vi "SentinelController v38.vi"() -> ()   [LabVIEW 2011]
uses:
  SC MT99XX tester states.ctl
  SC handler states.ctl
  Handler Types.ctl
  SC NS6040 tester states v2.ctl
  <vilib>/Instr/_visa.llb/Select Event Type.ctl
  <userlib>/configTool/configTool.llb/initConfigGlobal.vi
  <userlib>/configTool/configTool.llb/loadConfigFile.vi
  <userlib>/configTool/configTool.llb/closeConfig.vi
  <userlib>/configTool/configTool.llb/getProperty(DBL).vi
  <userlib>/configTool/configTool.llb/getProperty(U32).vi
  <userlib>/configTool/configTool.llb/getProperty(BOOL).vi
  <userlib>/configTool/configTool.llb/getProperty(I32).vi
  <userlib>/configTool/configTool.llb/getProperty(STR).vi
panel:
  out "H2 wt start hidden":u32
  out "H2 wt end hidden":u32
  out "H2 it start hidden":u32
  out "H2 it end hidden":u32
  out "H2 tt start hidden":u32
  out "H2 tt end hidden":u32
  in  "Data log path and filename":path=path "configuraitons/default_configuraiton.cfg"
  in  "Panels":T1(tab)=enum."System Configuration"
  in  "Test cell ID":string="default"
  in  "Operator name":string="default"
  in  "Lot number":string="default"
  in  "Configuration file path and filename":path
  in  "POWER":bool=TRUE
  in  "Tester Handler Config":T2=enum."Seiko-Epson NS6040" caption="Handler type"
  in  "H1 handler type":T2=enum."Seiko-Epson NS6040" caption="Handler type"
  in  "H2 handler type":T2=enum."Seiko-Epson NS6040" caption="Handler type"
  in  "H2 allow lower parallelism":bool
  in  "H1 allow lower parallelism":bool
  in  "H1 low yield warning":dbl=95.0 min=0.0 max=100.0 step=1.0
  in  "Ignore alarms until AFTER this many cycles":i32=20
  in  "H1 low yield alarm":dbl=85.0 min=0.0 max=100.0 step=1.0
  in  "H1 low UPH warning (%)":dbl=95.0 min=1.0 max=48000.0 step=1.0
  in  "H1 low UPH alarm (%)":dbl=90.0 min=1.0 max=48000.0 step=1.0
  in  "Enable data logging of all events":bool=TRUE
  in  "Enable electronic notification of alarms":bool
  in  "H2 low UPH alarm (%)":dbl=90.0 min=1.0 max=48000.0 step=1.0
  in  "H2 low UPH warning (%)":dbl=95.0 min=1.0 max=48000.0 step=1.0
  in  "H2 low yield alarm":dbl=90.0 min=0.0 max=100.0 step=1.0
  in  "H2  low yield warning":dbl=95.0 min=0.0 max=100.0 step=1.0
  in  "H1 enable halt\non yield alarm":bool
  in  "H2 enable halt\non yield alarm":bool
  in  "H1 enable halt\non UPH alarm":bool
  in  "H2 enable halt\non UPH alarm":bool
  out "H2 Device Count":u32 caption="Device Count"
  out "H1 Device Count":u32 caption="Decvice Count"
  out "H1 Good Units":u32 caption="Decvice Count"
  out "H2 Good Units":u32 caption="Device Count"
  out "H1 lot yield mon":dbl format="%.1f"
  out "H2 lot yield mon":dbl format="%.1f"
  out "UPH averaging":u32=20 min=2 max=100 step=1
  out "Yield averaging":u32=20 min=2 max=100 step=1
  in  "Push to reset charts":bool
  in  "Run":bool caption="Run / Stop"
  in  "Optimize handler speed":bool
  out "H1 parallelism":u32
  out "Utilization averaging":i32=6 min=2 max=20 step=1
  out "H2 nominal 2":bool=TRUE
  out "H2 warning 2":bool
  out "H2 alarm 2":bool
  out "H1 nominal 2":bool=TRUE
  out "H1 warning 2":bool
  out "H1 alarm 2":bool
  out "H2 nominal":bool=TRUE
  out "H2 warning":bool
  out "H2 alarm":bool
  out "H1 nominal":bool=TRUE
  out "H1 warning":bool
  out "H1 alarm":bool
  out "H2 Lock":bool
  out "H1 Lock":bool
  out "H2 measured Test Time":dbl caption="Index Time" format="%.2f"
  out "H2 measured  Index Time":dbl caption="Index Time" format="%.2f"
  out "H2 Indexing":bool
  out "H2 Testing":bool
  out "H2 Waiting":bool
  out "H2 On/Off-line":bool
  out "H2 measured Wait Time":dbl caption="Index Time" format="%.2f"
  out "H1 measured Test Time":dbl caption="Index Time" format="%.2f"
  out "H1 measured Index Time":dbl caption="Index Time" format="%.2f"
  out "H1 Indexing":bool
  out "H1 Testing":bool
  out "H1 Waiting":bool
  out "H1 On/Off-line":bool
  out "H1 measured Wait Time":dbl caption="Index Time" format="%.2f"
  out "System UPH":u32(knob) caption="Sys UPH" scale=0.0..30240.0 scale format="%#.0f"
  out "H2 UPH":cluster{u32, u32}(knob) scale=0.0..14400.0 scale format="%#.0f"
  out "H1 UPH":cluster{u32, u32}(knob) scale=0.0..14400.0 scale format="%#.0f"
  out "Sys utilization":dbl(knob) caption="Yield" scale=0.0..100.0
  in  "H2 online":bool=TRUE
  in  "H1 online":bool=TRUE
  in  "Tester online":bool=TRUE
  in  "Alert volume":u32(knob)=5 max=10 step=1 scale=0.0..10.0
  in  "Audio On / Off":bool
  out "SysUtilMon":cluster{i32, i32}(graph)
  out "H2 parallelism":u32 caption="H2 Paralellism"
  out "YieldMon":cluster{i32, i32, i32, i32}(graph)
  out "Program Parallelism":u32=8 caption="Tester Parallelism" min=1 max=16 step=1
  out "H2 calc UPH":dbl format="%#.0f"
  out "H1 Index Time 2":dbl caption="H1 index time"
  out "H1 Test Time 2":dbl caption="H1 test time"
  out "H1 P in formula":u32 caption="H1 Parallelism"
  out "H2 UPH per unit area":dbl format="%.1f"
  out "H1 calc UPH":dbl format="%#.0f"
  out "H1 UPH per unit area":dbl format="%.1f"
  out "Std mo cost ($/mo)":dbl
  out "Std unit cost\n(cents/device)":dbl format="%.3g"
  out "UPH":dbl format="%#.0f"
  in  "Hours per month":i32=730
  out "Std hourly\ncost ($/hr)":dbl format="%.2f"
  in  "Std cell \nfloorspace area":i32=200 min=10 max=1000 step=10
  in  "Overhead ($/mo)":dbl=1000.0 min=0.0 max=10000.0 step=100.0
  in  "Handler cost ($/mo)":dbl=2500.0 min=0.0 max=100000.0 step=100.0
  in  "Tester cost ($/mo)":dbl=8500.0 min=0.0 max=100000.0 step=500.0
  in  "Utilization (%)":u32=80 min=10 max=100 step=10
  out "Calendar days required\nfor testing all units":dbl format="%.1f"
  in  "# of devices to test":u32=10000000 min=1000 max=100000000 step=1000
  out "$ saved":i64 format="%#.0f"
  out "H2 IT (scycle)":dbl format="%.2f"
  out "H2 TT (s/cycle)":dbl format="%.2f"
  out "H2 WT (s/cycle)":dbl format="%.2f"
  out "H1 WT (s/cycle)":dbl format="%.2f"
  out "H1 IT (s/cycle)":dbl format="%.2f"
  out "H1 TT (s/cycle)":dbl format="%.2f"
  out "H2 units/cycle":u32 caption="H1 Parallelism"
  out "H1 units/cycle":u32
  out "Calc H1 UPH":u32
  out "Calc H2 UPH":u32
  out "Std cell floorspace area":i32
  out "Tandem unit cost\n(cents/device)":dbl format="%.3f"
  out "Hours per month 2":i32 caption="Hours per month"
  out "Total Mo Costs ($/mo) 3":dbl caption="Tandem mo cost ($/mo)"
  out "Total Mo Costs ($/mo) 2":dbl caption="Std mo cost ($/mo)"
  out "Calc\nsystem UPH":u32 caption="Simulated\nSystem UPH"
  out "Tandem\nfloorspace area":i32
  out "Tandem UPH\nper unit area":dbl format="%.1f"
  in  "Second handler cost ($/mo)":dbl=2500.0 min=0.0 max=10000.0 step=100.0
  out "Tandem hourly\ncost ($/hr)":dbl format="%.2f"
  in  "Celerint licensing cost ($/mo)":dbl=1000.0 min=0.0 max=10000.0 step=100.0
  in  "Celerint hardware cost ($/mo)":dbl min=0.0 max=10000.0 step=1.0
  in  "Additional floorspace\nfor second handler":i32=50 min=0 max=1000 step=10
  out "Number of text alerts":u32 caption="Number of alerts\nsent as notifications"
  in  "Enable text notification":bool
  out "Notifications Lot Display":string="default" caption="Lot number (not editable)"
  in  "Include\ndata log as\nattachment":bool=TRUE
  out "Number of email alerts":u32 caption="Number of alerts\nsent as notifications"
  out "Email alert - attachment (not editable)":path
  in  "Email alert - message":string="An alarm event has ocurred on a semiconductor test lot that you have requested to monitor.  Please see the attached data log for event details.\n\nThis message is generated automatically by the Sentinel Controller program.\n\nTo stop these messages, please contact the test floor operator and disable automatic alert notifictions.\n\n"
  in  "Email alert - engineer":string="harry@celerint.com"
  in  "Email alert - CC":string="hjr@celerint.com"
  in  "Enable email notification":bool
  in  "Carrier":enum16{"T-Mobile", "AT&T", "Verizon", "Sprint"}(ring)=enum."AT&T"
  in  "Phone number":string="5128263411"
  in  "Subject":string="From: Sentinel Controller"
  in  "Body":string="An alarm event has ocurred"
  in  "GPIB wait time (ms)":u32=1000
  in  "Slow for  Diagnostics":bool=TRUE
  out "GPIB bus 0 read error":bool
  out "GPIB Bus 0 traffic":string
  out "GPIB bus 1 traffic":string
  out "GPIB bus 2 traffic":string
  out "GPIB bus 0 write error":bool
  out "GPIB bus 1 read error":bool
  out "GPIB bus 1 write error":bool
  out "GPIB bus 2 write error":bool
  out "GPIB bus 2 read error":bool
  out "VISA bus 1 open error":bool
  out "VISA bus 2 open error":bool
  out "VISA bus 0 open error":bool
  out "VISA bus 0 close error":bool
  out "VISA bus 1 close error":bool
  out "VISA bus 2 close error":bool
  out "Decrease Handler Velocity":string
  out "Increase Handler Velocity":string
  out "Get Handler Velocity":string
  in  "SentCtrl listens to tester at":refnum<visa-resource-name>="GPIB0::INTFC"
  out "H2 Address":string
  out "H1 Address":string
  out "Tester address":string
  in  "SentCtrl talks to tester at":refnum<visa-resource-name>="GPIB0::0::INSTR"
  in  "SentCtrl listens to handler 1 at":refnum<visa-resource-name>="GPIB1::INTFC"
  in  "SentCtrl talks to handler 1 at":refnum<visa-resource-name>="GPIB1::1::INSTR"
  in  "SentCtrl listens to handler 2 at":refnum<visa-resource-name>="GPIB2::INTFC"
  in  "SentCtrl talks to handler 2 at":refnum<visa-resource-name>="GPIB2::1::INSTR"
  in  "Ni Logo":bool
  in  "Ni Logo 2":bool
  in  "H2 Ready with sites hid":bool
  in  "SRQ MASK from tester hid":string
  in  "H1 binning string hid":string
  in  "H2 binning string hid":string
  in  "H1 FULLSITES? response hid":string
  in  "H2 FULLSITES? response hid":string
  in  "H1 FULLSITES? binary hid":string
  in  "H2 FULLSITES? binary hid":string
  in  "H1 response to SPOLL hid":string
  in  "H2 response to SPOLL hid":string
  in  "H1 response to FR? hid":string
  in  "H2 response to FR? hid":string
  in  "NS6040 tester states H1 hid":T3
  in  "NS6040 tester states H2 hid":T3
  in  "MT99XX tester states H2 hid":T4
  in  "MT99XX tester states H1 hid":T4
  in  "GPIB parsed msg from tester hid":string
  in  "Message from H2 hid":string
  in  "Message from H1 hid":string
  in  "Message from tester hid":string
  in  "H1 response to *IDN? hid":string
  in  "H2 response to *IDN? hid":string
  in  "GPIB wait timeout hid":u32
  out "Number of data log entries hid":u32
  in  "Last locked handler hid":enum16{"H1", "H2"}(ring)
  out "SC measured wait time hid":dbl
  out "Exit SC tester H2 StMach hid":bool
  out "Exit SC tester H1 StMach hid":bool
  out "Exit SC handler StMach hid":bool
  out "H2 response to *HAND? hid":string
  out "H1 response to *HAND? hid":string
  in  "Tester loop counter hid":u32
  in  "H2 loop counter hid":u32
  in  "H1 loop counter hid":u32
  in  "Test Cycle State hid":T5(ring)
  in  "Test time expected hid":dbl
  out "H1 it end hidden":u32
  out "H1 wt start hidden":u32
  out "H1 tt start hidden":u32
  out "H1 wt end hidden":u32
  out "H1 tt end hidden":u32
  out "H1 it start hidden":u32
  in  "H1 SITES? response hid":string
  out "VISA bus 1 resource name out hid":refnum<visa-resource-name>
  out "VISA bus 1 error out hid":errorcluster
  out "VISA bus 2 error out hid":errorcluster
  out "VISA bus 2 resource name out hid":refnum<visa-resource-name>
  out "VISA bus 0 error out hid":errorcluster
  out "tester wt start hid":u32
  out "tester wt end hid":u32
  out "tester tt start hid":u32
  out "tester tt end hid":u32
  out "SC measured test time hid":dbl
  in  "Binning string from tester hid":string
  out "VISA bus 0 resource name out hid":refnum<visa-resource-name>
  in  "SC handler states hid":T6
  out "H1 Single Handler UPH hid":dbl
  out "H1 UPH warning limit hid":dbl
  out "H1 UPH alarm limit hid":dbl
  out "H2 Single Handler UPH hid":dbl
  out "H2 UPH warning limit hid":dbl
  out "H2 UPH alarm limit hid":dbl
  in  "Min Test Time hid":dbl=0.499 caption="Min Test Time" min=0.1 max=1.0 step=0.1 format="%#.1g"
  in  "H2 index time expected hid":dbl
  in  "H1 index time expected hid":dbl
  in  "system states hid":T7(ring)
  in  "system statuts hid":T8(ring)
  out "H1 cycle yield hid":dbl format="%.1f"
  out "H2 cycle yield hid":dbl format="%.1f"
  in  "H2 SITES? response hid":string
  in  "H1 Ready with sites hid":bool
  # "Sentinel Controller\nfor\nTandlem Handler\nTest Cells \nwww.celerint.com"
  # "Turning off POWER will stop execution the Sentinel Controller Program"
  # "INPUT FILE"
  # "LOT INFORMATION"
  # "Celerint Sentinel Controller"
  # "SYSTEM SETTINGS"
  # "Tester Handler Config"
  # "Handler  1"
  # "Handler 2"
  # "Set UPH thresholds as % of max UPH"
  # "Set UPH thresholds as % of max UPH"
  # "test cycles (insertions)"
  # "Celerint Sentinel Controller"
  # "Handler 2"
  # "Handler 1"
  # "Yield"
  # "UPH"
  # "Yield"
  # "UPH"
  # "parallelism"
  # "lot yield (%)"
  # "good devices"
  # "devices tested"
  # "Data"
  # "Avg"
  # "wait time"
  # "index time"
  # "test time"
  # "waiting"
  # "H1"
  # "H2"
  # "testing"
  # "indexing"
  # "on/off-line"
  # "STANDARD SETUP"
  # "H2 calculated\nsimilarly"
  # "3600"
  # "Celerint Sentinel\nController Simulator"
  # "TANDEM HANDLER SETUP"
  # "SAVINGS"
  # "3600 (s/hr)"
  # "3600 (s/hr)"
  # "Celerint Sentinel Controller"
  # "Lot number will be appended automatically:"
  # "This data is read from the INI file (.cfg)\nat program start and is used to configure\nthe various GPIB interfaces on the Sentinel\nController."
  # "These setting are created based on the addresses read from the INI file."
  # "Laptop Tester Sim\nGPIB0,SC\naddress 0\nlisten at: GPIB0::INTFC\ntalk to: GPIB0::1::INSTR"
  # "*SITES?"
  # "binning"
  # "Bus 0"
  # "1011"
  # "SC\nGPIB0,Non-SC\naddress 1\nlisten at: GPIB0::INTFC\ntalk to: GPIB0::0::INSTR"
  # "SC\nGPIB1,SC\naddress 0\nlisten at: GPIB1::INTFC\ntalk to: GPIB1::0::INSTR"
  # "SC\nGPIB2,SC\naddress 0\nlisten at: GPIB2::INTFC\ntalk to: GPIB2::0::INSTR"
  # "NI PXI-1031"
  # "*SITES?"
  # "binning"
  # "*SITES?"
  # "binning"
  # "Bus 1"
  # "Bus 2"
  # "1011"
  # "1011"
  # "Laptop H1 Sim\nGPIB1,Non-SC\naddress 1\nlisten at: GPIB1::INTFC\ntalk to: GPIB1::0::INSTR"
  # "Laptop H2 Sim\nGPIB2,Non-SC\naddress 1\nlisten at: GPIB2::INTFC\ntalk to: GPIB2::0::INSTR"
  # "Note:\nUsually, there are default GPIB addresses used for the tester and handler.\nThese addresses are read in from the INI file (.cfrg extension) when this\nprogram initializes.  For the purposes of this map, we are using  these defaults:\n          - Semiconductor tester default GPIB address: 6\n          - Semiconductor handler default GPIB address: 14\nFor the purposes of this illustration, these addresses are purely arbitrary."
  # "Tester\nGPIB0,SC\naddress 6\nlisten at: GPIB0::INTFC\ntalk to: GPIB0:14::INSTR"
  # "*SITES?"
  # "binning"
  # "Bus 0"
  # "1011"
  # "SC\nGPIB0,Non-SC\naddress 14\nlisten at: GPIB1::INTFC\ntalk to: GPIB1:6::INSTR"
  # "SC\nGPIB1,SC\naddress 6\nlisten at: GPIB1::INTFC\ntalk to: GPIB1:14::INSTR"
  # "SC\nGPIB2,SC\naddress 6\nlisten at: GPIB2::INTFC\ntalk to: GPIB2:14::INSTR"
  # "NI PXI-1031"
  # "*SITES?"
  # "binning"
  # "*SITES?"
  # "binning"
  # "Bus 1"
  # "Bus 2"
  # "1011"
  # "1011"
  # "Handler 1\nGPIB0,Non-SC\naddress 14\nlisten at: GPIB0::INTFC\ntalk to: GPIB0:6::INSTR"
  # "Handler 2\nGPIB0,Non-SC\naddress 14\nlisten at: GPIB0::INTFC\ntalk to: GPIB0:6::INSTR"
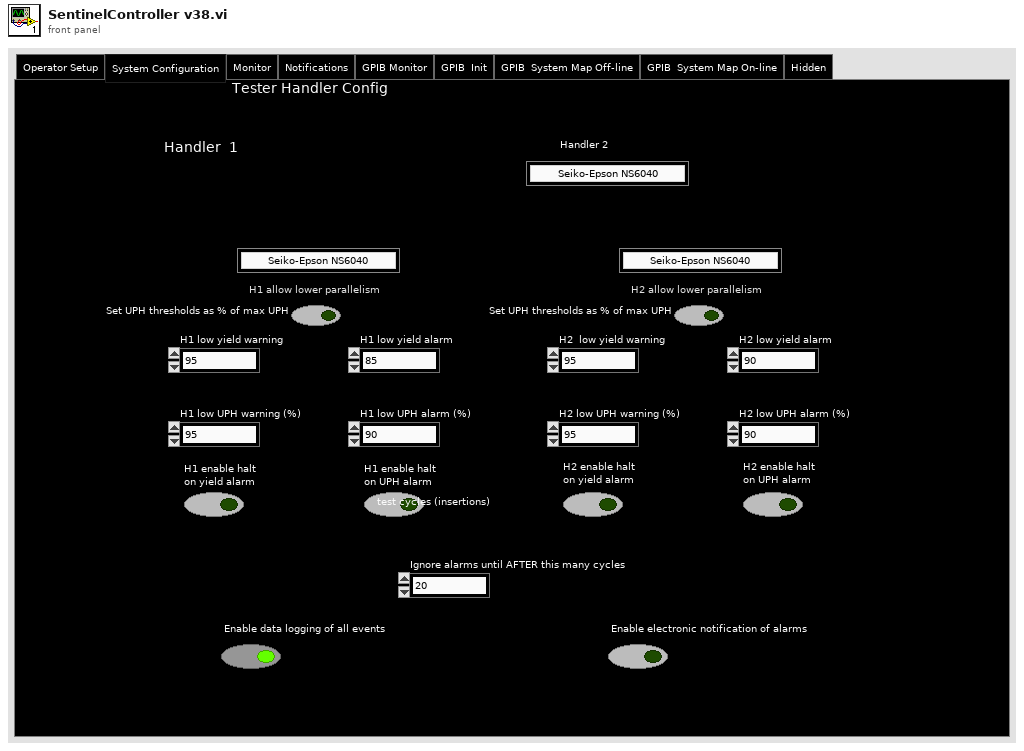
[diagram p1: front panel]
types:
  T1 = enum32{"Operator Setup", "System Configuration", "Monitor", "Benefit Analysis", "Notifications", "GPIB Monitor", "GPIB  Init", "GPIB  System Map Off-line", "GPIB  System Map On-line", "Hidden"}
  T2 = typedef "Handler Types.ctl" = enum16{"Multitest", "Seiko-Epson NS6040"}
  T3 = typedef "SC NS6040 tester states v2.ctl" = enum16{"initializing bus", "sending *IDN?", "serial polling handler", "sending Fullsites?", "testing", "binning", "closing bus"}
  T4 = typedef "SC MT99XX tester states.ctl" = enum16{"initializing bus", "polling *SITES?", "sending *IDN?", "testing", "binning", "closing bus"}
  T5 = enum16{"idled", "SOT received", "SOT sent", "binning sent", "binning received", "sites ready received", "sites ready sent"}
  T6 = typedef "SC handler states.ctl" = enum16{"initializing bus", "waiting on event", "waiting on serial poll", "reading", "responding to *IDN?", "responding to Fullsites?", "responding to SITES?", "responding to HIDN?", "respond to HAND?", "testing", "responding to BINON", "responding to A BIN", "ECHONG", "ECHOOK", "responding to unknown command", "closing bus"}
  T7 = enum16{"H1 Ready", "H2 Ready", "No Handler Ready"}
  T8 = enum16{"H1NH2N", "H1NH2W", "H1NH2A", "H1WH2N", "H1WH2W", "H1WH2A", "H1AH2N", "H1AH2W", "H1AH2A"}
  T9 = enum16{"open", "replace", "create", "open or create", "replace or create", "replace or create with confirmation"}
  T10 = typedef "configRef.ctl" = refnum<vi>
  T11 = cluster{i32, "rolling avg out":dbl, "H1 low yield alarm":dbl, "H2 low yield alarm":dbl}
  T12 = cluster{"rolling avg out":dbl, i32, "H1 low yield alarm":dbl, "H2 low yield alarm":dbl}
  T13 = typedef "Select Event Type.ctl" = u32
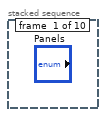
[diagram p2: hidden frame]
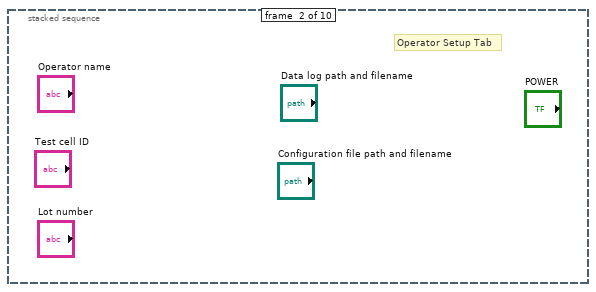
[diagram p3: hidden frame]
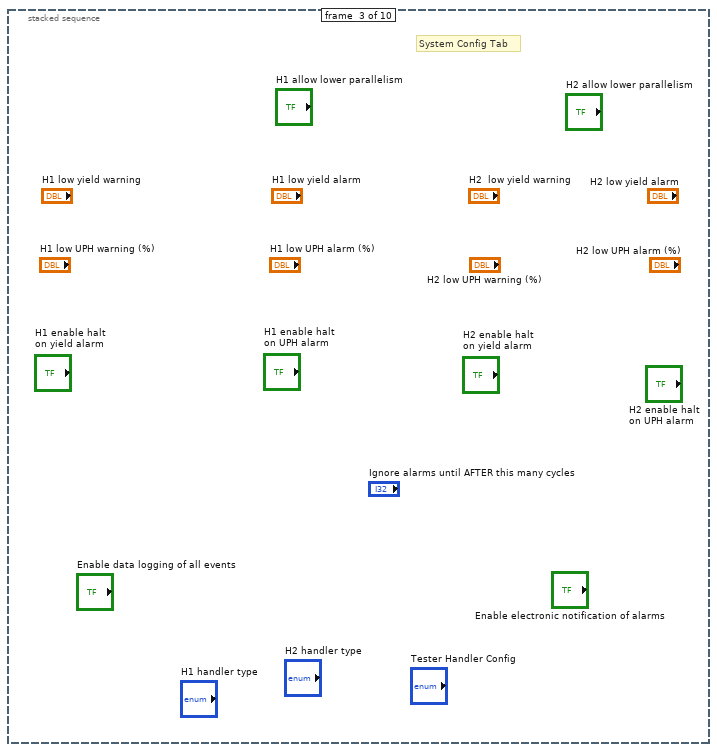
[diagram p4: hidden frame]
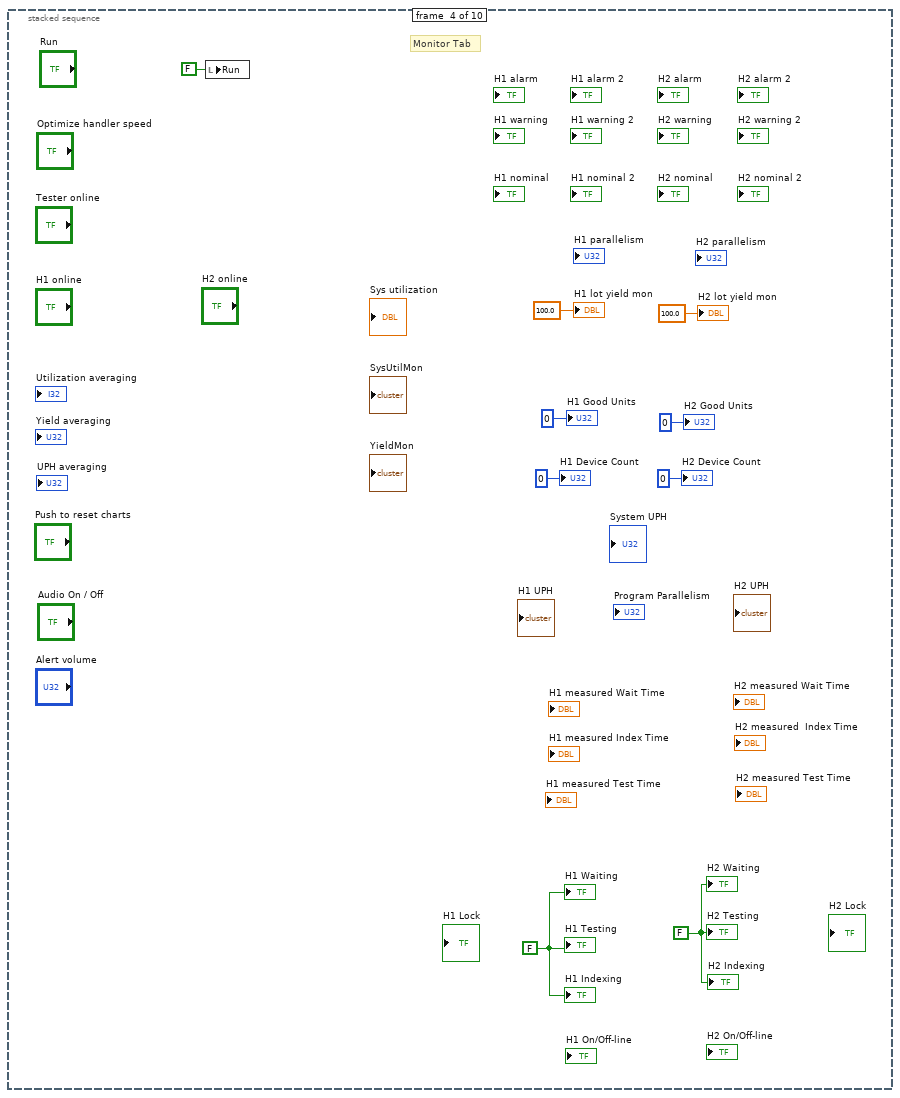
[diagram p5: hidden frame]
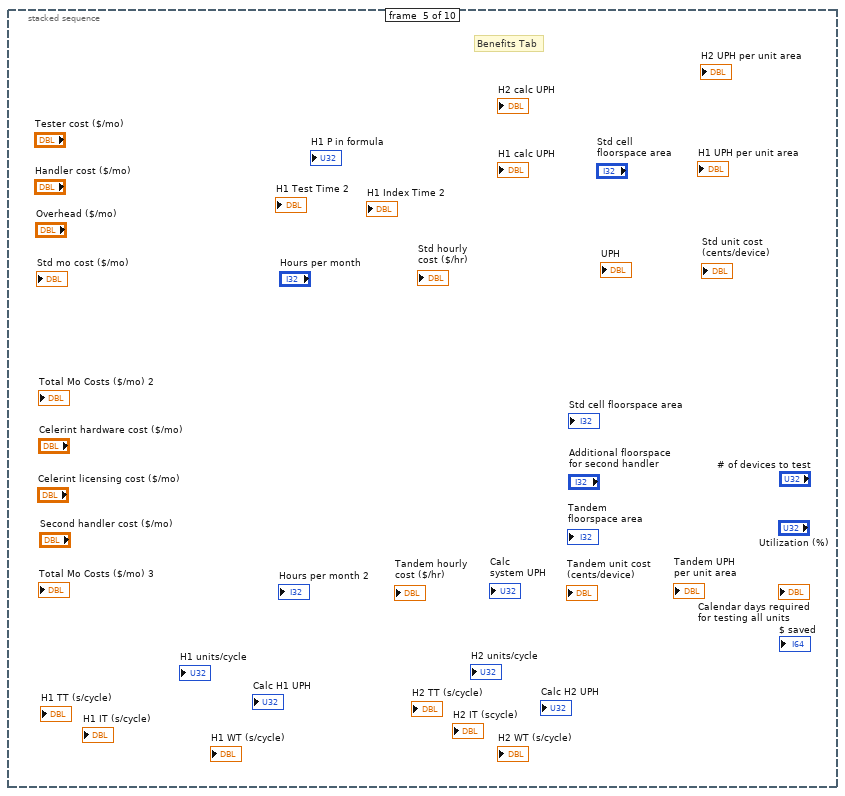
[diagram p6: hidden frame]
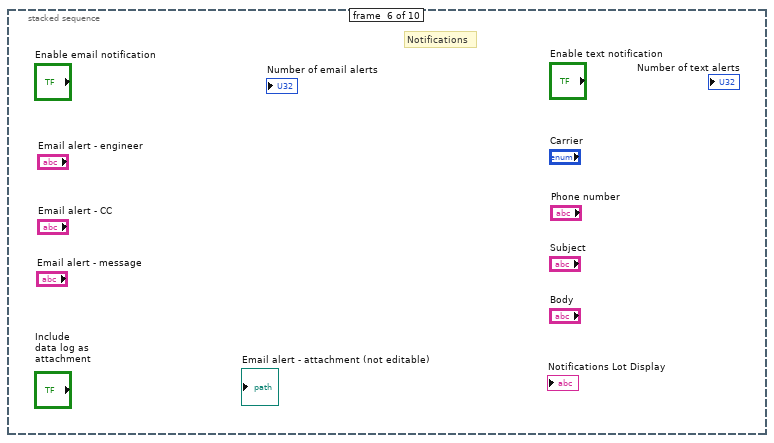
[diagram p7: hidden frame]
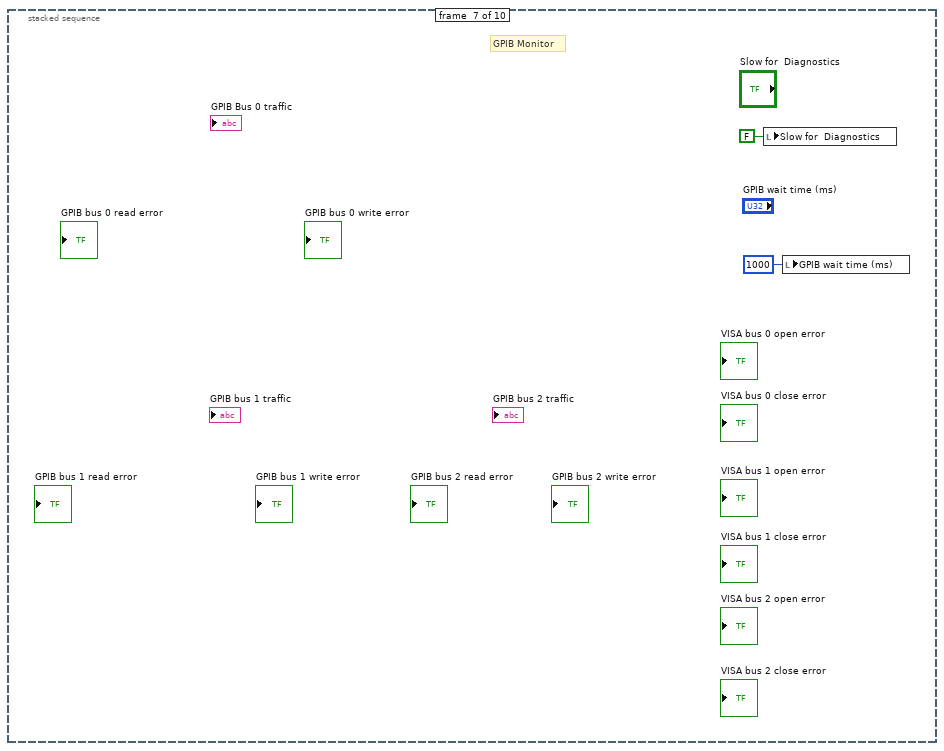
[diagram p8: hidden frame]
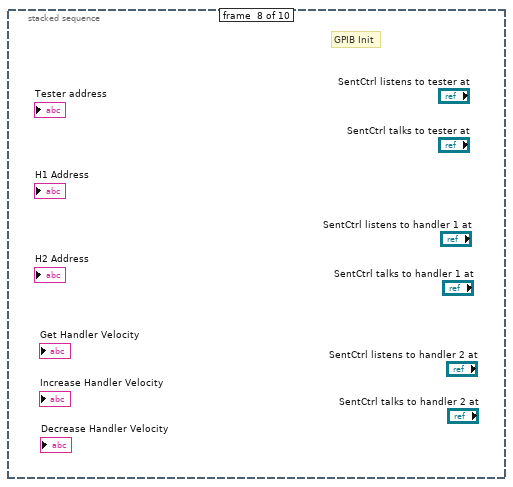
[diagram p9: hidden frame]
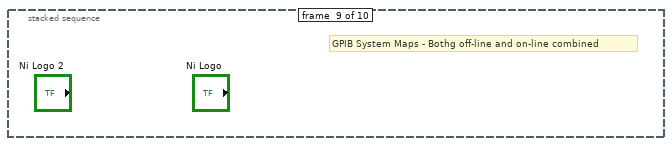
[diagram p10: hidden frame]
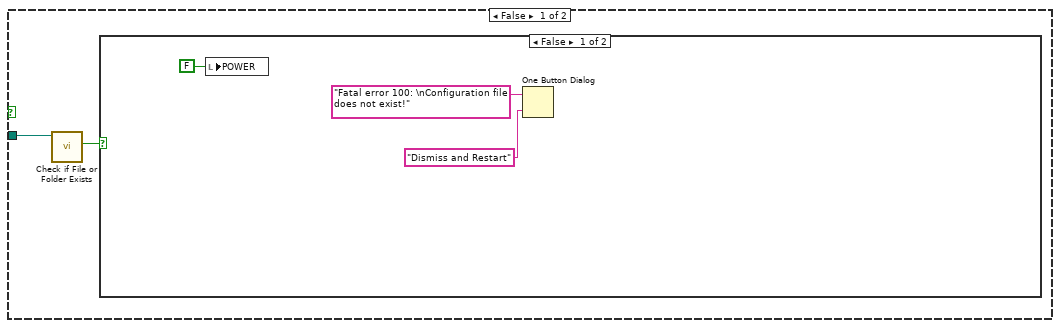
[diagram p11: hidden frame]
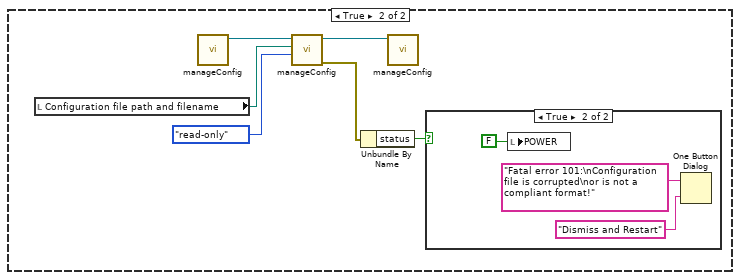
[diagram p12: hidden frame]
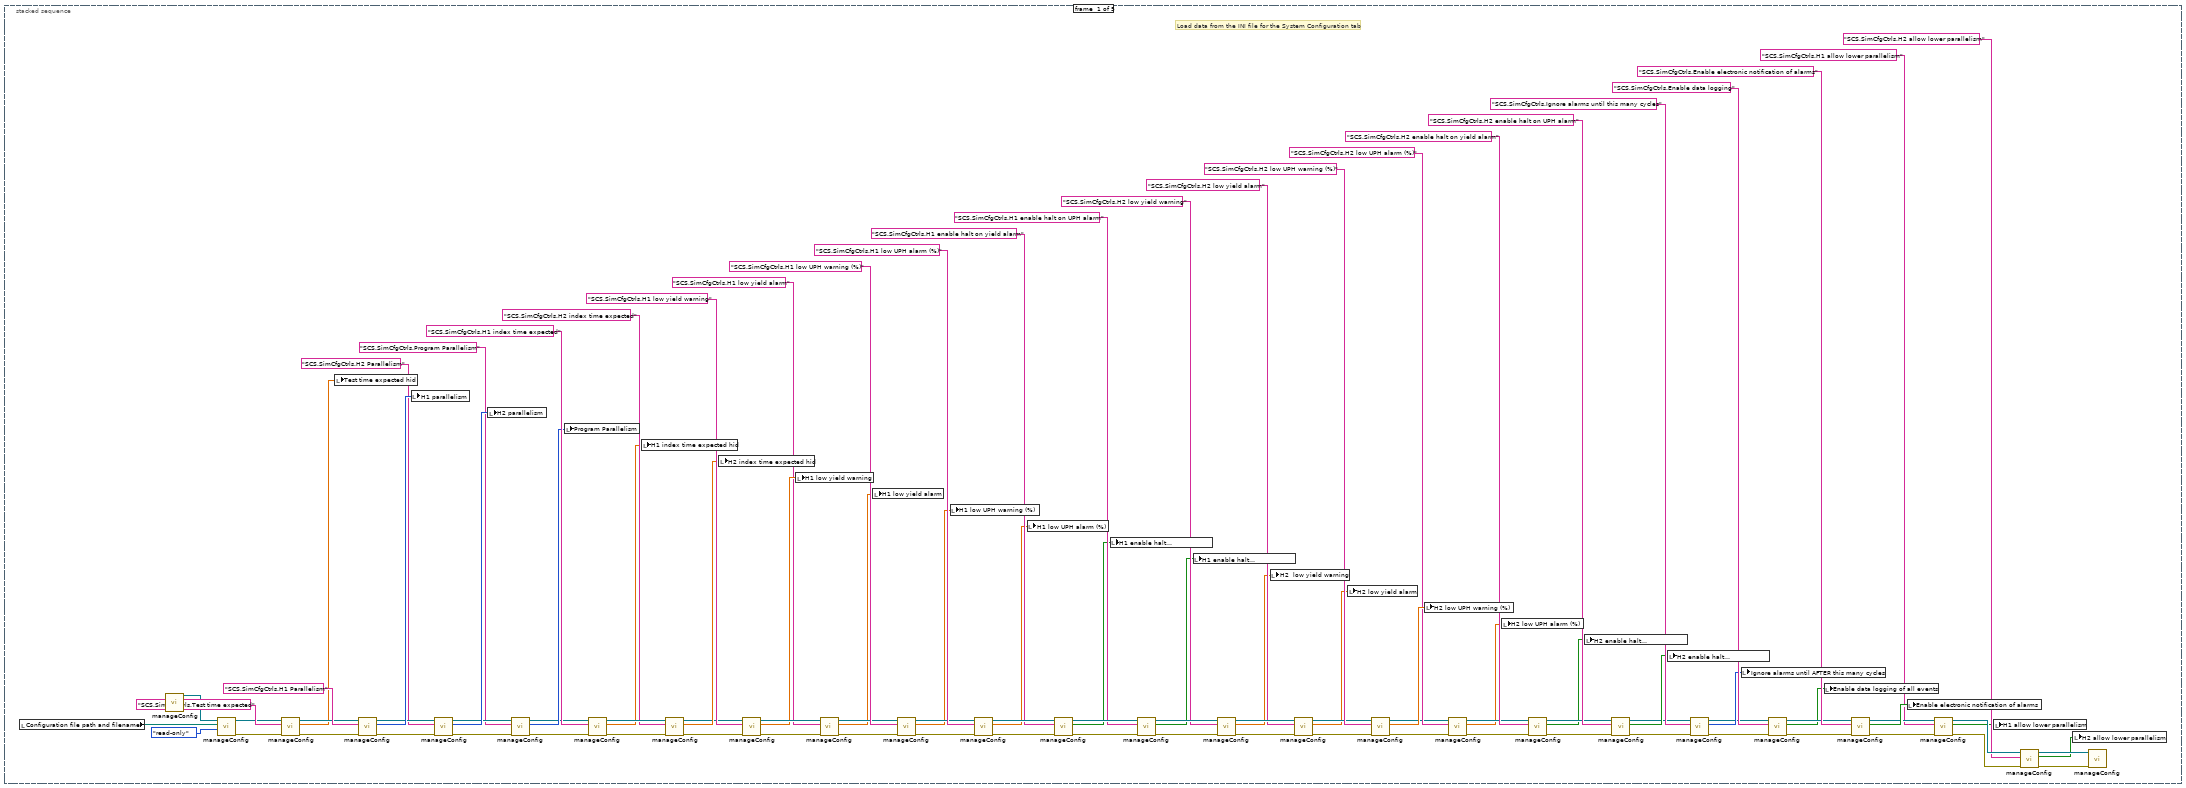
[diagram p15: hidden frame]
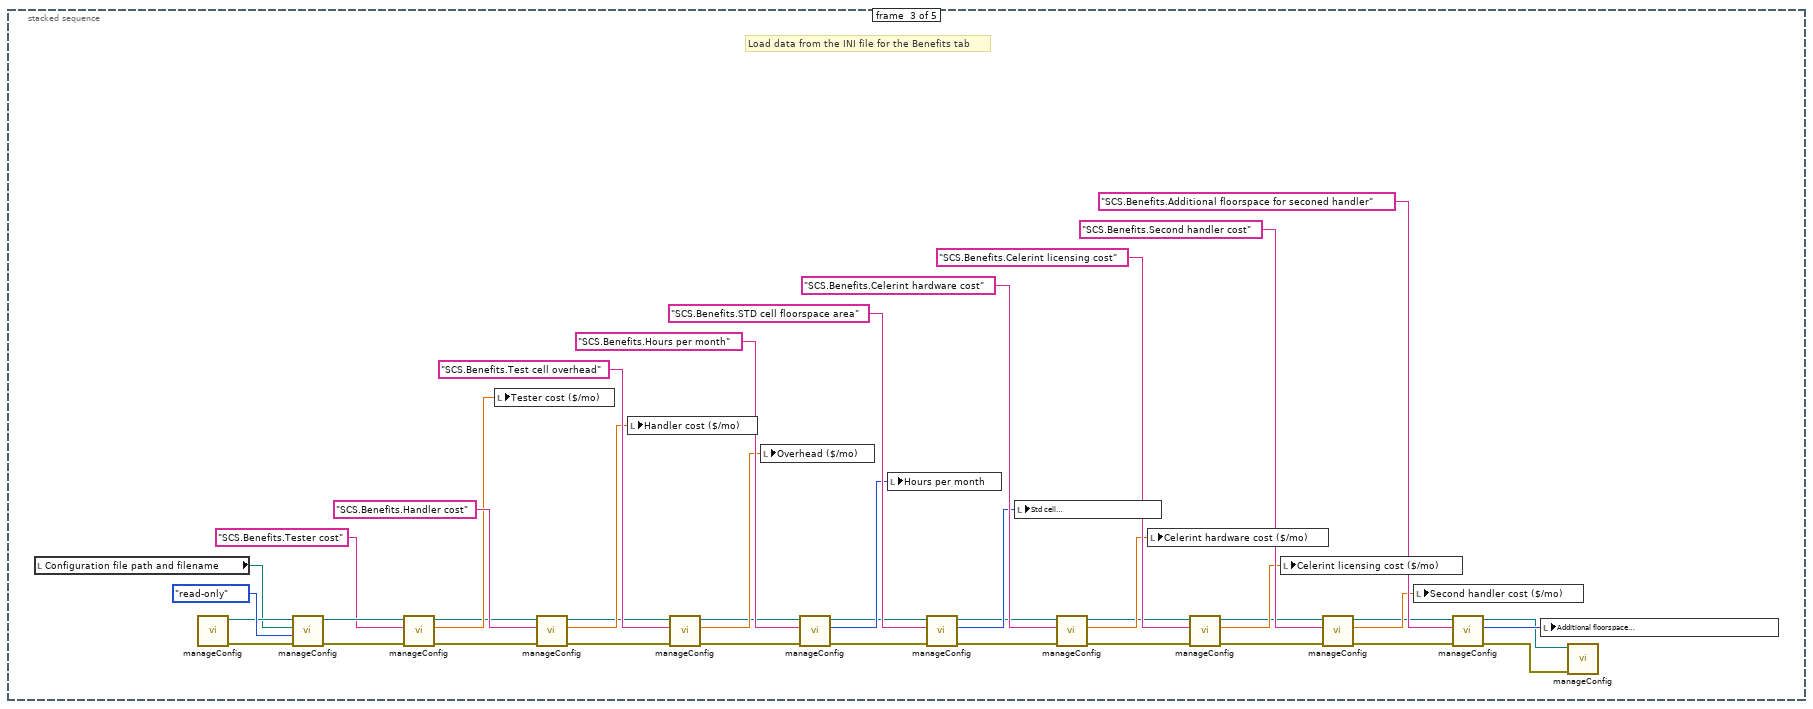
[diagram p16: hidden frame]
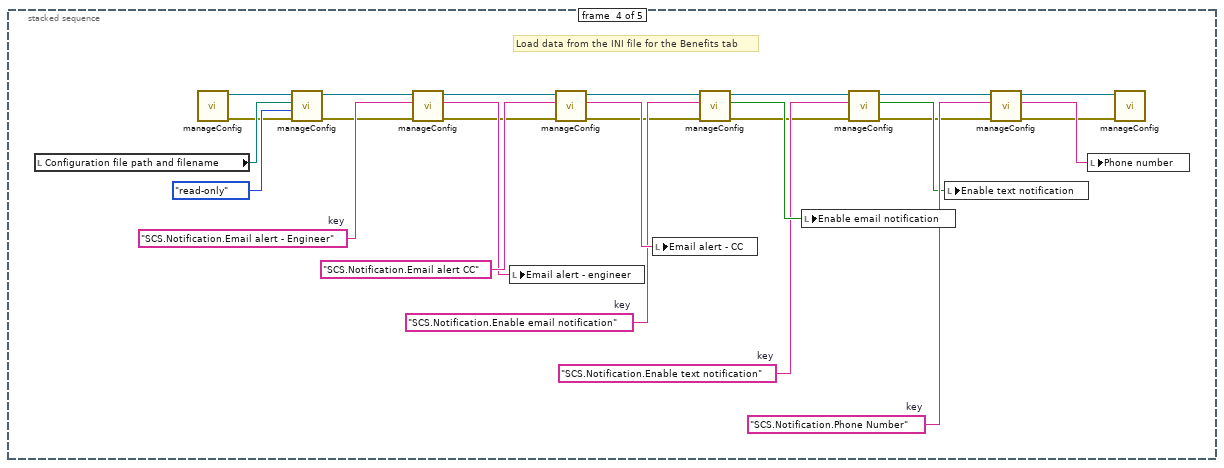
[diagram p17: hidden frame]
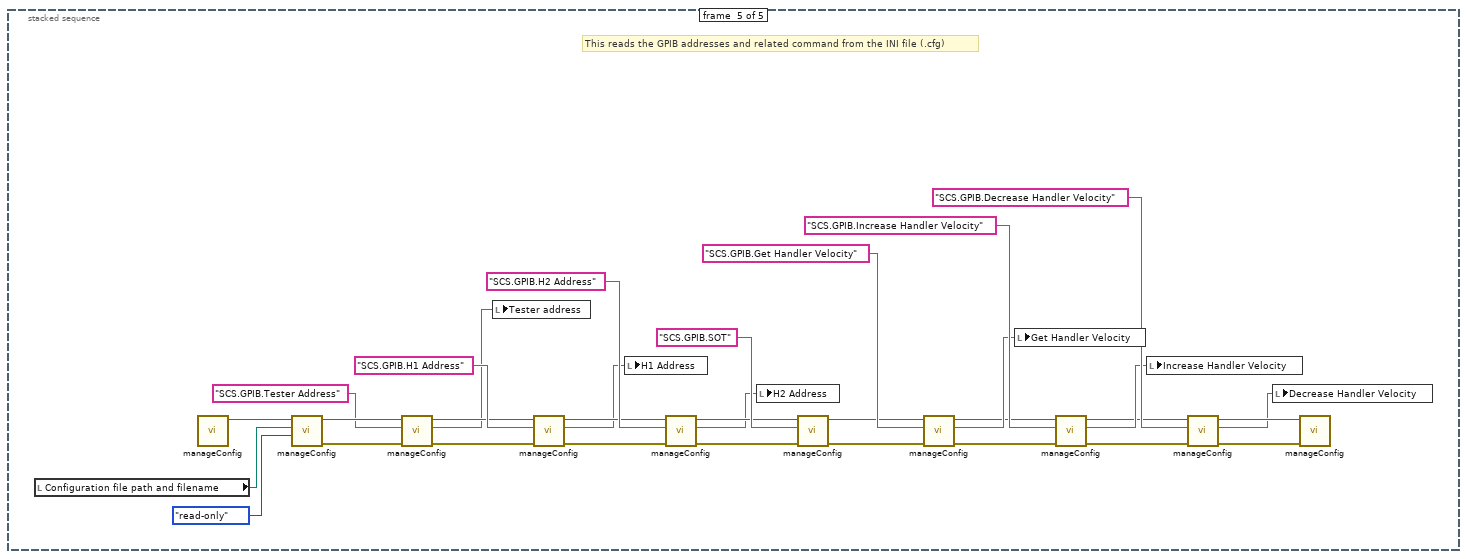
[diagram p18: hidden frame]
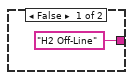
[diagram p20: hidden frame]
diagram:
  n1 = flat-sequence {
    frame #0 {
      # "This frame contains ALL declarations for control and indicators.\nAll hidden objects are on frame #9.  On the front panel, these hidden\nobjects are located on a tab that is hidden."
      n2 = stacked-sequence {
        frame #0 {
        }
        frame #1 {
          # "Operator Setup Tab"
        }
        frame #2 {
          # "System Config Tab"
        }
        frame #3 {
          w2 = FALSE ("H2 Testing")
          w1 = FALSE ("H1 Testing")
          # "Monitor Tab"
          n3 = local write "Run"(FALSE ("Run")) -> ()
          "H1 Testing" <- w1
          "H1 Waiting" <- w1
          "H1 Indexing" <- w1
          "H2 Testing" <- w2
          "H2 Waiting" <- w2
          "H2 Indexing" <- w2
          "H2 Good Units" <- 0
          "H2 Device Count" <- 0
          "H2 lot yield mon" <- 100.0 ("H2 Yield  Mon")
          "H1 lot yield mon" <- 100.0 ("H1 Yield Mon")
          "H1 Good Units" <- u32 0
          "H1 Device Count" <- u32 0
        }
        frame #4 {
          # "Benefits Tab"
        }
        frame #5 {
          # "Notifications"
        }
        frame #6 {
          # "GPIB Monitor"
          n4 = local write "Slow for  Diagnostics"(FALSE ("Slow for  Diagnostics")) -> ()
          n5 = local write "GPIB wait time (ms)"(u32 1000 ("GPIB wait time (ms)")) -> ()
        }
        frame #7 {
          # "GPIB Init"
        }
        frame #8 {
          # "GPIB System Maps - Bothg off-line and on-line combined"
        }
        frame #9 {
          (unwired) 0.031 ("tester measured wait time")
          # "Hidden controls and indicators"
          n6 = local write "Last locked handler hid"(enum16{"H1", "H2"}."H1" ("Last locked handler")) -> ()
          "SC measured test time hid" <- 1.0 ("tester measured test time")
          "H1 response to *HAND? hid" <- "" ("H1 response to *HAND? hidden")
          "H2 response to *HAND? hid" <- "" ("H2 response to *HAND? hidden")
          "Exit SC handler StMach hid" <- FALSE ("Exit tester state machine")
          "Exit SC tester H1 StMach hid" <- FALSE ("Exit H1 state machine")
          "Exit SC tester H2 StMach hid" <- FALSE ("Exit H2 state machine")
          "SC measured wait time hid" <- 1.0 ("tester measured wait time hid")
          "H2 cycle yield hid" <- 100.0 ("H2 Yield  Mon")
          "H1 cycle yield hid" <- 100.0 ("H1 Yield Mon")
        }
      }
    }
    frame #1 {
      n7 = local write "POWER"(TRUE ("POWER")) -> ()
    }
    frame #2 {
      # "This frame handles verifying that the configuration file exists and is valaid.\nIt also creates the data log."
      n8 = local read "Configuration file path and filename"() -> (w25:path)
      n9 = call <vilib>:"Application Directory.vi"() -> ("Application Directory"=w27:path)
      n10 = Equal?(x=w25, y=path "") -> (x = y?=w24:bool)
      n11 = Get Date/Time String(want seconds? (F)=TRUE) -> (date string=w40:string, time string=w32:string)  [unwired: 2 in]
      n12 = Build Path(base path=w27, name or relative path="datalogs") -> (appended path=w45:path)
      n13 = Path To String(path=w45) -> (string=w36:string)
      n14 = Search and Replace String(replace all?=TRUE ("replace all? (F)"), input string=w40, search string="/", replace string="-" ("replace string (\"\")")) -> (result string=w30:string)  [unwired: 4 in, 3 out]
      n15 = Search and Replace String(replace all?=TRUE ("replace all? (F)"), input string=w32, search string=":", replace string="." ("replace string (\"\")")) -> (result string=w31:string)  [unwired: 4 in, 3 out]
      n16 = case shown="True" w24 {
        tunnel: w25 -> [w47 _]
        frame False {
          n17 = call <vilib>:"Check if File or Folder Exists.vi"("path"=w47) -> ("file or folder exists?"=w46:bool)  [unwired: 8 in, 2 out]
          n18 = case shown="False" w46 {
            frame False {
              n19 = local write "POWER"(FALSE ("POWER")) -> ()
              n20 = One Button Dialog(message="Fatal error 100: \nConfiguration file does not exist!", button name ("OK")="Dismiss and Restart") -> ()  [unwired: 1 out]
            }
            frame True {
              n21 = local read "Configuration file path and filename"() -> (w54:path)
              n22 = call-poly <userlib>:"manageConfig.vi"() -> ("config ref out"=w55:T10)  [unwired: 10 in, 1 out]
              n23 = call-poly <userlib>:"manageConfig.vi"("access (0:read/write)"=enum16{"read/write", "read-only", "write-only"}."read-only", "config file path"=w54, "config ref"=w55) -> ("error out"=w53:errorcluster, "config ref out"=w51:T10)  [unwired: 6 in, 1 out]
              n24 = Unbundle By Name(w53) -> ("status"=w52:bool)
              n25 = call-poly <userlib>:"manageConfig.vi"("config ref"=w51) -> ()  [unwired: 10 in, 1 out]
              n26 = case shown="True" w52 {
                frame False {
                }
                frame True {
                  n27 = local write "POWER"(FALSE ("POWER")) -> ()
                  n28 = One Button Dialog(message="Fatal error 101:\nConfiguration file is corrupted\nor is not a compliant format!", button name ("OK")="Dismiss and Restart") -> ()  [unwired: 1 out]
                }
              }
            }
          }
        }
        frame True {
          n29 = call <vilib>:"Application Directory.vi"() -> ("Application Directory"=w63:path)
          n30 = Build Path(base path=w63, name or relative path="configurations") -> (appended path=w60:path)
          n31 = Path To String(path=w60) -> (string=w65:string)
          n32 = Concatenate Strings(w65, "\\" ("string"), "default_configuration.cfg" ("string")) -> (w66:string)
          n33 = String To Path(string=w66) -> (path=w67:path)
          n34 = local write "Configuration file path and filename"(w67) -> ()
        }
      }
      n35 = Concatenate Strings(w36, "\\" ("string"), w30, " " ("string"), w31, ".txt" ("string")) -> (w42:string)
      n36 = String To Path(string=w42) -> (path=w44:path)
      n37 = local write "Data log path and filename"(w44) -> ()
    }
    frame #3 {
      # "This frame reads the INI file and initializes all data that is under engineering control."
      n38 = local read "POWER"() -> (w68:bool)
      n39 = case shown="True" w68 {
        frame False {
        }
        frame True {
          n40 = stacked-sequence {
            frame #0 {
              # "Load data from the INI file for the System Configuration tab"
              n41 = local read "Configuration file path and filename"() -> (w162:path)
              n42 = call-poly <userlib>:"manageConfig.vi"() -> ("config ref out"=w163:T10)  [unwired: 10 in, 1 out]
              n43 = call-poly <userlib>:"manageConfig.vi"("access (0:read/write)"=enum16{"read/write", "read-only", "write-only"}."read-only", "config file path"=w162, "config ref"=w163) -> ("error out"=w101:errorcluster, "config ref out"=w100:T10)  [unwired: 6 in, 1 out]
              n44 = call-poly <userlib>:"manageConfig.vi"("error in"=w101, "property path"="SCS.SimCfgCtrls.Test time expected" ("key"), "config ref"=w100) -> ("error out"=w97:errorcluster, "data"=w103:dbl, "config ref out"=w104:T10)  [unwired: 5 in, 1 out]
              n45 = local write "Test time expected hid"(w103) -> ()
              n46 = call-poly <userlib>:"manageConfig.vi"("error in"=w97, "property path"="SCS.SimCfgCtrls.H1 Parallelism", "config ref"=w104) -> ("error out"=w96:errorcluster, "value"=w116:u32, "config ref out"=w110:T10)  [unwired: 5 in, 1 out]
              n47 = local write "H1 parallelism"(w116) -> ()
              n48 = call-poly <userlib>:"manageConfig.vi"("error in"=w96, "property path"="SCS.SimCfgCtrls.H2 Parallelism", "config ref"=w110) -> ("error out"=w95:errorcluster, "value"=w112:u32, "config ref out"=w109:T10)  [unwired: 5 in, 1 out]
              n49 = local write "H2 parallelism"(w112) -> ()
              n50 = call-poly <userlib>:"manageConfig.vi"("error in"=w95, "property path"="SCS.SimCfgCtrls.Program Parallelism", "config ref"=w109) -> ("error out"=w94:errorcluster, "value"=w111:u32, "config ref out"=w102:T10)  [unwired: 5 in, 1 out]
              n51 = local write "Program Parallelism"(w111) -> ()
              n52 = call-poly <userlib>:"manageConfig.vi"("error in"=w94, "property path"="SCS.SimCfgCtrls.H1 index time expected", "config ref"=w102) -> ("error out"=w93:errorcluster, "data"=w106:dbl, "config ref out"=w115:T10)  [unwired: 5 in, 1 out]
              n53 = local write "H1 index time expected hid"(w106) -> ()
              n54 = call-poly <userlib>:"manageConfig.vi"("error in"=w93, "property path"="SCS.SimCfgCtrls.H2 index time expected", "config ref"=w115) -> ("error out"=w99:errorcluster, "data"=w105:dbl, "config ref out"=w98:T10)  [unwired: 5 in, 1 out]
              n55 = local write "H2 index time expected hid"(w105) -> ()
              n56 = call-poly <userlib>:"manageConfig.vi"("error in"=w99, "property path"="SCS.SimCfgCtrls.H1 low yield warning" ("key"), "config ref"=w98) -> ("error out"=w92:errorcluster, "data"=w139:dbl, "config ref out"=w149:T10)  [unwired: 5 in, 1 out]
              n57 = local write "H1 low yield warning"(w139) -> ()
              n58 = call-poly <userlib>:"manageConfig.vi"("error in"=w92, "property path"="SCS.SimCfgCtrls.H1 low yield alarm", "config ref"=w149) -> ("error out"=w91:errorcluster, "data"=w138:dbl, "config ref out"=w148:T10)  [unwired: 5 in, 1 out]
              n59 = local write "H1 low yield alarm"(w138) -> ()
              n60 = call-poly <userlib>:"manageConfig.vi"("error in"=w91, "property path"="SCS.SimCfgCtrls.H1 low UPH warning (%)", "config ref"=w148) -> ("error out"=w90:errorcluster, "data"=w137:dbl, "config ref out"=w150:T10)  [unwired: 5 in, 1 out]
              n61 = local write "H1 low UPH warning (%)"(w137) -> ()
              n62 = call-poly <userlib>:"manageConfig.vi"("error in"=w90, "property path"="SCS.SimCfgCtrls.H1 low UPH alarm (%)", "config ref"=w150) -> ("error out"=w89:errorcluster, "data"=w136:dbl, "config ref out"=w151:T10)  [unwired: 5 in, 1 out]
              n63 = local write "H1 low UPH alarm (%)"(w136) -> ()
              n64 = call-poly <userlib>:"manageConfig.vi"("error in"=w89, "property path"="SCS.SimCfgCtrls.H1 enable halt on yield alarm", "config ref"=w151) -> ("error out"=w88:errorcluster, "value"=w135:bool, "config ref out"=w152:T10)  [unwired: 5 in, 1 out]
              n65 = local write "H1 enable halt\non yield alarm"(w135) -> ()
              n66 = call-poly <userlib>:"manageConfig.vi"("error in"=w88, "property path"="SCS.SimCfgCtrls.H1 enable halt on UPH alarm", "config ref"=w152) -> ("error out"=w87:errorcluster, "value"=w134:bool, "config ref out"=w153:T10)  [unwired: 5 in, 1 out]
              n67 = local write "H1 enable halt\non UPH alarm"(w134) -> ()
              n68 = call-poly <userlib>:"manageConfig.vi"("error in"=w87, "property path"="SCS.SimCfgCtrls.H2 low yield warning", "config ref"=w153) -> ("error out"=w86:errorcluster, "data"=w133:dbl, "config ref out"=w154:T10)  [unwired: 5 in, 1 out]
              n69 = local write "H2  low yield warning"(w133) -> ()
              n70 = call-poly <userlib>:"manageConfig.vi"("error in"=w86, "property path"="SCS.SimCfgCtrls.H2 low yield alarm", "config ref"=w154) -> ("error out"=w85:errorcluster, "data"=w132:dbl, "config ref out"=w155:T10)  [unwired: 5 in, 1 out]
              n71 = local write "H2 low yield alarm"(w132) -> ()
              n72 = call-poly <userlib>:"manageConfig.vi"("error in"=w85, "property path"="SCS.SimCfgCtrls.H2 low UPH warning (%)", "config ref"=w155) -> ("error out"=w84:errorcluster, "data"=w131:dbl, "config ref out"=w123:T10)  [unwired: 5 in, 1 out]
              n73 = local write "H2 low UPH warning (%)"(w131) -> ()
              n74 = call-poly <userlib>:"manageConfig.vi"("error in"=w84, "property path"="SCS.SimCfgCtrls.H2 low UPH alarm (%)", "config ref"=w123) -> ("error out"=w83:errorcluster, "data"=w121:dbl, "config ref out"=w122:T10)  [unwired: 5 in, 1 out]
              n75 = local write "H2 low UPH alarm (%)"(w121) -> ()
              n76 = call-poly <userlib>:"manageConfig.vi"("error in"=w83, "property path"="SCS.SimCfgCtrls.H2 enable halt on yield alarm", "config ref"=w122) -> ("error out"=w82:errorcluster, "value"=w130:bool, "config ref out"=w156:T10)  [unwired: 5 in, 1 out]
              n77 = local write "H2 enable halt\non yield alarm"(w130) -> ()
              n78 = call-poly <userlib>:"manageConfig.vi"("error in"=w82, "property path"="SCS.SimCfgCtrls.H2 enable halt on UPH alarm", "config ref"=w156) -> ("error out"=w81:errorcluster, "value"=w129:bool, "config ref out"=w120:T10)  [unwired: 5 in, 1 out]
              n79 = local write "H2 enable halt\non UPH alarm"(w129) -> ()
              n80 = call-poly <userlib>:"manageConfig.vi"("error in"=w81, "property path"="SCS.SimCfgCtrls.Ignore alarms until this many cycles", "config ref"=w120) -> ("error out"=w80:errorcluster, "value"=w128:i32, "config ref out"=w119:T10)  [unwired: 5 in, 1 out]
              n81 = local write "Ignore alarms until AFTER this many cycles"(w128) -> ()
              n82 = call-poly <userlib>:"manageConfig.vi"("error in"=w80, "property path"="SCS.SimCfgCtrls.Enable data logging", "config ref"=w119) -> ("error out"=w79:errorcluster, "value"=w127:bool, "config ref out"=w140:T10)  [unwired: 5 in, 1 out]
              n83 = local write "Enable data logging of all events"(w127) -> ()
              n84 = call-poly <userlib>:"manageConfig.vi"("error in"=w79, "property path"="SCS.SimCfgCtrls.Enable electronic notification of alarms", "config ref"=w140) -> ("error out"=w78:errorcluster, "value"=w126:bool, "config ref out"=w76:T10)  [unwired: 5 in, 1 out]
              n85 = local write "Enable electronic notification of alarms"(w126) -> ()
              n86 = call-poly <userlib>:"manageConfig.vi"("error in"=w78, "property path"="SCS.SimCfgCtrls.H1 allow lower parallelism", "config ref"=w76) -> ("error out"=w77:errorcluster, "value"=w70:bool, "config ref out"=w75:T10)  [unwired: 5 in, 1 out]
              n87 = local write "H1 allow lower parallelism"(w70) -> ()
              n88 = call-poly <userlib>:"manageConfig.vi"("error in"=w77, "property path"="SCS.SimCfgCtrls.H2 allow lower parallelism", "config ref"=w75) -> ("error out"=w73:errorcluster, "value"=w69:bool, "config ref out"=w74:T10)  [unwired: 5 in, 1 out]
              n89 = local write "H2 allow lower parallelism"(w69) -> ()
              n90 = call-poly <userlib>:"manageConfig.vi"("error in (no error)"=w73, "config ref"=w74) -> ()  [unwired: 9 in, 1 out]
            }
            frame #1 {
              # "Load data from the INI file for the Monitor tab"
              n91 = local read "Configuration file path and filename"() -> (w201:path)
              n92 = call-poly <userlib>:"manageConfig.vi"() -> ("error out"=w175:errorcluster, "config ref out"=w202:T10)  [unwired: 10 in]
              n93 = call-poly <userlib>:"manageConfig.vi"("error in (no error)"=w175, "access (0:read/write)"=enum16{"read/write", "read-only", "write-only"}."read-only", "config file path"=w201, "config ref"=w202) -> ("error out"=w204:errorcluster, "config ref out"=w206:T10)  [unwired: 5 in, 1 out]
              n94 = call-poly <userlib>:"manageConfig.vi"("error in"=w204, "property path"="SCS.Monitor.Optimize handler speed" ("key"), "config ref"=w206) -> ("error out"=w174:errorcluster, "value"=w184:bool, "config ref out"=w176:T10)  [unwired: 5 in, 1 out]
              n95 = local write "Optimize handler speed"(w184) -> ()
              n96 = call-poly <userlib>:"manageConfig.vi"("error in"=w174, "property path"="SCS.Monitor.Tester on-line" ("key"), "config ref"=w176) -> ("error out"=w173:errorcluster, "value"=w183:bool, "config ref out"=w197:T10)  [unwired: 5 in, 1 out]
              n97 = local write "Tester online"(w183) -> ()
              n98 = call-poly <userlib>:"manageConfig.vi"("error in"=w173, "property path"="SCS.Monitor.H1 on-line" ("key"), "config ref"=w197) -> ("error out"=w172:errorcluster, "value"=w182:bool, "config ref out"=w196:T10)  [unwired: 5 in, 1 out]
              n99 = local write "H1 online"(w182) -> ()
              n100 = call-poly <userlib>:"manageConfig.vi"("error in"=w172, "property path"="SCS.Monitor.H2 on-line" ("key"), "config ref"=w196) -> ("error out"=w171:errorcluster, "value"=w181:bool, "config ref out"=w195:T10)  [unwired: 5 in, 1 out]
              n101 = local write "H2 online"(w181) -> ()
              n102 = call-poly <userlib>:"manageConfig.vi"("error in"=w171, "property path"="SCS.Monitor.Utilization averaging", "config ref"=w195) -> ("error out"=w170:errorcluster, "value"=w177:i32, "config ref out"=w194:T10)  [unwired: 5 in, 1 out]
              n103 = local write "Utilization averaging"(w177) -> ()
              n104 = call-poly <userlib>:"manageConfig.vi"("error in"=w170, "property path"="SCS.Monitor.Audio On/Off", "config ref"=w194) -> ("error out"=w169:errorcluster, "config ref out"=w193:T10)  [unwired: 5 in, 2 out]
              n105 = call-poly <userlib>:"manageConfig.vi"("error in"=w169, "property path"="SCS.Monitor.Alert volume", "config ref"=w193) -> ("error out"=w168:errorcluster, "value"=w180:u32, "config ref out"=w192:T10)  [unwired: 5 in, 1 out]
              n106 = local write "Alert volume"(w180) -> ()
              n107 = call-poly <userlib>:"manageConfig.vi"("error in"=w168, "property path"="SCS.Monitor.UPH averaging", "config ref"=w192) -> ("error out"=w167:errorcluster, "value"=w179:u32, "config ref out"=w191:T10)  [unwired: 5 in, 1 out]
              n108 = local write "UPH averaging"(w179) -> ()
              n109 = call-poly <userlib>:"manageConfig.vi"("error in"=w167, "property path"="SCS.Monitor.Yield averaging", "config ref"=w191) -> ("error out"=w166:errorcluster, "value"=w178:u32, "config ref out"=w190:T10)  [unwired: 5 in, 1 out]
              n110 = local write "Yield averaging"(w178) -> ()
              n111 = call-poly <userlib>:"manageConfig.vi"("error in (no error)"=w166, "config ref"=w190) -> ()  [unwired: 9 in, 1 out]
            }
            frame #2 {
              # "Load data from the INI file for the Benefits tab"
              n112 = local read "Configuration file path and filename"() -> (w243:path)
              n113 = call-poly <userlib>:"manageConfig.vi"() -> ("error out"=w216:errorcluster, "config ref out"=w244:T10)  [unwired: 10 in]
              n114 = call-poly <userlib>:"manageConfig.vi"("error in (no error)"=w216, "access (0:read/write)"=enum16{"read/write", "read-only", "write-only"}."read-only", "config file path"=w243, "config ref"=w244) -> ("error out"=w246:errorcluster, "config ref out"=w248:T10)  [unwired: 5 in, 1 out]
              n115 = call-poly <userlib>:"manageConfig.vi"("error in"=w246, "property path"="SCS.Benefits.Tester cost" ("key"), "config ref"=w248) -> ("error out"=w215:errorcluster, "data"=w234:dbl, "config ref out"=w225:T10)  [unwired: 5 in, 1 out]
              n116 = local write "Tester cost ($/mo)"(w234) -> ()
              n117 = call-poly <userlib>:"manageConfig.vi"("error in"=w215, "property path"="SCS.Benefits.Handler cost" ("key"), "config ref"=w225) -> ("error out"=w214:errorcluster, "data"=w233:dbl, "config ref out"=w224:T10)  [unwired: 5 in, 1 out]
              n118 = local write "Handler cost ($/mo)"(w233) -> ()
              n119 = call-poly <userlib>:"manageConfig.vi"("error in"=w214, "property path"="SCS.Benefits.Test cell overhead" ("key"), "config ref"=w224) -> ("error out"=w213:errorcluster, "data"=w232:dbl, "config ref out"=w223:T10)  [unwired: 5 in, 1 out]
              n120 = local write "Overhead ($/mo)"(w232) -> ()
              n121 = call-poly <userlib>:"manageConfig.vi"("error in"=w213, "property path"="SCS.Benefits.Hours per month" ("key"), "config ref"=w223) -> ("error out"=w212:errorcluster, "value"=w231:i32, "config ref out"=w222:T10)  [unwired: 5 in, 1 out]
              n122 = local write "Hours per month"(w231) -> ()
              n123 = call-poly <userlib>:"manageConfig.vi"("error in"=w212, "property path"="SCS.Benefits.STD cell floorspace area" ("key"), "config ref"=w222) -> ("error out"=w211:errorcluster, "value"=w230:i32, "config ref out"=w221:T10)  [unwired: 5 in, 1 out]
              n124 = local write "Std cell \nfloorspace area"(w230) -> ()
              n125 = call-poly <userlib>:"manageConfig.vi"("error in"=w211, "property path"="SCS.Benefits.Celerint hardware cost" ("key"), "config ref"=w221) -> ("error out"=w210:errorcluster, "data"=w229:dbl, "config ref out"=w220:T10)  [unwired: 5 in, 1 out]
              n126 = local write "Celerint hardware cost ($/mo)"(w229) -> ()
              n127 = call-poly <userlib>:"manageConfig.vi"("error in"=w210, "property path"="SCS.Benefits.Celerint licensing cost" ("key"), "config ref"=w220) -> ("error out"=w209:errorcluster, "data"=w228:dbl, "config ref out"=w219:T10)  [unwired: 5 in, 1 out]
              n128 = local write "Celerint licensing cost ($/mo)"(w228) -> ()
              n129 = call-poly <userlib>:"manageConfig.vi"("error in"=w209, "property path"="SCS.Benefits.Second handler cost" ("key"), "config ref"=w219) -> ("error out"=w208:errorcluster, "data"=w227:dbl, "config ref out"=w218:T10)  [unwired: 5 in, 1 out]
              n130 = local write "Second handler cost ($/mo)"(w227) -> ()
              n131 = call-poly <userlib>:"manageConfig.vi"("error in"=w208, "property path"="SCS.Benefits.Additional floorspace for seconed handler" ("key"), "config ref"=w218) -> ("error out"=w207:errorcluster, "value"=w226:i32, "config ref out"=w217:T10)  [unwired: 5 in, 1 out]
              n132 = local write "Additional floorspace\nfor second handler"(w226) -> ()
              n133 = call-poly <userlib>:"manageConfig.vi"("error in (no error)"=w207, "config ref"=w217) -> ()  [unwired: 9 in, 1 out]
            }
            frame #3 {
              w259 = "SCS.Notification.Enable text notification"  # key
              w265 = "SCS.Notification.Phone Number"  # key
              w266 = "SCS.Notification.Enable email notification"  # key
              w273 = "SCS.Notification.Email alert - Engineer"  # key
              # "Load data from the INI file for the Benefits tab"
              n134 = local read "Configuration file path and filename"() -> (w270:path)
              n135 = call-poly <userlib>:"manageConfig.vi"() -> ("error out"=w255:errorcluster, "config ref out"=w271:T10)  [unwired: 10 in]
              n136 = call-poly <userlib>:"manageConfig.vi"("error in (no error)"=w255, "access (0:read/write)"=enum16{"read/write", "read-only", "write-only"}."read-only", "config file path"=w270, "config ref"=w271) -> ("error out"=w254:errorcluster, "config ref out"=w274:T10)  [unwired: 5 in, 1 out]
              n137 = call-poly <userlib>:"manageConfig.vi"("error in"=w254, "property path"=w273, "config ref"=w274) -> ("error out"=w253:errorcluster, "value"=w268:string, "config ref out"=w264:T10)  [unwired: 5 in, 1 out]
              n138 = local write "Email alert - engineer"(w268) -> ()
              n139 = call-poly <userlib>:"manageConfig.vi"("error in"=w253, "property path"="SCS.Notification.Email alert CC", "config ref"=w264) -> ("error out"=w252:errorcluster, "value"=w267:string, "config ref out"=w263:T10)  [unwired: 5 in, 1 out]
              n140 = local write "Email alert - CC"(w267) -> ()
              n141 = call-poly <userlib>:"manageConfig.vi"("error in"=w252, "property path"=w266, "config ref"=w263) -> ("error out"=w251:errorcluster, "value"=w261:bool, "config ref out"=w258:T10)  [unwired: 5 in, 1 out]
              n142 = local write "Enable email notification"(w261) -> ()
              n143 = call-poly <userlib>:"manageConfig.vi"("error in"=w251, "property path"=w259, "config ref"=w258) -> ("error out"=w250:errorcluster, "value"=w256:bool, "config ref out"=w257:T10)  [unwired: 5 in, 1 out]
              n144 = local write "Enable text notification"(w256) -> ()
              n145 = call-poly <userlib>:"manageConfig.vi"("error in"=w250, "property path"=w265, "config ref"=w257) -> ("error out"=w249:errorcluster, "value"=w260:string, "config ref out"=w262:T10)  [unwired: 5 in, 1 out]
              n146 = local write "Phone number"(w260) -> ()
              n147 = call-poly <userlib>:"manageConfig.vi"("error in (no error)"=w249, "config ref"=w262) -> ()  [unwired: 9 in, 1 out]
            }
            frame #4 {
              # "This reads the GPIB addresses and related command from the INI file (.cfg)"
              n148 = local read "Configuration file path and filename"() -> (w301:path)
              n149 = call-poly <userlib>:"manageConfig.vi"() -> ("config ref out"=w302:T10)  [unwired: 10 in, 1 out]
              n150 = call-poly <userlib>:"manageConfig.vi"("access (0:read/write)"=enum16{"read/write", "read-only", "write-only"}."read-only", "config file path"=w301, "config ref"=w302) -> ("error out"=w304:errorcluster, "config ref out"=w306:T10)  [unwired: 6 in, 1 out]
              n151 = call-poly <userlib>:"manageConfig.vi"("error in"=w304, "property path"="SCS.GPIB.Tester Address" ("key"), "config ref"=w306) -> ("error out"=w291:errorcluster, "value"=w283:string, "config ref out"=w297:T10)  [unwired: 5 in, 1 out]
              n152 = local write "Tester address"(w283) -> ()
              n153 = call-poly <userlib>:"manageConfig.vi"("error in"=w291, "property path"="SCS.GPIB.H1 Address" ("key"), "config ref"=w297) -> ("error out"=w290:errorcluster, "value"=w282:string, "config ref out"=w296:T10)  [unwired: 5 in, 1 out]
              n154 = local write "H1 Address"(w282) -> ()
              n155 = call-poly <userlib>:"manageConfig.vi"("error in"=w290, "property path"="SCS.GPIB.H2 Address" ("key"), "config ref"=w296) -> ("error out"=w289:errorcluster, "value"=w281:string, "config ref out"=w295:T10)  [unwired: 5 in, 1 out]
              n156 = local write "H2 Address"(w281) -> ()
              n157 = call-poly <userlib>:"manageConfig.vi"("error in"=w289, "property path"="SCS.GPIB.SOT" ("key"), "config ref"=w295) -> ("error out"=w288:errorcluster, "config ref out"=w277:T10)  [unwired: 5 in, 2 out]
              n158 = call-poly <userlib>:"manageConfig.vi"("error in"=w288, "property path"="SCS.GPIB.Get Handler Velocity" ("key"), "config ref"=w277) -> ("error out"=w287:errorcluster, "value"=w280:string, "config ref out"=w276:T10)  [unwired: 5 in, 1 out]
              n159 = local write "Get Handler Velocity"(w280) -> ()
              n160 = call-poly <userlib>:"manageConfig.vi"("error in"=w287, "property path"="SCS.GPIB.Increase Handler Velocity" ("key"), "config ref"=w276) -> ("error out"=w286:errorcluster, "value"=w279:string, "config ref out"=w275:T10)  [unwired: 5 in, 1 out]
              n161 = local write "Increase Handler Velocity"(w279) -> ()
              n162 = call-poly <userlib>:"manageConfig.vi"("error in"=w286, "property path"="SCS.GPIB.Decrease Handler Velocity" ("key"), "config ref"=w275) -> ("error out"=w285:errorcluster, "value"=w278:string, "config ref out"=w284:T10)  [unwired: 5 in, 1 out]
              n163 = local write "Decrease Handler Velocity"(w278) -> ()
              n164 = call-poly <userlib>:"manageConfig.vi"("error in (no error)"=w285, "config ref"=w284) -> ()  [unwired: 9 in, 1 out]
            }
          }
        }
      }
    }
    frame #4 {
      # "This frame writes the headewr to the data log.\nIt includes setup and configuration information for the lot."
      n165 = local read "POWER"() -> (w307:bool)
      n166 = case shown="True" w307 {
        frame False {
        }
        frame True {
          w313 = "\r\n"
          n167 = local read "Lot number"() -> (w317:string)
          n168 = local read "Test cell ID"() -> (w315:string)
          n169 = local read "H1 online"() -> (w325:bool)
          n170 = local read "H2 online"() -> (w326:bool)
          n171 = local read "Data log path and filename"() -> (w308:path)
          n172 = local read "Operator name"() -> (w319:string)
          n173 = local read "H1 UPH warning limit hid"() -> (w321:dbl)
          n174 = local read "H2 UPH warning limit hid"() -> (w323:dbl)
          n175 = local read "H2  low yield warning"() -> (w322:dbl)
          n176 = local read "H1 low yield warning"() -> (w320:dbl)
          n177 = case shown="True" w325 {
            tunnel: ["H1 Off-Line" "H1 On-Line"] -> w327
            frame False {
            }
            frame True {
            }
          }
          n178 = case shown="True" w326 {
            tunnel: ["H2 Off-Line" "H2 On-Line"] -> w332
            frame False {
            }
            frame True {
            }
          }
          n179 = local write "Email alert - attachment (not editable)"(w308) -> ()
          n180 = Number To Decimal String(number=w320) -> (decimal integer string=w329:string)  [unwired: 1 in]
          n181 = Number To Decimal String(number=w321) -> (decimal integer string=w331:string)  [unwired: 1 in]
          n182 = Number To Decimal String(number=w322) -> (decimal integer string=w334:string)  [unwired: 1 in]
          n183 = Number To Decimal String(number=w323) -> (decimal integer string=w336:string)  [unwired: 1 in]
          n184 = Get Date/Time String() -> (date string=w310:string, time string=w312:string)  [unwired: 3 in]
          n185 = Concatenate Strings(w310, "   " ("string"), w312, w313, "Test Cell ID: ", w315, w313, "Lot Number: ", w317, w313, "Operator Name:  ", w319, w313, "System Started", w313, w327, w313, "H1 Low Yield Warning Limit: ", w329, w313, "H1 Low UPH Warning Limit: ", w331, w313, w332, w313, "H2 Low Yield Warning Limit: ", w334, w313, "H2 Low UPH Warning Limit: ", w336, w313, w313) -> (w337:string)
          n186 = call "SentinelDatalog.vi"("operation (0:open)"=T9."open or create", "String"=w337, "data log path"=w308) -> ()  [unwired: 8 in, 1 out]
        }
      }
    }
    frame #5 {
      # "This frame implements the main Sentinel Controller loop.\nAll loops within this frame execute as parallel processes."
      n187 = local read "POWER"() -> (w342:bool)
      n188 = case shown="True" w342 {
        frame False {
        }
        frame True {
          n189 = while {
            stop <- w357 stop-if-true
            w347 = 0
            w346 = 0.0
            w354 = 0
            w355 = 0.0
            # "Sentinel operating loop\n- tester loop\n- H1 loop\n- H2 loop\n- controls loop\n- alarm state machine loop\nExit with Power off"
            n190 = local read "POWER"() -> (w358:bool)
            n191 = Wait (ms)(milliseconds to wait=u32 100) -> ()  [unwired: 1 out]
            n192 = Not(x=w358) -> (.not. x?=w357:bool)
            n193 = while {
              i -> [w2475]
              stop <- w2491 stop-if-true
              n194 = local read "Run"() -> (w2467:bool)
              n195 = First Call?() -> (First Call?: T/F=w2468:bool)
              n196 = case shown="True" w2467 {
                frame False {
                  n197 = local write "Tester online"(FALSE ("Tester online")) -> ()
                  n198 = local write "H2 online"(FALSE ("H2 online")) -> ()
                  n199 = local write "H1 online"(FALSE ("H1 online")) -> ()
                }
                frame True {
                }
              }
              n200 = local read "Additional floorspace\nfor second handler"() -> (w2476:i32)
              n201 = Wait (ms)(milliseconds to wait=u32 50) -> ()  [unwired: 1 out]
              n202 = local read "Optimize handler speed"() -> (w2484:bool)
              n203 = local read "Std cell \nfloorspace area"() -> (w2489:i32)
              n204 = local read "Std cell \nfloorspace area"() -> (w2461:i32)
              n205 = local read "Celerint hardware cost ($/mo)"() -> (w2479:dbl)
              n206 = local read "Celerint licensing cost ($/mo)"() -> (w2478:dbl)
              n207 = local read "Second handler cost ($/mo)"() -> (w2477:dbl)
              n208 = case shown="True" w2468 {
                frame False {
                }
                frame True {
                  n209 = local read "H1 parallelism"() -> (w2524:u32)
                  n210 = local read "H2 parallelism"() -> (w2523:u32)
                  n211 = local read "H1 index time expected hid"() -> (w2522:dbl)
                  n212 = local read "H1 index time expected hid"() -> (w2532:dbl)
                  n213 = local read "H2 index time expected hid"() -> (w2521:dbl)
                  n214 = local read "H2 index time expected hid"() -> (w2533:dbl)
                  n215 = local read "Test time expected hid"() -> (w2530:dbl)
                  n216 = local write "H2 units/cycle"(w2523) -> ()
                  n217 = local write "H1 units/cycle"(w2524) -> ()
                  n218 = formula code="H1UPHorig=P1*3600/(T+H1ITorig);\nH2UPHorig=P2*3600/(T+H2ITorig);\nSYSH1WT=T-H1I;\nSYSH2WT=T-H2I;"("T"=w2530, "H1I"=w2522, "H2I"=w2521, "P1"=w2524, "H1ITorig"=w2532, "H2ITorig"=w2533, "P2"=w2523) -> ("H1UPHorig"=w2520:dbl, "H2UPHorig"=w2519:dbl, "SYSH1WT"=w2539:dbl, "SYSH2WT"=w2538:dbl)
                  n219 = local write "H1 Index Time 2"(w2522) -> ()
                  n220 = local write "H1 Test Time 2"(w2521) -> ()
                  n221 = local write "H1 P in formula"(w2524) -> ()
                  n222 = local write "H2 calc UPH"(w2519) -> ()
                  n223 = local read "H1 index time expected hid"() -> (w2526:dbl)
                  n224 = local read "H2 index time expected hid"() -> (w2525:dbl)
                  n225 = local read "Test time expected hid"() -> (w2527:dbl)
                  n226 = local write "H1 calc UPH"(w2520) -> ()
                  n227 = local write "UPH"(w2520) -> ()
                  n228 = local read "H2 parallelism"() -> (w2529:u32)
                  n229 = local read "H1 parallelism"() -> (w2528:u32)
                  n230 = Less Than 0?(x=w2539) -> (x < 0?=w2540:bool)
                  n231 = Less Than 0?(x=w2538) -> (x < 0?=w2541:bool)
                  n232 = Select(t=0.0, s=w2540, f=w2539) -> (s? t:f=w2535:dbl)
                  n233 = Select(t=0.0, s=w2541, f=w2538) -> (s? t:f=w2534:dbl)
                  n234 = local read "H1 index time expected hid"() -> (w2518:dbl)
                  n235 = local read "H2 index time expected hid"() -> (w2517:dbl)
                  n236 = local read "Test time expected hid"() -> (w2513:dbl)
                  n237 = formula code="ExpH1UPH=P1*3600/(T+SYSH1I+SYSH1WT);\nExpH2UPH=P2*3600/(T+SYSH2I+SYSH2WT);\nMaxUPH=Margin*(ExpH1UPH+ExpH2UPH);"("P1"=w2529, "T"=w2527, "SYSH1I"=w2526, "SYSH2I"=w2525, "Margin"=1.05 ("input variable"), "SYSH1WT"=w2535, "SYSH2WT"=w2534, "P2"=w2528) -> ("MaxUPH"=w2531:dbl, "ExpH1UPH"=w2537:dbl, "ExpH2UPH"=w2536:dbl)
                  n238 = Add(x=w2518, y=w2517) -> (x+y=w2516:dbl)
                  n239 = Divide(x=w2516, y=2.0) -> (x/y=w2514:dbl)
                  n240 = Add(x=w2513, y=w2514) -> (x+y=w2512:dbl)
                  n241 = Multiply(x=4000.0, y=w2512) -> (x*y=w2510:dbl)
                  n242 = To Unsigned Long Integer(number=w2510) -> (unsigned 32bit integer=w2509:u32)
                  n243 = local write "GPIB wait timeout hid"(w2509) -> ()
                  n244 = property on="System UPH" class="Knob (strict)"("Scale.Maximum"=w2531) -> ()  [unwired: 2 in, 2 out]
                  n245 = property on="H1 UPH" class="Knob (strict)"("Scale.Maximum"=w2537) -> ()  [unwired: 2 in, 2 out]
                  n246 = property on="H2 UPH" class="Knob (strict)"("Scale.Maximum"=w2536) -> ()  [unwired: 2 in, 2 out]
                }
              }
              n247 = local read "Handler cost ($/mo)"() -> (w2481:dbl)
              n248 = local read "Tester cost ($/mo)"() -> (w2482:dbl)
              n249 = local read "H1 online"() -> (w2471:bool)
              n250 = local read "H2 online"() -> (w2470:bool)
              n251 = local read "Overhead ($/mo)"() -> (w2480:dbl)
              n252 = local read "POWER"() -> (w2493:bool)
              n253 = Not(x=w2493) -> (.not. x?=w2492:bool)
              n254 = Not(x=w2471) -> (.not. x?=w2459:bool)
              n255 = Not(x=w2470) -> (.not. x?=w2458:bool)
              n256 = local read "Hours per month"() -> (w2463:i32)
              n257 = case shown="True" w2484 {
                frame False {
                }
                frame True {
                  # "place code here to optimize handler index times"
                }
              }
              n258 = local write "Std cell floorspace area"(w2461) -> ()
              n259 = Compound Arithmetic op=OR(w2492) -> (w2491:bool)
              n260 = And(x=w2459, y=w2458) -> (x .and. y?=w2469:bool)
              n261 = case shown="True" w2459 {
                frame False {
                }
                frame True {
                  n262 = local write "H1 nominal 2"(TRUE) -> ()
                  n263 = local write "H1 nominal"(TRUE) -> ()
                  n264 = local write "H1 warning 2"(TRUE) -> ()
                  n265 = local write "H1 warning"(TRUE) -> ()
                  n266 = local write "H1 alarm 2"(TRUE) -> ()
                  n267 = local write "H1 alarm"(TRUE) -> ()
                }
              }
              n268 = local write "H1 On/Off-line"(w2459) -> ()
              n269 = case shown="True" w2458 {
                frame False {
                }
                frame True {
                  n270 = local write "H2 nominal"(TRUE) -> ()
                  n271 = local write "H2 nominal 2"(TRUE) -> ()
                  n272 = local write "H2 warning"(TRUE) -> ()
                  n273 = local write "H2 warning 2"(TRUE) -> ()
                  n274 = local write "H2 alarm"(TRUE) -> ()
                  n275 = local write "H2 alarm 2"(TRUE) -> ()
                }
              }
              n276 = local write "H2 On/Off-line"(w2458) -> ()
              n277 = Add(x=w2476, y=w2489) -> (x+y=w2460:i32)
              n278 = Compound Arithmetic op=ADD(w2482, w2481, w2480) -> (w2486:dbl)
              n279 = Compound Arithmetic op=ADD(w2479, w2478, w2477) -> (w2487:dbl)
              n280 = Compound Arithmetic op=ADD(w2482, w2480) -> (w2464:dbl)
              n281 = case shown="False" w2469 {
                frame False {
                }
                frame True {
                  n282 = local write "System UPH"(u32 0 ("System UPH")) -> ()
                  n283 = local write "Sys utilization"(0.0 ("Sys utilization")) -> ()
                }
              }
              n284 = local write "Tandem\nfloorspace area"(w2460) -> ()
              n285 = Divide(x=w2487, y=w2463) -> (x/y=w2490:dbl)
              n286 = Add(x=w2487, y=w2486) -> (x+y=w2466:dbl)
              n287 = Divide(x=w2486, y=w2463) -> (x/y=w2462:dbl)
              n288 = local write "Hours per month 2"(w2463) -> ()
              n289 = local write "Total Mo Costs ($/mo) 2"(w2464) -> ()
              n290 = local write "Total Mo Costs ($/mo) 3"(w2466) -> ()
              n291 = local write "Std mo cost ($/mo)"(w2464) -> ()
              n292 = Add(x=w2462, y=w2490) -> (x+y=w2465:dbl)
              n293 = local write "Std hourly\ncost ($/hr)"(w2462) -> ()
              n294 = local read "Push to reset charts"() -> (w2473:bool)
              n295 = local write "Tandem hourly\ncost ($/hr)"(w2465) -> ()
              n296 = local read "Optimize handler speed"() -> (w2472:bool)
              n297 = case shown="True" w2473 {
                frame False {
                }
                frame True {
                  n298 = property on="YieldMon" class="WFChart (strict)"("History Data"=cluster{dbl, dbl, dbl, dbl}[] [{100.0, 100.0, 0.0, 0.0}]) -> ()  [unwired: 2 in, 2 out]
                  n299 = property on="SysUtilMon" class="WFChart (strict)"("History Data"=cluster{dbl, dbl}[] []) -> ()  [unwired: 2 in, 2 out]
                }
              }
              n300 = Equal To 0?(x=w2475) -> (x = 0?=w2474:bool)
              n301 = case shown="True" w2474 {
                frame False {
                }
                frame True {
                  w2568 = "" ("Message from tester")
                  w2571 = 0
                  w2574 = 0
                  w2587 = 100
                  w2588 = 0
                  w2589 = FALSE ("H1 alarm")
                  # "graphs and charts - declared here, displayed elsewhere"
                  n302 = Bundle(w2587, w2587, w2587, w2587) -> (w2566:cluster{i32, i32, i32, i32})  [unwired: 1 in]
                  n303 = Bundle(w2588, w2588) -> (w2565:cluster{i32, i32})  [unwired: 1 in]
                  n304 = local write "H2 Lock"(FALSE ("H2 Lock")) -> ()
                  n305 = local write "H1 alarm"(FALSE ("H1 warning")) -> ()
                  n306 = local write "H1 Lock"(FALSE ("H1 Lock")) -> ()
                  n307 = local write "H2 warning 2"(FALSE ("H1 warning")) -> ()
                  n308 = local write "H2 warning"(FALSE ("H1 warning")) -> ()
                  n309 = local write "H1 warning 2"(FALSE ("H1 warning")) -> ()
                  n310 = local write "H1 warning"(FALSE ("H1 warning")) -> ()
                  n311 = local write "H2 nominal 2"(TRUE ("H1 nominal")) -> ()
                  n312 = local write "H2 alarm 2"(FALSE ("H1 warning")) -> ()
                  n313 = local write "H2 alarm"(FALSE ("H1 warning")) -> ()
                  n314 = local write "H1 nominal 2"(TRUE ("H1 nominal")) -> ()
                  n315 = local write "H1 alarm 2"(FALSE ("H1 warning")) -> ()
                  n316 = local write "system statuts hid"(T8."H1NH2N" ("system statuts")) -> ()
                  n317 = local write "H1 Good Units"(w2574) -> ()
                  n318 = local write "H2 Device Count"(w2574) -> ()
                  n319 = local write "H2 Good Units"(w2574) -> ()
                  n320 = local write "H1 Device Count"(w2574) -> ()
                  n321 = property on="System UPH" class="Knob (strict)"("Scale.Minimum"=w2571) -> ()  [unwired: 2 in, 2 out]
                  n322 = property on="H1 UPH" class="Knob (strict)"("Scale.Minimum"=w2571) -> ()  [unwired: 2 in, 2 out]
                  n323 = property on="H2 UPH" class="Knob (strict)"("Scale.Minimum"=w2571) -> ()  [unwired: 2 in, 2 out]
                  n324 = property on="SysUtilMon" class="WFChart (strict)"("History Data"=cluster{dbl, dbl}[] []) -> ()  [unwired: 2 in, 2 out]
                  n325 = local write "H1 alarm"(w2589) -> ()
                  n326 = local write "H2 alarm"(w2589) -> ()
                  n327 = property on="YieldMon" class="WFChart (strict)"("History Data"=cluster{dbl, dbl, dbl, dbl}[] []) -> ()  [unwired: 2 in, 2 out]
                  n328 = local write "YieldMon"(w2566) -> ()
                  n329 = local write "SysUtilMon"(w2565) -> ()
                  n330 = local write "Sys utilization"(0.0) -> ()
                  n331 = local write "H2 alarm 2"(w2589) -> ()
                  n332 = local write "H1 alarm 2"(w2589) -> ()
                  n333 = local write "H2 nominal"(TRUE ("H1 nominal")) -> ()
                  n334 = local write "H1 nominal"(TRUE ("H1 nominal")) -> ()
                  n335 = local read "Lot number"() -> (w2563:string)
                  n336 = local write "Number of text alerts"(0.0 ("Number of Emails Alerts Sent")) -> ()
                  n337 = local write "Number of email alerts"(u32 0 ("Number of Emails Alerts Sent")) -> ()
                  n338 = local write "Tester loop counter hid"(u32 0 ("Tester loop counter")) -> ()
                  n339 = local write "H1 loop counter hid"(u32 0 ("H1 loop counter hid")) -> ()
                  n340 = local write "H2 loop counter hid"(u32 0 ("H2 loop counter hid")) -> ()
                  n341 = local write "H1 Waiting"(FALSE ("H1 Ready with sites")) -> ()
                  n342 = local write "H2 Waiting"(FALSE ("H1 Ready with sites")) -> ()
                  n343 = local write "GPIB Bus 0 traffic"(w2568) -> ()
                  n344 = local write "Notifications Lot Display"(w2563) -> ()
                  n345 = local write "GPIB bus 1 traffic"(w2568) -> ()
                  n346 = local write "GPIB bus 2 traffic"(w2568) -> ()
                }
              }
              n347 = case shown="True" w2472 {
                frame False {
                }
                frame True {
                  w2548 = FALSE
                  n348 = local read "H1 online"() -> (w2550:bool)
                  n349 = local read "H2 online"() -> (w2549:bool)
                  n350 = Equal?(x=w2550, y=w2548) -> (x = y?=w2552:bool)
                  n351 = Equal?(x=w2548, y=w2549) -> (x = y?=w2551:bool)
                  n352 = Or(x=w2552, y=w2551) -> (x .or. y?=w2547:bool)
                  n353 = case shown="True" w2547 {
                    frame False {
                    }
                    frame True {
                      n354 = local write "Optimize handler speed"(FALSE ("Optimize Handler Speed")) -> ()
                    }
                  }
                }
              }
              n355 = local read "Alert volume"() -> (w2483:u32)
              n356 = Equal To 0?(x=w2483) -> (x = 0?=w2485:bool)
              n357 = case shown="True" w2485 {
                frame False {
                }
                frame True {
                  n358 = local write "Audio On / Off"(FALSE ("Audio On/Off")) -> ()
                }
              }
            }
            n359 = case shown="True" FALSE {
              frame False {
              }
              frame True {
                n360 = while {
                  i -> [w602]
                  stop <- w615 stop-if-true
                  # "Play Audio Aert Loop"
                  n361 = local read "Ignore alarms until AFTER this many cycles"() -> (w607:i32)
                  n362 = local read "H1 Device Count"() -> (w612:u32)
                  n363 = local read "H2 Device Count"() -> (w611:u32)
                  n364 = local read "Program Parallelism"() -> (w609:u32)
                  n365 = local read "Run"() -> (w604:bool)
                  n366 = local read "POWER"() -> (w605:bool)
                  n367 = Add(x=w612, y=w611) -> (x+y=w610:u32)
                  n368 = Wait (ms)(milliseconds to wait=u32 100) -> ()  [unwired: 1 out]
                  n369 = Divide(x=w610, y=w609) -> (x/y=w608:dbl)
                  n370 = Greater?(x=w602, y=50) -> (0:w600:bool)
                  n371 = Greater?(x=w608, y=w607) -> (0:w606:bool)
                  n372 = Compound Arithmetic op=AND(w606, w605, w604, w600) -> (w603:bool)
                  n373 = case shown="True" w603 {
                    frame False {
                    }
                    frame True {
                      n374 = local read "system statuts hid"() -> (w619:T8)
                      n375 = case shown="\"H1AH2A\"" w619 {
                        frame "H1NH2N", Default {
                          n376 = Wait (ms)(milliseconds to wait=u32 50) -> ()  [unwired: 1 out]
                        }
                        frame "H1NH2W" {
                          n377 = flat-sequence {
                            frame #0 {
                              n378 = local read "Audio On / Off"() -> (w622:bool)
                              n379 = local read "H2 online"() -> (w621:bool)
                              n380 = And(x=w621, y=w622) -> (x .and. y?=w623:bool)
                              n381 = case shown="True" w623 {
                                frame False {
                                }
                                frame True {
                                n382 = local read "Run"() -> (w626:bool)
                                n383 = case shown="True" w626 {
                                tunnel: [0.001 w628] -> w625
                                frame False {
                                }
                                frame True {
                                n384 = local read "Alert volume"() -> (w628:u32)
                                }
                                }
                                n385 = call "PlayAlarm.vi"("wavefilename"="audio\\4_synth_warning.wav", "alertvolume"=w625) -> ()  [unwired: 10 in]
                                }
                              }
                            }
                            frame #1 {
                              n386 = local read "Run"() -> (w629:bool)
                              n387 = case shown="True" w629 {
                                frame False {
                                }
                                frame True {
                                n388 = Wait (ms)(milliseconds to wait=u32 5000) -> ()  [unwired: 1 out]
                                }
                              }
                            }
                          }
                        }
                        frame "H1NH2A" {
                          n389 = flat-sequence {
                            frame #0 {
                              n390 = local read "Audio On / Off"() -> (w633:bool)
                              n391 = local read "H2 online"() -> (w632:bool)
                              n392 = And(x=w632, y=w633) -> (x .and. y?=w631:bool)
                              n393 = case shown="True" w631 {
                                frame False {
                                }
                                frame True {
                                n394 = local read "Run"() -> (w636:bool)
                                n395 = case shown="True" w636 {
                                tunnel: [0.001 w638] -> w635
                                frame False {
                                }
                                frame True {
                                n396 = local read "Alert volume"() -> (w638:u32)
                                }
                                }
                                n397 = call "PlayAlarm.vi"("wavefilename"="audio\\bass_synth_alarm.wav", "alertvolume"=w635) -> ()  [unwired: 10 in]
                                }
                              }
                            }
                            frame #1 {
                              n398 = local read "Run"() -> (w639:bool)
                              n399 = case shown="True" w639 {
                                frame False {
                                n400 = Wait (ms)(milliseconds to wait=u32 50) -> ()  [unwired: 1 out]
                                }
                                frame True {
                                n401 = Wait (ms)(milliseconds to wait=u32 5000) -> ()  [unwired: 1 out]
                                }
                              }
                            }
                          }
                        }
                        frame "H1WH2N" {
                          n402 = flat-sequence {
                            frame #0 {
                              n403 = local read "Audio On / Off"() -> (w644:bool)
                              n404 = local read "H1 online"() -> (w643:bool)
                              n405 = And(x=w643, y=w644) -> (x .and. y?=w642:bool)
                              n406 = case shown="True" w642 {
                                frame False {
                                }
                                frame True {
                                n407 = local read "Run"() -> (w647:bool)
                                n408 = case shown="True" w647 {
                                tunnel: [0.001 w649] -> w646
                                frame False {
                                }
                                frame True {
                                n409 = local read "Alert volume"() -> (w649:u32)
                                }
                                }
                                n410 = call "PlayAlarm.vi"("wavefilename"="audio\\4_synth_warning.wav", "alertvolume"=w646) -> ()  [unwired: 10 in]
                                }
                              }
                            }
                            frame #1 {
                              n411 = local read "Run"() -> (w650:bool)
                              n412 = case shown="True" w650 {
                                frame False {
                                n413 = Wait (ms)(milliseconds to wait=u32 50) -> ()  [unwired: 1 out]
                                }
                                frame True {
                                n414 = Wait (ms)(milliseconds to wait=u32 5000) -> ()  [unwired: 1 out]
                                }
                              }
                            }
                          }
                        }
                        frame "H1WH2W" {
                          n415 = flat-sequence {
                            frame #0 {
                              n416 = local read "Audio On / Off"() -> (w656:bool)
                              n417 = local read "H1 online"() -> (w653:bool)
                              n418 = local read "H2 online"() -> (w655:bool)
                              n419 = Compound Arithmetic op=AND(w653, w655, w656) -> (w654:bool)
                              n420 = case shown="True" w654 {
                                frame False {
                                }
                                frame True {
                                n421 = local read "Run"() -> (w659:bool)
                                n422 = case shown="True" w659 {
                                tunnel: [0.001 w661] -> w658
                                frame False {
                                }
                                frame True {
                                n423 = local read "Alert volume"() -> (w661:u32)
                                }
                                }
                                n424 = call "PlayAlarm.vi"("wavefilename"="audio\\4_synth_warning.wav", "alertvolume"=w658) -> ()  [unwired: 10 in]
                                }
                              }
                            }
                            frame #1 {
                              n425 = local read "Run"() -> (w662:bool)
                              n426 = case shown="True" w662 {
                                frame False {
                                n427 = Wait (ms)(milliseconds to wait=u32 50) -> ()  [unwired: 1 out]
                                }
                                frame True {
                                n428 = Wait (ms)(milliseconds to wait=u32 5000) -> ()  [unwired: 1 out]
                                }
                              }
                            }
                          }
                        }
                        frame "H1WH2A" {
                          n429 = flat-sequence {
                            frame #0 {
                              n430 = local read "Audio On / Off"() -> (w668:bool)
                              n431 = local read "H1 online"() -> (w666:bool)
                              n432 = local read "H2 online"() -> (w667:bool)
                              n433 = Compound Arithmetic op=AND(w666, w667, w668) -> (w665:bool)
                              n434 = case shown="True" w665 {
                                frame False {
                                }
                                frame True {
                                n435 = local read "Run"() -> (w671:bool)
                                n436 = case shown="True" w671 {
                                tunnel: [0.001 w673] -> w670
                                frame False {
                                }
                                frame True {
                                n437 = local read "Alert volume"() -> (w673:u32)
                                }
                                }
                                n438 = call "PlayAlarm.vi"("wavefilename"="audio\\bass_synth_alarm.wav", "alertvolume"=w670) -> ()  [unwired: 10 in]
                                }
                              }
                            }
                            frame #1 {
                              n439 = local read "Run"() -> (w674:bool)
                              n440 = case shown="True" w674 {
                                frame False {
                                n441 = Wait (ms)(milliseconds to wait=u32 50) -> ()  [unwired: 1 out]
                                }
                                frame True {
                                n442 = Wait (ms)(milliseconds to wait=u32 5000) -> ()  [unwired: 1 out]
                                }
                              }
                            }
                          }
                        }
                        frame "H1AH2N" {
                          n443 = flat-sequence {
                            frame #0 {
                              n444 = local read "Audio On / Off"() -> (w679:bool)
                              n445 = local read "H1 online"() -> (w677:bool)
                              n446 = And(x=w677, y=w679) -> (x .and. y?=w678:bool)
                              n447 = case shown="True" w678 {
                                frame False {
                                }
                                frame True {
                                n448 = local read "Run"() -> (w682:bool)
                                n449 = case shown="True" w682 {
                                tunnel: [0.001 w684] -> w681
                                frame False {
                                }
                                frame True {
                                n450 = local read "Alert volume"() -> (w684:u32)
                                }
                                }
                                n451 = call "PlayAlarm.vi"("wavefilename"="audio\\bass_synth_alarm.wav", "alertvolume"=w681) -> ()  [unwired: 10 in]
                                }
                              }
                            }
                            frame #1 {
                              n452 = local read "Run"() -> (w685:bool)
                              n453 = case shown="True" w685 {
                                frame False {
                                n454 = Wait (ms)(milliseconds to wait=u32 50) -> ()  [unwired: 1 out]
                                }
                                frame True {
                                n455 = Wait (ms)(milliseconds to wait=u32 5000) -> ()  [unwired: 1 out]
                                }
                              }
                            }
                          }
                        }
                        frame "H1AH2W" {
                          n456 = flat-sequence {
                            frame #0 {
                              n457 = local read "Audio On / Off"() -> (w691:bool)
                              n458 = local read "H1 online"() -> (w689:bool)
                              n459 = local read "H2 online"() -> (w690:bool)
                              n460 = Compound Arithmetic op=AND(w689, w690, w691) -> (w688:bool)
                              n461 = case shown="True" w688 {
                                frame False {
                                }
                                frame True {
                                n462 = local read "Run"() -> (w694:bool)
                                n463 = case shown="True" w694 {
                                tunnel: [0.001 w696] -> w693
                                frame False {
                                }
                                frame True {
                                n464 = local read "Alert volume"() -> (w696:u32)
                                }
                                }
                                n465 = call "PlayAlarm.vi"("wavefilename"="audio\\bass_synth_alarm.wav", "alertvolume"=w693) -> ()  [unwired: 10 in]
                                }
                              }
                            }
                            frame #1 {
                              n466 = local read "Run"() -> (w697:bool)
                              n467 = case shown="True" w697 {
                                frame False {
                                n468 = Wait (ms)(milliseconds to wait=u32 50) -> ()  [unwired: 1 out]
                                }
                                frame True {
                                n469 = Wait (ms)(milliseconds to wait=u32 5000) -> ()  [unwired: 1 out]
                                }
                              }
                            }
                          }
                        }
                        frame "H1AH2A" {
                          n470 = flat-sequence {
                            frame #0 {
                              n471 = local read "Audio On / Off"() -> (w703:bool)
                              n472 = local read "H1 online"() -> (w701:bool)
                              n473 = local read "H2 online"() -> (w702:bool)
                              n474 = Compound Arithmetic op=AND(w701, w702, w703) -> (w700:bool)
                              n475 = case shown="True" w700 {
                                frame False {
                                }
                                frame True {
                                n476 = local read "Run"() -> (w706:bool)
                                n477 = case shown="True" w706 {
                                tunnel: [0.001 w708] -> w705
                                frame False {
                                }
                                frame True {
                                n478 = local read "Alert volume"() -> (w708:u32)
                                }
                                }
                                n479 = call "PlayAlarm.vi"("wavefilename"="audio\\bass_synth_alarm.wav", "alertvolume"=w705) -> ()  [unwired: 10 in]
                                }
                              }
                            }
                            frame #1 {
                              n480 = local read "Run"() -> (w709:bool)
                              n481 = case shown="True" w709 {
                                frame False {
                                n482 = Wait (ms)(milliseconds to wait=u32 50) -> ()  [unwired: 1 out]
                                }
                                frame True {
                                n483 = Wait (ms)(milliseconds to wait=u32 5000) -> ()  [unwired: 1 out]
                                }
                              }
                            }
                          }
                        }
                      }
                    }
                  }
                  n484 = local read "Run"() -> (w613:bool)
                  n485 = local read "POWER"() -> (w616:bool)
                  n486 = Not(x=w616) -> (.not. x?=w618:bool)
                  n487 = Not(x=w613) -> (.not. x?=w617:bool)
                  n488 = Compound Arithmetic op=OR(w618, w617) -> (w615:bool)
                }
              }
            }
            n489 = while {
              shift-right: [w1878] -> _
              shift-left: T8."H1NH2N" ("system statuts") -> [w1868]
              stop <- w1867 continue-if-true
              # "system status state machine:\n- writes data log whenever there is a change (if data loggin enabled)\n- issues email and text alerts is enabled (electronic notification of alarms)"
              n490 = local read "H1 parallelism"() -> (w1874:u32)
              n491 = local read "H1 Device Count"() -> (w1875:u32)
              n492 = local read "H2 Device Count"() -> (w1873:u32)
              n493 = local read "H2 parallelism"() -> (w1872:u32)
              n494 = local read "POWER"() -> (w1867:bool)
              n495 = Divide(x=w1873, y=w1872) -> (x/y=w1869:dbl)
              n496 = Divide(x=w1875, y=w1874) -> (x/y=w1870:dbl)
              n497 = local read "Ignore alarms until AFTER this many cycles"() -> (w1877:i32)
              n498 = Add(x=w1870, y=w1869) -> (x+y=w1871:dbl)
              n499 = Greater?(x=w1871, y=w1877) -> (0:w1876:bool)
              n500 = case shown="True" w1876 {
                tunnel: [w1880 w1883] -> w1878
                tunnel: w1868 -> [w1880 w1881]
                frame False {
                }
                frame True {
                  n501 = flat-sequence {
                    tunnel: [w1884] -> w1882
                    tunnel: w1881 -> [w1884]
                    tunnel: [w1981] -> w1883
                    tunnel: w1882 -> [w1979]
                    frame #0 {
                      # "Determine current state for System Status state-machine"
                      n502 = stacked-sequence {
                        frame #0 {
                          n503 = local read "H1 nominal 2"() -> (w1888:bool)
                          n504 = local read "H2 nominal 2"() -> (w1886:bool)
                          n505 = local read "H1 nominal"() -> (w1889:bool)
                          n506 = local read "H2 nominal"() -> (w1887:bool)
                          n507 = Compound Arithmetic op=AND(w1889, w1888, w1887, w1886) -> (w1885:bool)
                          n508 = case shown="True" w1885 {
                            frame False {
                            }
                            frame True {
                              n509 = local write "system statuts hid"(T8."H1NH2N" ("system statuts")) -> ()
                            }
                          }
                        }
                        frame #1 {
                          n510 = local read "H2 warning 2"() -> (w1893:bool)
                          n511 = local read "H2 warning"() -> (w1894:bool)
                          n512 = local read "H1 nominal 2"() -> (w1895:bool)
                          n513 = local read "H1 nominal"() -> (w1896:bool)
                          n514 = Or(x=w1894, y=w1893) -> (x .or. y?=w1892:bool)
                          n515 = Compound Arithmetic op=AND(w1896, w1895, w1892) -> (w1891:bool)
                          n516 = case shown="False" w1891 {
                            frame False {
                            }
                            frame True {
                              n517 = local write "system statuts hid"(T8."H1NH2W" ("system statuts")) -> ()
                            }
                          }
                        }
                        frame #2 {
                          n518 = local read "H1 nominal 2"() -> (w1903:bool)
                          n519 = local read "H1 nominal"() -> (w1904:bool)
                          n520 = local read "H2 alarm 2"() -> (w1901:bool)
                          n521 = local read "H2 alarm"() -> (w1902:bool)
                          n522 = Or(x=w1902, y=w1901) -> (x .or. y?=w1899:bool)
                          n523 = And(x=w1904, y=w1903) -> (x .and. y?=w1900:bool)
                          n524 = And(x=w1900, y=w1899) -> (x .and. y?=w1898:bool)
                          n525 = case shown="True" w1898 {
                            frame False {
                            }
                            frame True {
                              n526 = local write "system statuts hid"(T8."H1NH2A" ("system statuts")) -> ()
                            }
                          }
                        }
                        frame #3 {
                          n527 = local read "H1 alarm 2"() -> (w1914:bool)
                          n528 = local read "H1 alarm"() -> (w1915:bool)
                          n529 = local read "H2 nominal 2"() -> (w1917:bool)
                          n530 = local read "H1 warning 2"() -> (w1910:bool)
                          n531 = local read "H1 warning"() -> (w1911:bool)
                          n532 = local read "H2 nominal"() -> (w1916:bool)
                          n533 = Not(x=w1915) -> (.not. x?=w1913:bool)
                          n534 = Not(x=w1914) -> (.not. x?=w1912:bool)
                          n535 = Or(x=w1911, y=w1910) -> (x .or. y?=w1908:bool)
                          n536 = And(x=w1913, y=w1912) -> (x .and. y?=w1907:bool)
                          n537 = And(x=w1916, y=w1917) -> (x .and. y?=w1906:bool)
                          n538 = Compound Arithmetic op=AND(w1908, w1907, w1906) -> (w1909:bool)
                          n539 = case shown="True" w1909 {
                            frame False {
                            }
                            frame True {
                              n540 = local write "system statuts hid"(T8."H1WH2N" ("system statuts")) -> ()
                            }
                          }
                        }
                        frame #4 {
                          n541 = local read "H1 alarm 2"() -> (w1929:bool)
                          n542 = local read "H2 alarm 2"() -> (w1934:bool)
                          n543 = local read "H1 alarm"() -> (w1928:bool)
                          n544 = local read "H2 alarm"() -> (w1935:bool)
                          n545 = local read "H1 warning 2"() -> (w1925:bool)
                          n546 = local read "H2 warning 2"() -> (w1926:bool)
                          n547 = local read "H1 warning"() -> (w1924:bool)
                          n548 = local read "H2 warning"() -> (w1927:bool)
                          n549 = Not(x=w1928) -> (.not. x?=w1930:bool)
                          n550 = Not(x=w1929) -> (.not. x?=w1931:bool)
                          n551 = Not(x=w1935) -> (.not. x?=w1933:bool)
                          n552 = Not(x=w1934) -> (.not. x?=w1932:bool)
                          n553 = Or(x=w1924, y=w1925) -> (x .or. y?=w1922:bool)
                          n554 = Or(x=w1927, y=w1926) -> (x .or. y?=w1920:bool)
                          n555 = And(x=w1930, y=w1931) -> (x .and. y?=w1921:bool)
                          n556 = And(x=w1933, y=w1932) -> (x .and. y?=w1919:bool)
                          n557 = Compound Arithmetic op=AND(w1922, w1921, w1920, w1919) -> (w1923:bool)
                          n558 = case shown="True" w1923 {
                            frame False {
                            }
                            frame True {
                              n559 = local write "system statuts hid"(T8."H1WH2W" ("system statuts")) -> ()
                            }
                          }
                        }
                        frame #5 {
                          n560 = local read "H1 alarm 2"() -> (w1942:bool)
                          n561 = local read "H1 alarm"() -> (w1943:bool)
                          n562 = local read "H1 warning 2"() -> (w1945:bool)
                          n563 = local read "H1 warning"() -> (w1946:bool)
                          n564 = local read "H2 alarm 2"() -> (w1947:bool)
                          n565 = local read "H2 alarm"() -> (w1948:bool)
                          n566 = Not(x=w1943) -> (.not. x?=w1941:bool)
                          n567 = Not(x=w1942) -> (.not. x?=w1940:bool)
                          n568 = Or(x=w1946, y=w1945) -> (x .or. y?=w1939:bool)
                          n569 = Or(x=w1948, y=w1947) -> (x .or. y?=w1937:bool)
                          n570 = And(x=w1941, y=w1940) -> (x .and. y?=w1938:bool)
                          n571 = Compound Arithmetic op=AND(w1939, w1938, w1937) -> (w1944:bool)
                          n572 = case shown="True" w1944 {
                            frame False {
                            }
                            frame True {
                              n573 = local write "system statuts hid"(T8."H1WH2A" ("system statuts")) -> ()
                            }
                          }
                        }
                        frame #6 {
                          n574 = local read "H2 nominal 2"() -> (w1955:bool)
                          n575 = local read "H2 nominal"() -> (w1956:bool)
                          n576 = local read "H1 alarm 2"() -> (w1953:bool)
                          n577 = local read "H1 alarm"() -> (w1954:bool)
                          n578 = Or(x=w1954, y=w1953) -> (x .or. y?=w1951:bool)
                          n579 = And(x=w1956, y=w1955) -> (x .and. y?=w1950:bool)
                          n580 = And(x=w1951, y=w1950) -> (x .and. y?=w1952:bool)
                          n581 = case shown="True" w1952 {
                            frame False {
                            }
                            frame True {
                              n582 = local write "system statuts hid"(T8."H1AH2N" ("system statuts")) -> ()
                            }
                          }
                        }
                        frame #7 {
                          n583 = local read "H2 alarm 2"() -> (w1960:bool)
                          n584 = local read "H2 alarm"() -> (w1961:bool)
                          n585 = local read "H2 warning 2"() -> (w1966:bool)
                          n586 = local read "H2 warning"() -> (w1967:bool)
                          n587 = local read "H1 alarm 2"() -> (w1968:bool)
                          n588 = local read "H1 alarm"() -> (w1969:bool)
                          n589 = Not(x=w1961) -> (.not. x?=w1959:bool)
                          n590 = Not(x=w1960) -> (.not. x?=w1958:bool)
                          n591 = Or(x=w1969, y=w1968) -> (x .or. y?=w1964:bool)
                          n592 = Or(x=w1967, y=w1966) -> (x .or. y?=w1963:bool)
                          n593 = And(x=w1959, y=w1958) -> (x .and. y?=w1962:bool)
                          n594 = Compound Arithmetic op=AND(w1964, w1963, w1962) -> (w1965:bool)
                          n595 = case shown="True" w1965 {
                            frame False {
                            }
                            frame True {
                              n596 = local write "system statuts hid"(T8."H1AH2W" ("system statuts")) -> ()
                            }
                          }
                        }
                        frame #8 {
                          n597 = local read "H1 alarm 2"() -> (w1975:bool)
                          n598 = local read "H2 alarm 2"() -> (w1974:bool)
                          n599 = local read "H1 alarm"() -> (w1976:bool)
                          n600 = local read "H2 alarm"() -> (w1973:bool)
                          n601 = Or(x=w1976, y=w1975) -> (x .or. y?=w1971:bool)
                          n602 = Or(x=w1973, y=w1974) -> (x .or. y?=w1972:bool)
                          n603 = And(x=w1971, y=w1972) -> (x .and. y?=w1977:bool)
                          n604 = case shown="True" w1977 {
                            frame False {
                            }
                            frame True {
                              n605 = local write "system statuts hid"(T8."H1AH2A" ("system statuts")) -> ()
                            }
                          }
                        }
                      }
                    }
                    frame #1 {
                      n606 = local read "system statuts hid"() -> (w1981:T8)
                      n607 = Not Equal?(x=w1981, y=w1979) -> (x != y?=w1980:bool)
                      n608 = case shown="True" w1980 {
                        tunnel: w1981 -> [_ w1983]
                        frame False {
                        }
                        frame True {
                          n609 = local read "Enable data logging of all events"() -> (w1982:bool)
                          n610 = case shown="True" w1982 {
                            tunnel: w1983 -> [_ w1984]
                            frame False {
                            }
                            frame True {
                              n611 = stacked-sequence {
                                tunnel: w1984 -> [_ w1987 _ _ _]
                                frame #0 {
                                n612 = local read "Number of data log entries hid"() -> (w1986:u32)
                                n613 = Increment(x=w1986) -> (x+1=w1985:u32)
                                n614 = local write "Number of data log entries hid"(w1985) -> ()
                                }
                                frame #1 {
                                n615 = case shown="\"H1AH2A\"" w1987 {
                                frame "H1NH2N", Default {
                                w1994 = "\r\n"
                                n616 = local read "H1 online"() -> (w2011:bool)
                                n617 = local read "H2 online"() -> (w2012:bool)
                                n618 = local read "Number of data log entries hid"() -> (w1988:u32)
                                n619 = local read "H1 UPH warning limit hid"() -> (w2007:dbl)
                                n620 = local read "H2 UPH warning limit hid"() -> (w2009:dbl)
                                n621 = local read "YieldMon"() -> (w1992:cluster{i32, i32, i32, i32})
                                n622 = local read "H2  low yield warning"() -> (w2008:dbl)
                                n623 = local read "H1 low yield warning"() -> (w2006:dbl)
                                n624 = local read "H1 UPH"() -> (w2000:cluster{u32, u32})
                                n625 = local read "H2 UPH"() -> (w1998:cluster{u32, u32})
                                n626 = local read "YieldMon"() -> (w1990:cluster{i32, i32, i32, i32})
                                n627 = case shown="True" w2011 {
                                tunnel: ["H1 Off-Line" "H1 On-Line"] -> w2013
                                frame False {
                                }
                                frame True {
                                }
                                }
                                n628 = case shown="True" w2012 {
                                tunnel: ["H2 Off-Line" "H2 On-Line"] -> w2022
                                frame False {
                                }
                                frame True {
                                }
                                }
                                n629 = Unbundle(w1992) -> (w1991:i32)  [unwired: 3 out]
                                n630 = Unbundle(w2000) -> (w1999:u32)  [unwired: 1 out]
                                n631 = Unbundle(w1990) -> (w1989:i32)  [unwired: 3 out]
                                n632 = Unbundle(w1998) -> (w1997:u32)  [unwired: 1 out]
                                n633 = local read "Data log path and filename"() -> (w1996:path)
                                n634 = Number To Decimal String(number=w2006) -> (decimal integer string=w2015:string)  [unwired: 1 in]
                                n635 = Number To Decimal String(number=w1991) -> (decimal integer string=w2017:string)  [unwired: 1 in]
                                n636 = Number To Decimal String(number=w2007) -> (decimal integer string=w2019:string)  [unwired: 1 in]
                                n637 = Number To Decimal String(number=w1999) -> (decimal integer string=w2021:string)  [unwired: 1 in]
                                n638 = Number To Decimal String(number=w2008) -> (decimal integer string=w2024:string)  [unwired: 1 in]
                                n639 = Number To Decimal String(number=w1989) -> (decimal integer string=w2026:string)  [unwired: 1 in]
                                n640 = Number To Decimal String(number=w2009) -> (decimal integer string=w2028:string)  [unwired: 1 in]
                                n641 = Number To Decimal String(number=w1997) -> (decimal integer string=w2030:string)  [unwired: 1 in]
                                n642 = Number To Decimal String(number=w1988) -> (decimal integer string=w1993:string)  [unwired: 1 in]
                                n643 = Get Date/Time String(want seconds? (F)=TRUE) -> (date string=w2004:string, time string=w2005:string)  [unwired: 2 in]
                                n644 = Concatenate Strings(w1993, w1994, w2004, "   " ("string"), w2005, w1994, "H1 Nominal, H2 Nominal", w1994, w2013, w1994, "H1 Low Yield Warning Limit: ", w2015, ", H1 yield = ", w2017, w1994, "H1 Low UPH Warning Limit: ", w2019, ", H1 UPH = ", w2021, w1994, w2022, w1994, "H2 Low Yield Warning Limit: ", w2024, ", H2 yield = ", w2026, w1994, "H2 Low UPH Warning Limit: ", w2028, ", H2 UPH = ", w2030, w1994, w1994) -> (w2002:string)
                                n645 = call "SentinelDatalog.vi"("operation (0:open)"=T9."open", "String"=w2002, "data log path"=w1996) -> ()  [unwired: 8 in, 1 out]
                                }
                                frame "H1NH2W" {
                                w2040 = "\r\n"
                                n646 = local read "H1 online"() -> (w2058:bool)
                                n647 = local read "H2 online"() -> (w2059:bool)
                                n648 = local read "H1 UPH warning limit hid"() -> (w2054:dbl)
                                n649 = local read "H2 UPH warning limit hid"() -> (w2056:dbl)
                                n650 = local read "YieldMon"() -> (w2039:cluster{i32, i32, i32, i32})
                                n651 = local read "H2  low yield warning"() -> (w2055:dbl)
                                n652 = local read "H1 low yield warning"() -> (w2053:dbl)
                                n653 = local read "H1 UPH"() -> (w2047:cluster{u32, u32})
                                n654 = local read "H2 UPH"() -> (w2045:cluster{u32, u32})
                                n655 = local read "YieldMon"() -> (w2037:cluster{i32, i32, i32, i32})
                                n656 = local read "Number of data log entries hid"() -> (w2035:u32)
                                n657 = case shown="True" w2058 {
                                tunnel: ["H1 Off-Line" "H1 On-Line"] -> w2060
                                frame False {
                                }
                                frame True {
                                }
                                }
                                n658 = case shown="True" w2059 {
                                tunnel: ["H2 Off-Line" "H2 On-Line"] -> w2069
                                frame False {
                                }
                                frame True {
                                }
                                }
                                n659 = Unbundle(w2037) -> (w2036:i32)  [unwired: 3 out]
                                n660 = Unbundle(w2047) -> (w2046:u32)  [unwired: 1 out]
                                n661 = Unbundle(w2039) -> (w2038:i32)  [unwired: 3 out]
                                n662 = Unbundle(w2045) -> (w2044:u32)  [unwired: 1 out]
                                n663 = Number To Decimal String(number=w2053) -> (decimal integer string=w2062:string)  [unwired: 1 in]
                                n664 = Number To Decimal String(number=w2036) -> (decimal integer string=w2064:string)  [unwired: 1 in]
                                n665 = Number To Decimal String(number=w2054) -> (decimal integer string=w2066:string)  [unwired: 1 in]
                                n666 = Number To Decimal String(number=w2046) -> (decimal integer string=w2068:string)  [unwired: 1 in]
                                n667 = Number To Decimal String(number=w2055) -> (decimal integer string=w2071:string)  [unwired: 1 in]
                                n668 = Number To Decimal String(number=w2038) -> (decimal integer string=w2073:string)  [unwired: 1 in]
                                n669 = Number To Decimal String(number=w2056) -> (decimal integer string=w2075:string)  [unwired: 1 in]
                                n670 = Number To Decimal String(number=w2044) -> (decimal integer string=w2077:string)  [unwired: 1 in]
                                n671 = Number To Decimal String(number=w2035) -> (decimal integer string=w2041:string)  [unwired: 1 in]
                                n672 = local read "Data log path and filename"() -> (w2043:path)
                                n673 = Get Date/Time String(want seconds? (F)=TRUE) -> (date string=w2051:string, time string=w2052:string)  [unwired: 2 in]
                                n674 = Concatenate Strings(w2041, w2040, w2051, "   " ("string"), w2052, w2040, "H1 Nominal, H2 Warning", w2040, w2060, w2040, "H1 Low Yield Warning Limit: ", w2062, ", H1 yield = ", w2064, w2040, "H1 Low UPH Warning Limit: ", w2066, ", H1 UPH = ", w2068, w2040, w2069, w2040, "H2 Low Yield Warning Limit: ", w2071, ", H2 yield = ", w2073, w2040, "H2 Low UPH Warning Limit: ", w2075, ", H2 UPH = ", w2077, w2040, w2040) -> (w2049:string)
                                n675 = call "SentinelDatalog.vi"("operation (0:open)"=T9."open", "String"=w2049, "data log path"=w2043) -> ()  [unwired: 8 in, 1 out]
                                }
                                frame "H1NH2A" {
                                w2088 = "\r\n"
                                n676 = local read "H1 online"() -> (w2105:bool)
                                n677 = local read "H2 online"() -> (w2106:bool)
                                n678 = local read "Number of data log entries hid"() -> (w2082:u32)
                                n679 = local read "H1 UPH warning limit hid"() -> (w2101:dbl)
                                n680 = local read "H1 low yield warning"() -> (w2100:dbl)
                                n681 = local read "H2 UPH alarm limit hid"() -> (w2103:dbl)
                                n682 = local read "YieldMon"() -> (w2086:cluster{i32, i32, i32, i32})
                                n683 = local read "H1 UPH"() -> (w2094:cluster{u32, u32})
                                n684 = local read "H2 low yield alarm"() -> (w2102:dbl)
                                n685 = local read "H2 UPH"() -> (w2093:cluster{u32, u32})
                                n686 = local read "YieldMon"() -> (w2084:cluster{i32, i32, i32, i32})
                                n687 = case shown="True" w2105 {
                                tunnel: ["H1 Off-Line" "H1 On-Line"] -> w2107
                                frame False {
                                }
                                frame True {
                                }
                                }
                                n688 = case shown="True" w2106 {
                                tunnel: ["H2 Off-Line" "H2 On-Line"] -> w2116
                                frame False {
                                }
                                frame True {
                                }
                                }
                                n689 = Number To Decimal String(number=w2082) -> (decimal integer string=w2087:string)  [unwired: 1 in]
                                n690 = Unbundle(w2086) -> (w2085:i32)  [unwired: 3 out]
                                n691 = Unbundle(w2094) -> (w2091:u32)  [unwired: 1 out]
                                n692 = Unbundle(w2084) -> (w2083:i32)  [unwired: 3 out]
                                n693 = Unbundle(w2093) -> (w2092:u32)  [unwired: 1 out]
                                n694 = Number To Decimal String(number=w2100) -> (decimal integer string=w2109:string)  [unwired: 1 in]
                                n695 = Number To Decimal String(number=w2085) -> (decimal integer string=w2111:string)  [unwired: 1 in]
                                n696 = Number To Decimal String(number=w2101) -> (decimal integer string=w2113:string)  [unwired: 1 in]
                                n697 = Number To Decimal String(number=w2091) -> (decimal integer string=w2115:string)  [unwired: 1 in]
                                n698 = Number To Decimal String(number=w2102) -> (decimal integer string=w2118:string)  [unwired: 1 in]
                                n699 = Number To Decimal String(number=w2083) -> (decimal integer string=w2120:string)  [unwired: 1 in]
                                n700 = Number To Decimal String(number=w2103) -> (decimal integer string=w2122:string)  [unwired: 1 in]
                                n701 = Number To Decimal String(number=w2092) -> (decimal integer string=w2124:string)  [unwired: 1 in]
                                n702 = local read "Data log path and filename"() -> (w2090:path)
                                n703 = Get Date/Time String(want seconds? (F)=TRUE) -> (date string=w2098:string, time string=w2099:string)  [unwired: 2 in]
                                n704 = Concatenate Strings(w2087, w2088, w2098, "   " ("string"), w2099, w2088, "H1 Nominal, H2 Alarming", w2088, w2107, w2088, "H1 Low Yield Warning Limit: ", w2109, ", H1 yield = ", w2111, w2088, "H1 Low UPH Warning Limit: ", w2113, ", H1 UPH = ", w2115, w2088, w2116, w2088, "H2 Low Yield Alarm Limit: ", w2118, ", H2 yield = ", w2120, w2088, "H2 Low UPH Alarm Limit: ", w2122, ", H2 UPH = ", w2124, w2088, w2088) -> (w2096:string)
                                n705 = call "SentinelDatalog.vi"("operation (0:open)"=T9."open", "String"=w2096, "data log path"=w2090) -> ()  [unwired: 8 in, 1 out]
                                }
                                frame "H1WH2N" {
                                w2135 = "\r\n"
                                n706 = local read "H1 online"() -> (w2153:bool)
                                n707 = local read "H2 online"() -> (w2154:bool)
                                n708 = local read "H1 UPH warning limit hid"() -> (w2149:dbl)
                                n709 = local read "H2 UPH warning limit hid"() -> (w2151:dbl)
                                n710 = local read "H2  low yield warning"() -> (w2150:dbl)
                                n711 = local read "H1 low yield warning"() -> (w2148:dbl)
                                n712 = local read "H1 UPH"() -> (w2141:cluster{u32, u32})
                                n713 = local read "H2 UPH"() -> (w2140:cluster{u32, u32})
                                n714 = local read "YieldMon"() -> (w2133:cluster{i32, i32, i32, i32})
                                n715 = local read "YieldMon"() -> (w2131:cluster{i32, i32, i32, i32})
                                n716 = local read "Number of data log entries hid"() -> (w2129:u32)
                                n717 = case shown="True" w2153 {
                                tunnel: ["H1 Off-Line" "H1 On-Line"] -> w2142
                                frame False {
                                }
                                frame True {
                                }
                                }
                                n718 = case shown="True" w2154 {
                                tunnel: ["H2 Off-Line" "H2 On-Line"] -> w2163
                                frame False {
                                }
                                frame True {
                                }
                                }
                                n719 = Unbundle(w2133) -> (w2132:i32)  [unwired: 3 out]
                                n720 = Unbundle(w2141) -> (w2138:u32)  [unwired: 1 out]
                                n721 = Unbundle(w2131) -> (w2130:i32)  [unwired: 3 out]
                                n722 = Unbundle(w2140) -> (w2139:u32)  [unwired: 1 out]
                                n723 = Number To Decimal String(number=w2148) -> (decimal integer string=w2156:string)  [unwired: 1 in]
                                n724 = Number To Decimal String(number=w2132) -> (decimal integer string=w2158:string)  [unwired: 1 in]
                                n725 = Number To Decimal String(number=w2149) -> (decimal integer string=w2160:string)  [unwired: 1 in]
                                n726 = Number To Decimal String(number=w2138) -> (decimal integer string=w2162:string)  [unwired: 1 in]
                                n727 = Number To Decimal String(number=w2150) -> (decimal integer string=w2165:string)  [unwired: 1 in]
                                n728 = Number To Decimal String(number=w2130) -> (decimal integer string=w2167:string)  [unwired: 1 in]
                                n729 = Number To Decimal String(number=w2151) -> (decimal integer string=w2169:string)  [unwired: 1 in]
                                n730 = Number To Decimal String(number=w2139) -> (decimal integer string=w2171:string)  [unwired: 1 in]
                                n731 = local read "Data log path and filename"() -> (w2137:path)
                                n732 = Number To Decimal String(number=w2129) -> (decimal integer string=w2134:string)  [unwired: 1 in]
                                n733 = Get Date/Time String(want seconds? (F)=TRUE) -> (date string=w2146:string, time string=w2147:string)  [unwired: 2 in]
                                n734 = Concatenate Strings(w2134, w2135, w2146, "   " ("string"), w2147, w2135, "H1 Warning, H2 Nominal", w2135, w2142, w2135, "H1 Low Yield Warning Limit: ", w2156, ", H1 yield = ", w2158, w2135, "H1 Low UPH Warning Limit: ", w2160, ", H1 UPH = ", w2162, w2135, w2163, w2135, "H2 Low Yield Warning Limit: ", w2165, ", H2 yield = ", w2167, w2135, "H2 Low UPH Warning Limit: ", w2169, ", H2 UPH = ", w2171, w2135, w2135) -> (w2144:string)
                                n735 = call "SentinelDatalog.vi"("operation (0:open)"=T9."open", "String"=w2144, "data log path"=w2137) -> ()  [unwired: 8 in, 1 out]
                                }
                                frame "H1WH2W" {
                                w2181 = "\r\n"
                                w2189 = "\r\n"
                                n736 = local read "H1 online"() -> (w2200:bool)
                                n737 = local read "H2 online"() -> (w2201:bool)
                                n738 = local read "H1 UPH warning limit hid"() -> (w2196:dbl)
                                n739 = local read "H2 UPH warning limit hid"() -> (w2198:dbl)
                                n740 = local read "H2  low yield warning"() -> (w2197:dbl)
                                n741 = local read "H1 low yield warning"() -> (w2195:dbl)
                                n742 = local read "H1 UPH"() -> (w2188:cluster{u32, u32})
                                n743 = local read "H2 UPH"() -> (w2187:cluster{u32, u32})
                                n744 = local read "YieldMon"() -> (w2180:cluster{i32, i32, i32, i32})
                                n745 = local read "YieldMon"() -> (w2178:cluster{i32, i32, i32, i32})
                                n746 = case shown="True" w2200 {
                                tunnel: ["H1 Off-Line" "H1 On-Line"] -> w2202
                                frame False {
                                }
                                frame True {
                                }
                                }
                                n747 = case shown="True" w2201 {
                                tunnel: ["H2 Off-Line" "H2 On-Line"] -> w2211
                                frame False {
                                }
                                frame True {
                                }
                                }
                                n748 = local read "Number of data log entries hid"() -> (w2176:u32)
                                n749 = Unbundle(w2180) -> (w2179:i32)  [unwired: 3 out]
                                n750 = Unbundle(w2188) -> (w2186:u32)  [unwired: 1 out]
                                n751 = Unbundle(w2178) -> (w2177:i32)  [unwired: 3 out]
                                n752 = Unbundle(w2187) -> (w2185:u32)  [unwired: 1 out]
                                n753 = Number To Decimal String(number=w2195) -> (decimal integer string=w2204:string)  [unwired: 1 in]
                                n754 = Number To Decimal String(number=w2179) -> (decimal integer string=w2206:string)  [unwired: 1 in]
                                n755 = Number To Decimal String(number=w2196) -> (decimal integer string=w2208:string)  [unwired: 1 in]
                                n756 = Number To Decimal String(number=w2186) -> (decimal integer string=w2210:string)  [unwired: 1 in]
                                n757 = Number To Decimal String(number=w2197) -> (decimal integer string=w2213:string)  [unwired: 1 in]
                                n758 = Number To Decimal String(number=w2177) -> (decimal integer string=w2215:string)  [unwired: 1 in]
                                n759 = Number To Decimal String(number=w2198) -> (decimal integer string=w2217:string)  [unwired: 1 in]
                                n760 = Number To Decimal String(number=w2185) -> (decimal integer string=w2219:string)  [unwired: 1 in]
                                n761 = local read "Data log path and filename"() -> (w2184:path)
                                n762 = Get Date/Time String(want seconds? (F)=TRUE) -> (date string=w2193:string, time string=w2194:string)  [unwired: 2 in]
                                n763 = Number To Decimal String(number=w2176) -> (decimal integer string=w2182:string)  [unwired: 1 in]
                                n764 = Concatenate Strings(w2182, w2181, w2193, "   " ("string"), w2194, w2181, "H1 Warning, H2 Warning", w2181, w2202, w2181, "H1 Low Yield Warning Limit: ", w2204, ", H1 yield = ", w2206, w2189, "H1 Low UPH Warning Limit: ", w2208, ", H1 UPH = ", w2210, w2189, w2211, w2189, "H2 Low Yield Warning Limit: ", w2213, ", H2 yield = ", w2215, w2189, "H2 Low UPH Warning Limit: ", w2217, ", H2 UPH = ", w2219, w2189, w2189) -> (w2191:string)
                                n765 = call "SentinelDatalog.vi"("operation (0:open)"=T9."open", "String"=w2191, "data log path"=w2184) -> ()  [unwired: 8 in, 1 out]
                                }
                                frame "H1WH2A" {
                                w2230 = "\r\n"
                                n766 = local read "H1 online"() -> (w2247:bool)
                                n767 = local read "H2 online"() -> (w2248:bool)
                                n768 = local read "H1 UPH warning limit hid"() -> (w2243:dbl)
                                n769 = local read "H1 low yield warning"() -> (w2242:dbl)
                                n770 = local read "H2 UPH alarm limit hid"() -> (w2245:dbl)
                                n771 = local read "H1 UPH"() -> (w2236:cluster{u32, u32})
                                n772 = local read "H2 low yield alarm"() -> (w2244:dbl)
                                n773 = local read "H2 UPH"() -> (w2235:cluster{u32, u32})
                                n774 = local read "YieldMon"() -> (w2226:cluster{i32, i32, i32, i32})
                                n775 = local read "YieldMon"() -> (w2228:cluster{i32, i32, i32, i32})
                                n776 = local read "Number of data log entries hid"() -> (w2224:u32)
                                n777 = case shown="True" w2247 {
                                tunnel: ["H1 Off-Line" "H1 On-Line"] -> w2249
                                frame False {
                                }
                                frame True {
                                }
                                }
                                n778 = case shown="True" w2248 {
                                tunnel: ["H2 Off-Line" "H2 On-Line"] -> w2258
                                frame False {
                                }
                                frame True {
                                }
                                }
                                n779 = Unbundle(w2226) -> (w2225:i32)  [unwired: 3 out]
                                n780 = Unbundle(w2236) -> (w2234:u32)  [unwired: 1 out]
                                n781 = Unbundle(w2228) -> (w2227:i32)  [unwired: 3 out]
                                n782 = Unbundle(w2235) -> (w2233:u32)  [unwired: 1 out]
                                n783 = Number To Decimal String(number=w2242) -> (decimal integer string=w2251:string)  [unwired: 1 in]
                                n784 = Number To Decimal String(number=w2225) -> (decimal integer string=w2253:string)  [unwired: 1 in]
                                n785 = Number To Decimal String(number=w2243) -> (decimal integer string=w2255:string)  [unwired: 1 in]
                                n786 = Number To Decimal String(number=w2234) -> (decimal integer string=w2257:string)  [unwired: 1 in]
                                n787 = Number To Decimal String(number=w2244) -> (decimal integer string=w2260:string)  [unwired: 1 in]
                                n788 = Number To Decimal String(number=w2227) -> (decimal integer string=w2262:string)  [unwired: 1 in]
                                n789 = Number To Decimal String(number=w2245) -> (decimal integer string=w2264:string)  [unwired: 1 in]
                                n790 = Number To Decimal String(number=w2233) -> (decimal integer string=w2266:string)  [unwired: 1 in]
                                n791 = local read "Data log path and filename"() -> (w2232:path)
                                n792 = Get Date/Time String(want seconds? (F)=TRUE) -> (date string=w2240:string, time string=w2241:string)  [unwired: 2 in]
                                n793 = Number To Decimal String(number=w2224) -> (decimal integer string=w2229:string)  [unwired: 1 in]
                                n794 = Concatenate Strings(w2229, w2230, w2240, "   " ("string"), w2241, w2230, "H1 Warning, H2 Alarming", w2230, w2249, w2230, "H1 Low Yield Warning Limit: ", w2251, ", H1 yield = ", w2253, w2230, "H1 Low UPH Warning Limit: ", w2255, ", H1 UPH = ", w2257, w2230, w2258, w2230, "H2 Low Yield Alarm Limit: ", w2260, ", H2 yield = ", w2262, w2230, "H2 Low UPH Alarm Limit: ", w2264, ", H2 UPH = ", w2266, w2230, w2230) -> (w2238:string)
                                n795 = call "SentinelDatalog.vi"("operation (0:open)"=T9."open", "String"=w2238, "data log path"=w2232) -> ()  [unwired: 8 in, 1 out]
                                }
                                frame "H1AH2N" {
                                w2277 = "\r\n"
                                n796 = local read "H1 online"() -> (w2294:bool)
                                n797 = local read "H2 online"() -> (w2295:bool)
                                n798 = local read "H2 UPH warning limit hid"() -> (w2292:dbl)
                                n799 = local read "H2  low yield warning"() -> (w2291:dbl)
                                n800 = local read "H1 UPH alarm limit hid"() -> (w2290:dbl)
                                n801 = local read "H1 low yield alarm"() -> (w2289:dbl)
                                n802 = local read "H1 UPH"() -> (w2283:cluster{u32, u32})
                                n803 = local read "H2 UPH"() -> (w2282:cluster{u32, u32})
                                n804 = local read "YieldMon"() -> (w2275:cluster{i32, i32, i32, i32})
                                n805 = local read "YieldMon"() -> (w2273:cluster{i32, i32, i32, i32})
                                n806 = case shown="True" w2294 {
                                tunnel: ["H1 Off-Line" "H1 On-Line"] -> w2296
                                frame False {
                                }
                                frame True {
                                }
                                }
                                n807 = case shown="False" w2295 {
                                tunnel: ["H2 Off-Line" "H2 On-Line"] -> w2305
                                frame False {
                                }
                                frame True {
                                }
                                }
                                n808 = local read "Number of data log entries hid"() -> (w2271:u32)
                                n809 = Unbundle(w2275) -> (w2274:i32)  [unwired: 3 out]
                                n810 = Unbundle(w2283) -> (w2281:u32)  [unwired: 1 out]
                                n811 = Unbundle(w2273) -> (w2272:i32)  [unwired: 3 out]
                                n812 = Unbundle(w2282) -> (w2280:u32)  [unwired: 1 out]
                                n813 = Number To Decimal String(number=w2289) -> (decimal integer string=w2298:string)  [unwired: 1 in]
                                n814 = Number To Decimal String(number=w2274) -> (decimal integer string=w2300:string)  [unwired: 1 in]
                                n815 = Number To Decimal String(number=w2290) -> (decimal integer string=w2302:string)  [unwired: 1 in]
                                n816 = Number To Decimal String(number=w2281) -> (decimal integer string=w2304:string)  [unwired: 1 in]
                                n817 = Number To Decimal String(number=w2291) -> (decimal integer string=w2307:string)  [unwired: 1 in]
                                n818 = Number To Decimal String(number=w2272) -> (decimal integer string=w2309:string)  [unwired: 1 in]
                                n819 = Number To Decimal String(number=w2292) -> (decimal integer string=w2311:string)  [unwired: 1 in]
                                n820 = Number To Decimal String(number=w2280) -> (decimal integer string=w2313:string)  [unwired: 1 in]
                                n821 = local read "Data log path and filename"() -> (w2279:path)
                                n822 = Get Date/Time String(want seconds? (F)=TRUE) -> (date string=w2287:string, time string=w2288:string)  [unwired: 2 in]
                                n823 = Number To Decimal String(number=w2271) -> (decimal integer string=w2276:string)  [unwired: 1 in]
                                n824 = Concatenate Strings(w2276, w2277, w2287, "   " ("string"), w2288, w2277, "H1 Alarming, H2 Nominal", w2277, w2296, w2277, "H1 Low Yield Alarm Limit: ", w2298, ", H1 yield = ", w2300, w2277, "H1 Low UPH Alarm Limit: ", w2302, ", H1 UPH = ", w2304, w2277, w2305, w2277, "H2 Low Yield Warning Limit: ", w2307, ", H2 yield = ", w2309, w2277, "H2 Low UPH Warning Limit: ", w2311, ", H2 UPH = ", w2313, w2277, w2277) -> (w2285:string)
                                n825 = call "SentinelDatalog.vi"("operation (0:open)"=T9."open", "String"=w2285, "data log path"=w2279) -> ()  [unwired: 8 in, 1 out]
                                }
                                frame "H1AH2W" {
                                w2324 = "\r\n"
                                n826 = local read "H1 online"() -> (w2341:bool)
                                n827 = local read "H2 online"() -> (w2342:bool)
                                n828 = local read "H2 UPH warning limit hid"() -> (w2339:dbl)
                                n829 = local read "H2  low yield warning"() -> (w2338:dbl)
                                n830 = local read "H1 UPH alarm limit hid"() -> (w2337:dbl)
                                n831 = local read "H1 low yield alarm"() -> (w2336:dbl)
                                n832 = local read "H1 UPH"() -> (w2330:cluster{u32, u32})
                                n833 = local read "H2 UPH"() -> (w2329:cluster{u32, u32})
                                n834 = local read "YieldMon"() -> (w2322:cluster{i32, i32, i32, i32})
                                n835 = local read "YieldMon"() -> (w2320:cluster{i32, i32, i32, i32})
                                n836 = case shown="True" w2341 {
                                tunnel: ["H1 Off-Line" "H1 On-Line"] -> w2343
                                frame False {
                                }
                                frame True {
                                }
                                }
                                n837 = case shown="True" w2342 {
                                tunnel: ["H2 Off-Line" "H2 On-Line"] -> w2352
                                frame False {
                                }
                                frame True {
                                }
                                }
                                n838 = local read "Number of data log entries hid"() -> (w2318:u32)
                                n839 = Unbundle(w2322) -> (w2321:i32)  [unwired: 3 out]
                                n840 = Unbundle(w2330) -> (w2328:u32)  [unwired: 1 out]
                                n841 = Unbundle(w2320) -> (w2319:i32)  [unwired: 3 out]
                                n842 = Unbundle(w2329) -> (w2327:u32)  [unwired: 1 out]
                                n843 = Number To Decimal String(number=w2336) -> (decimal integer string=w2345:string)  [unwired: 1 in]
                                n844 = Number To Decimal String(number=w2321) -> (decimal integer string=w2347:string)  [unwired: 1 in]
                                n845 = Number To Decimal String(number=w2337) -> (decimal integer string=w2349:string)  [unwired: 1 in]
                                n846 = Number To Decimal String(number=w2328) -> (decimal integer string=w2351:string)  [unwired: 1 in]
                                n847 = Number To Decimal String(number=w2338) -> (decimal integer string=w2354:string)  [unwired: 1 in]
                                n848 = Number To Decimal String(number=w2319) -> (decimal integer string=w2356:string)  [unwired: 1 in]
                                n849 = Number To Decimal String(number=w2339) -> (decimal integer string=w2358:string)  [unwired: 1 in]
                                n850 = Number To Decimal String(number=w2327) -> (decimal integer string=w2360:string)  [unwired: 1 in]
                                n851 = local read "Data log path and filename"() -> (w2326:path)
                                n852 = Get Date/Time String(want seconds? (F)=TRUE) -> (date string=w2334:string, time string=w2335:string)  [unwired: 2 in]
                                n853 = Number To Decimal String(number=w2318) -> (decimal integer string=w2323:string)  [unwired: 1 in]
                                n854 = Concatenate Strings(w2323, w2324, w2334, "   " ("string"), w2335, w2324, "H1 Alarming, H2 Warning", w2324, w2343, w2324, "H1 Low Yield Alarm Limit: ", w2345, ", H1 yield = ", w2347, w2324, "H1 Low UPH Alarm Limit: ", w2349, ", H1 UPH = ", w2351, w2324, w2352, w2324, "H2 Low Yield Warning Limit: ", w2354, ", H2 yield = ", w2356, w2324, "H2 Low UPH Warning Limit: ", w2358, ", H2 UPH = ", w2360, w2324) -> (w2332:string)
                                n855 = call "SentinelDatalog.vi"("operation (0:open)"=T9."open", "String"=w2332, "data log path"=w2326) -> ()  [unwired: 8 in, 1 out]
                                }
                                frame "H1AH2A" {
                                w2371 = "\r\n"
                                n856 = local read "H1 online"() -> (w2388:bool)
                                n857 = local read "H2 online"() -> (w2389:bool)
                                n858 = local read "H1 UPH alarm limit hid"() -> (w2384:dbl)
                                n859 = local read "H2 UPH alarm limit hid"() -> (w2386:dbl)
                                n860 = local read "H1 low yield alarm"() -> (w2383:dbl)
                                n861 = local read "H1 UPH"() -> (w2377:cluster{u32, u32})
                                n862 = local read "H2 low yield alarm"() -> (w2385:dbl)
                                n863 = local read "H2 UPH"() -> (w2376:cluster{u32, u32})
                                n864 = local read "YieldMon"() -> (w2369:cluster{i32, i32, i32, i32})
                                n865 = local read "YieldMon"() -> (w2368:cluster{i32, i32, i32, i32})
                                n866 = case shown="True" w2388 {
                                tunnel: ["H1 Off-Line" "H1 On-Line"] -> w2390
                                frame False {
                                }
                                frame True {
                                }
                                }
                                n867 = case shown="True" w2389 {
                                tunnel: ["H2 Off-Line" "H2 On-Line"] -> w2399
                                frame False {
                                }
                                frame True {
                                }
                                }
                                n868 = local read "Number of data log entries hid"() -> (w2365:u32)
                                n869 = Unbundle(w2369) -> (w2366:i32)  [unwired: 3 out]
                                n870 = Unbundle(w2377) -> (w2375:u32)  [unwired: 1 out]
                                n871 = Unbundle(w2368) -> (w2367:i32)  [unwired: 3 out]
                                n872 = Unbundle(w2376) -> (w2374:u32)  [unwired: 1 out]
                                n873 = Number To Decimal String(number=w2383) -> (decimal integer string=w2392:string)  [unwired: 1 in]
                                n874 = Number To Decimal String(number=w2366) -> (decimal integer string=w2394:string)  [unwired: 1 in]
                                n875 = Number To Decimal String(number=w2384) -> (decimal integer string=w2396:string)  [unwired: 1 in]
                                n876 = Number To Decimal String(number=w2375) -> (decimal integer string=w2398:string)  [unwired: 1 in]
                                n877 = Number To Decimal String(number=w2385) -> (decimal integer string=w2401:string)  [unwired: 1 in]
                                n878 = Number To Decimal String(number=w2367) -> (decimal integer string=w2403:string)  [unwired: 1 in]
                                n879 = Number To Decimal String(number=w2386) -> (decimal integer string=w2405:string)  [unwired: 1 in]
                                n880 = Number To Decimal String(number=w2374) -> (decimal integer string=w2407:string)  [unwired: 1 in]
                                n881 = local read "Data log path and filename"() -> (w2373:path)
                                n882 = Get Date/Time String(want seconds? (F)=TRUE) -> (date string=w2381:string, time string=w2382:string)  [unwired: 2 in]
                                n883 = Number To Decimal String(number=w2365) -> (decimal integer string=w2370:string)  [unwired: 1 in]
                                n884 = Concatenate Strings(w2370, w2371, w2381, "   " ("string"), w2382, w2371, "H1 Alarming, H2 Alarming", w2371, w2390, w2371, "H1 Low Yield Alarm Limit: ", w2392, ", H1 yield = ", w2394, w2371, "H1 Low UPH Alarm Limit: ", w2396, ", H1 UPH = ", w2398, w2371, w2399, w2371, "H2 Low Yield Alarm Limit: ", w2401, ", H2 yield = ", w2403, w2371, "H2 Low UPH Alarm Limit: ", w2405, ", H2 UPH = ", w2407, w2371, w2371) -> (w2379:string)
                                n885 = call "SentinelDatalog.vi"("operation (0:open)"=T9."open", "String"=w2379, "data log path"=w2373) -> ()  [unwired: 8 in, 1 out]
                                }
                                }
                                }
                                frame #2 {
                                n886 = Wait (ms)(milliseconds to wait=u32 100) -> ()  [unwired: 1 out]
                                }
                                frame #3 {
                                n887 = local read "Enable electronic notification of alarms"() -> (w2413:bool)
                                n888 = case shown="True" w2413 {
                                frame False {
                                }
                                frame True {
                                n889 = stacked-sequence {
                                frame #0 {
                                # "Email"
                                n890 = local read "Enable email notification"() -> (w2416:bool)
                                n891 = local read "Number of email alerts"() -> (w2415:u32)
                                n892 = Increment(x=w2415) -> (x+1=w2414:u32)
                                n893 = local write "Number of email alerts"(w2414) -> ()
                                n894 = case shown="True" w2416 {
                                frame False {
                                }
                                frame True {
                                n895 = flat-sequence {
                                tunnel: [w2423] -> w2418
                                tunnel: [w2431] -> w2417
                                tunnel: w2418 -> [w2431]
                                tunnel: w2417 -> [w2432]
                                frame #0 {
                                n896 = local read "Data log path and filename"() -> (w2428:path)
                                n897 = local read "Number of email alerts"() -> (w2422:u32)
                                n898 = Number To Decimal String(number=w2422) -> (decimal integer string=w2421:string)  [unwired: 1 in]
                                n899 = Strip Path(path=w2428) -> (stripped path=w2426:path, name=w2420:string)
                                n900 = Path To String(path=w2426) -> (string=w2425:string)
                                n901 = Concatenate Strings(w2425, "\\sent_#" ("string"), w2421, "_" ("string"), w2420) -> (w2429:string)
                                n902 = String To Path(string=w2429) -> (path=w2424:path)
                                n903 = Copy(10:w2424, 11:w2428) -> (3:w2423:path)  [unwired: 3 in, 2 out]
                                }
                                frame #1 {
                                n904 = Wait (ms)(milliseconds to wait=u32 1000) -> ()  [unwired: 1 out]
                                }
                                frame #2 {
                                n905 = local read "Email alert - engineer"() -> (w2434:string)
                                n906 = local read "Email alert - CC"() -> (w2433:string)
                                n907 = local read "Email alert - message"() -> (w2435:string)
                                n908 = call "email_alert.vi"("Email Alert - Message"=w2435, "Email Alert - Engineer"=w2434, "Email Alert - CC"=w2433, "Email ALert - Attachment"=w2432) -> ()  [unwired: 8 in]
                                }
                                }
                                }
                                }
                                }
                                frame #1 {
                                n909 = Wait (ms)(milliseconds to wait=u32 200) -> ()  [unwired: 1 out]
                                }
                                frame #2 {
                                # "text"
                                n910 = local read "Enable text notification"() -> (w2437:bool)
                                n911 = case shown="True" w2437 {
                                frame False {
                                }
                                frame True {
                                n912 = local read "Number of text alerts"() -> (w2441:u32)
                                n913 = Increment(x=w2441) -> (x+1=w2440:u32)
                                n914 = local write "Number of text alerts"(w2440) -> ()
                                n915 = local read "Number of email alerts"() -> (w2450:u32)
                                n916 = local read "Carrier"() -> (w2443:enum16{"T-Mobile", "AT&T", "Verizon", "Sprint"})
                                n917 = local read "Phone number"() -> (w2442:string)
                                n918 = local read "Body"() -> (w2439:string)
                                n919 = local read "Lot number"() -> (w2444:string)
                                n920 = local read "Subject"() -> (w2438:string)
                                n921 = Number To Decimal String(number=w2450) -> (decimal integer string=w2446:string)  [unwired: 1 in]
                                n922 = Concatenate Strings(w2439, ", # " ("string"), w2446, ", Lot Number: " ("string"), w2444) -> (w2451:string)
                                n923 = local write "Notifications Lot Display"(w2444) -> ()
                                n924 = call <userlib>:"Send SMS 2009.vi"("Body"=w2451, "Carrier"=w2443, "Subject"=w2438, "phone number"=w2442, "smtp server"="smtp.gmail.com", "password"="sentinelcontroller", "email username"="sentinelcontroller@gmail.com") -> ("Error Out"=w2449:errorcluster)  [unwired: 4 in]
                                n925 = Unbundle By Name(w2449) -> ("status"=w2448:bool)
                                n926 = case shown="True" w2448 {
                                frame False {
                                }
                                frame True {
                                n927 = One Button Dialog(message="Warning:\nError sending text message!\nTry changing the settings or\nswitch to email method", button name ("OK")="Dismiss") -> ()  [unwired: 1 out]
                                }
                                }
                                }
                                }
                                }
                                }
                                }
                                }
                                }
                                frame #4 {
                                n928 = Wait (ms)(milliseconds to wait=u32 100) -> ()  [unwired: 1 out]
                                }
                              }
                            }
                          }
                        }
                      }
                    }
                  }
                }
              }
              n929 = Wait (ms)(milliseconds to wait=u32 100) -> ()  [unwired: 1 out]
            }
            n930 = local read "Yield averaging"() -> (w350:u32)
            n931 = local read "UPH averaging"() -> (w349:u32)
            n932 = local read "Yield averaging"() -> (w351:u32)
            n933 = local read "UPH averaging"() -> (w352:u32)
            n934 = Initialize Array(w347, w350) -> (w348:i32[])
            n935 = Initialize Array(w346, w349) -> (w345:dbl[])
            n936 = Initialize Array(w354, w351) -> (w353:i32[])
            n937 = Initialize Array(w355, w352) -> (w356:dbl[])
            n938 = while {
              shift-right: [w1720] -> _
              shift-left: w346 -> [w1726]
              shift-right: [w1721] -> _
              shift-left: w345 -> [w1725]
              shift-right: [w1722] -> _
              shift-left: w347 -> [w1719]
              shift-right: [w1723] -> _
              shift-left: w348 -> [w1724]
              stop <- w1717 stop-if-true
              # "if there is now a lock, it is unlikely that the test time is going to be less than 100ms,\nso this is a relatively slow loop"
              n939 = local read "H2 Lock"() -> (w1716:bool)
              n940 = Wait (ms)(milliseconds to wait=u32 50) -> ()  [unwired: 1 out]
              n941 = case shown="True" w1716 {
                tunnel: w1726 -> [w1731 w1756]
                tunnel: w1725 -> [w1730 w1751]
                tunnel: w1724 -> [w1728 w1748]
                tunnel: [w1728 w1742] -> w1723
                tunnel: [w1729 w1740] -> w1722
                tunnel: [w1730 w1739] -> w1721
                tunnel: [w1731 w1738] -> w1720
                tunnel: w1719 -> [w1729 w1737]
                frame False {
                  n942 = local write "Calc H1 UPH"(u32 0 ("Sim H1 UPH")) -> ()
                }
                frame True {
                  n943 = flat-sequence {
                    tunnel: w1748 -> [w1759]
                    tunnel: w1737 -> [w1760]
                    tunnel: w1751 -> [w1761]
                    tunnel: w1756 -> [w1762]
                    tunnel: [w1762] -> w1747
                    tunnel: [w1761] -> w1746
                    tunnel: [w1760] -> w1745
                    tunnel: [w1759] -> w1744
                    tunnel: [w1775] -> w1755
                    tunnel: [w1774] -> w1752
                    tunnel: [w1773] -> w1750
                    tunnel: [w1772] -> w1749
                    tunnel: w1747 -> [w1775]
                    tunnel: w1746 -> [w1774]
                    tunnel: w1745 -> [w1773]
                    tunnel: w1744 -> [w1772]
                    tunnel: w1755 -> [w1801]
                    tunnel: [w1801] -> w1754
                    tunnel: [w1800] -> w1753
                    tunnel: w1752 -> [w1800]
                    tunnel: w1750 -> [w1790]
                    tunnel: w1749 -> [w1789]
                    tunnel: [w1788] -> w1743
                    tunnel: [w1787] -> w1741
                    tunnel: w1754 -> [w1827]
                    tunnel: w1753 -> [w1828]
                    tunnel: w1743 -> [w1846]
                    tunnel: w1741 -> [w1845]
                    tunnel: [w1846] -> w1736
                    tunnel: [w1845] -> w1735
                    tunnel: [w1824] -> w1734
                    tunnel: [w1823] -> w1733
                    tunnel: [w1861] -> w1738
                    tunnel: [w1862] -> w1739
                    tunnel: [w1863] -> w1740
                    tunnel: [w1864] -> w1742
                    tunnel: w1736 -> [w1864]
                    tunnel: w1735 -> [w1863]
                    tunnel: w1734 -> [w1862]
                    tunnel: w1733 -> [w1861]
                    frame #0 {
                      n944 = local read "H2 loop counter hid"() -> (w1757:u32)
                      n945 = Equal To 0?(x=w1757) -> (x = 0?=w1758:bool)
                      n946 = case shown="True" w1758 {
                        frame False {
                        }
                        frame True {
                          # "H2 first pass init"
                          n947 = local write "H2 Device Count"(0.0 ("H2 Device Count")) -> ()
                          n948 = local write "H2 measured  Index Time"(0.0 ("H2 Index Time")) -> ()
                          n949 = local write "H2 measured Test Time"(0.0 ("H2 Test Time")) -> ()
                          n950 = local write "H2 measured Wait Time"(0.0 ("H2 Wait Time")) -> ()
                          n951 = local read "H2 low UPH alarm (%)"() -> (w1766:dbl)
                          n952 = Divide(x=w1766, y=100.0) -> (x/y=w1765:dbl)
                          n953 = Bundle(0.0, w1765) -> (w1763:cluster{dbl, dbl})  [unwired: 1 in]
                          n954 = local write "H2 UPH"(w1763) -> ()
                        }
                      }
                    }
                    frame #1 {
                      # "H2 testing"
                      n955 = while {
                        stop <- w1779 stop-if-true
                        n956 = local read "H2 Lock"() -> (w1783:bool)
                        n957 = local read "POWER"() -> (w1778:bool)
                        n958 = local read "Run"() -> (w1776:bool)
                        n959 = Not(x=w1783) -> (.not. x?=w1777:bool)
                        n960 = Not(x=w1778) -> (.not. x?=w1781:bool)
                        n961 = Not(x=w1776) -> (.not. x?=w1780:bool)
                        n962 = Compound Arithmetic op=OR(w1777, w1781, w1780) -> (w1779:bool)
                        n963 = Wait (ms)(milliseconds to wait=u32 1) -> ()  [unwired: 1 out]
                      }
                    }
                    frame #2 {
                      n964 = local read "H2 cycle yield hid"() -> (w1784:dbl)
                      n965 = local read "H2 loop counter hid"() -> (w1785:u32)
                      n966 = local read "Yield averaging"() -> (w1786:u32)
                      n967 = local read "H2 low yield alarm"() -> (w1799:dbl)
                      n968 = local read "YieldMon"() -> (w1792:cluster{i32, i32, i32, i32})
                      n969 = local read "H2  low yield warning"() -> (w1798:dbl)
                      n970 = call "moving_avg_core.vi"("Array in"=w1789, "avg"=w1786, "accumulator in"=w1790, "i"=w1785, "data in"=w1784) -> ("Array out"=w1788:dbl[], "accumulator out"=w1787:dbl, "rolling avg out"=w1793:dbl)  [unwired: 4 in]
                      n971 = Unbundle(w1792) -> (w1791:i32)  [unwired: 3 out]
                      n972 = Less?(x=w1793, y=w1798) -> (x < y?=w1797:bool)
                      n973 = case shown="True" w1797 {
                        tunnel: w1793 -> [_ w1806]
                        tunnel: w1799 -> [_ w1805]
                        frame False {
                          n974 = local write "H2 nominal"(TRUE ("H1 nominal")) -> ()
                          n975 = local write "H2 warning"(FALSE ("H1 warning")) -> ()
                          n976 = local write "H2 alarm"(FALSE ("H1 warning")) -> ()
                        }
                        frame True {
                          n977 = Less?(x=w1806, y=w1805) -> (x < y?=w1807:bool)
                          n978 = case shown="True" w1807 {
                            frame False {
                              n979 = local write "H2 nominal"(FALSE ("H1 nominal")) -> ()
                              n980 = local write "H2 warning"(TRUE ("H1 warning")) -> ()
                              n981 = local write "H2 alarm"(FALSE ("H1 warning")) -> ()
                            }
                            frame True {
                              n982 = local read "H2 enable halt\non yield alarm"() -> (w1811:bool)
                              n983 = local write "H2 nominal"(FALSE ("H1 nominal")) -> ()
                              n984 = local write "H2 alarm"(TRUE ("H1 warning")) -> ()
                              n985 = local write "H2 warning"(FALSE ("H1 warning")) -> ()
                              n986 = case shown="True" w1811 {
                                frame False {
                                }
                                frame True {
                                n987 = local write "H2 online"(FALSE ("H1 Online")) -> ()
                                }
                              }
                            }
                          }
                        }
                      }
                      n988 = local read "H1 low yield alarm"() -> (w1796:dbl)
                      n989 = local read "H2 low yield alarm"() -> (w1795:dbl)
                      n990 = Bundle(w1791, "rolling avg out"=w1793, "H1 low yield alarm"=w1796, "H2 low yield alarm"=w1795) -> (w1794:T11)  [unwired: 1 in]
                      n991 = local write "YieldMon"(w1794) -> ()
                    }
                    frame #3 {
                      n992 = local read "H2 measured  Index Time"() -> (w1817:dbl)
                      n993 = local read "H2 measured Wait Time"() -> (w1816:dbl)
                      n994 = local read "H2 measured Test Time"() -> (w1818:dbl)
                      n995 = local read "H2 parallelism"() -> (w1830:u32)
                      n996 = local read "H2 lot yield mon"() -> (w1844:dbl)
                      n997 = local write "H2 IT (scycle)"(w1817) -> ()
                      n998 = local write "H2 TT (s/cycle)"(w1818) -> ()
                      n999 = local write "H2 WT (s/cycle)"(w1816) -> ()
                      n1000 = Compound Arithmetic op=ADD(w1817, w1818, w1816) -> (w1833:dbl)
                      n1001 = Compound Arithmetic op=ADD(w1817, w1818) -> (w1829:dbl)
                      n1002 = Multiply(x=w1830, y=3600.0 ("x")) -> (x*y=w1832:dbl)
                      n1003 = Divide(x=w1832, y=w1833) -> (x/y=w1843:dbl)
                      n1004 = Divide(x=w1844, y=w1829) -> (x/y=w1822:dbl)
                      n1005 = local write "H2 Single Handler UPH hid"(w1822) -> ()
                      n1006 = local read "H2 low UPH warning (%)"() -> (w1840:dbl)
                      n1007 = local read "H2 loop counter hid"() -> (w1826:u32)
                      n1008 = local read "Yield averaging"() -> (w1825:u32)
                      n1009 = local read "H2 low UPH alarm (%)"() -> (w1835:dbl)
                      n1010 = property on="H2 UPH" class="Knob (strict)"() -> ("Scale.Maximum"=w1841:dbl)  [unwired: 2 in, 2 out]
                      n1011 = Divide(x=w1840, y=100.0) -> (x/y=w1839:dbl)
                      n1012 = call "moving_avg_core.vi"("Array in"=w1828, "avg"=w1825, "accumulator in"=w1827, "i"=w1826, "data in"=w1843) -> ("Array out"=w1824:dbl[], "accumulator out"=w1823:dbl, "rolling avg out"=w1842:dbl)  [unwired: 4 in]
                      n1013 = Multiply(x=w1841, y=w1839) -> (x*y=w1821:dbl)
                      n1014 = Divide(x=w1835, y=100.0) -> (x/y=w1837:dbl)
                      n1015 = local write "H2 UPH warning limit hid"(w1821) -> ()
                      n1016 = Less?(x=w1842, y=w1821) -> (x < y?=w1834:bool)
                      n1017 = Multiply(x=w1841, y=w1837) -> (x*y=w1820:dbl)
                      n1018 = case shown="True" w1834 {
                        tunnel: w1842 -> [_ w1851]
                        tunnel: w1820 -> [_ w1850]
                        frame False {
                          n1019 = local write "H2 nominal 2"(TRUE ("H1 nominal")) -> ()
                          n1020 = local write "H2 warning 2"(FALSE ("H1 warning")) -> ()
                          n1021 = local write "H2 alarm 2"(FALSE ("H1 warning")) -> ()
                        }
                        frame True {
                          n1022 = Less?(x=w1851, y=w1850) -> (x < y?=w1852:bool)
                          n1023 = case shown="True" w1852 {
                            frame False {
                              n1024 = local write "H2 nominal 2"(FALSE ("H1 nominal")) -> ()
                              n1025 = local write "H2 warning 2"(TRUE ("H1 warning")) -> ()
                              n1026 = local write "H2 alarm 2"(FALSE ("H1 warning")) -> ()
                            }
                            frame True {
                              n1027 = local read "H2 enable halt\non UPH alarm"() -> (w1856:bool)
                              n1028 = local write "H2 alarm 2"(TRUE ("H1 warning")) -> ()
                              n1029 = local write "H2 warning 2"(FALSE ("H1 warning")) -> ()
                              n1030 = local write "H2 nominal 2"(FALSE ("H1 nominal")) -> ()
                              n1031 = case shown="True" w1856 {
                                frame False {
                                }
                                frame True {
                                n1032 = local write "H2 online"(FALSE ("H1 Online")) -> ()
                                }
                              }
                            }
                          }
                        }
                      }
                      n1033 = local write "H2 UPH alarm limit hid"(w1820) -> ()
                      n1034 = Bundle("rolling avg out"=w1842, w1820) -> (w1819:cluster{"rolling avg out":dbl, dbl})  [unwired: 1 in]
                      n1035 = local write "H2 UPH"(w1819) -> ()
                    }
                    frame #4 {
                      n1036 = while {
                        stop <- w1866 continue-if-true
                        n1037 = local read "H2 Lock"() -> (w1866:bool)
                        n1038 = Wait (ms)(milliseconds to wait=u32 10) -> ()  [unwired: 1 out]
                      }
                    }
                  }
                }
              }
              n1039 = local read "POWER"() -> (w1718:bool)
              n1040 = Not(x=w1718) -> (.not. x?=w1717:bool)
            }
            n1041 = while {
              shift-right: [w2597] -> _
              shift-left: w355 -> [w2600]
              shift-right: [w2598] -> _
              shift-left: w356 -> [w2599]
              shift-right: [w2593] -> _
              shift-left: w354 -> [w2596]
              shift-right: [w2594] -> _
              shift-left: w353 -> [w2595]
              stop <- w2592 stop-if-true
              # "if there is now a lock, it is unlikely that the test time is going to be less than 100ms,\nso this is a relatively slow loop"
              n1042 = local read "H1 Lock"() -> (w2591:bool)
              n1043 = case shown="True" w2591 {
                tunnel: w2600 -> [w2606 w2631]
                tunnel: w2599 -> [w2605 w2626]
                tunnel: [w2605 w2625] -> w2598
                tunnel: [w2606 w2624] -> w2597
                tunnel: w2596 -> [w2604 w2622]
                tunnel: w2595 -> [w2603 w2620]
                tunnel: [w2603 w2618] -> w2594
                tunnel: [w2604 w2616] -> w2593
                frame False {
                  n1044 = local write "Calc H1 UPH"(u32 0 ("Sim H1 UPH")) -> ()
                }
                frame True {
                  n1045 = flat-sequence {
                    tunnel: w2620 -> [w2634]
                    tunnel: w2622 -> [w2635]
                    tunnel: w2626 -> [w2636]
                    tunnel: w2631 -> [w2637]
                    tunnel: [w2637] -> w2615
                    tunnel: [w2636] -> w2614
                    tunnel: [w2635] -> w2613
                    tunnel: [w2634] -> w2612
                    tunnel: [w2650] -> w2630
                    tunnel: [w2649] -> w2627
                    tunnel: [w2648] -> w2623
                    tunnel: [w2647] -> w2621
                    tunnel: w2615 -> [w2650]
                    tunnel: w2614 -> [w2649]
                    tunnel: w2613 -> [w2648]
                    tunnel: w2612 -> [w2647]
                    tunnel: w2630 -> [w2665]
                    tunnel: [w2665] -> w2629
                    tunnel: [w2664] -> w2628
                    tunnel: w2627 -> [w2664]
                    tunnel: w2623 -> [w2663]
                    tunnel: w2621 -> [w2662]
                    tunnel: [w2661] -> w2619
                    tunnel: [w2660] -> w2617
                    tunnel: w2629 -> [w2703]
                    tunnel: w2628 -> [w2702]
                    tunnel: w2619 -> [w2699]
                    tunnel: w2617 -> [w2698]
                    tunnel: [w2701] -> w2611
                    tunnel: [w2700] -> w2610
                    tunnel: [w2699] -> w2609
                    tunnel: [w2698] -> w2608
                    tunnel: [w2738] -> w2616
                    tunnel: [w2739] -> w2618
                    tunnel: [w2740] -> w2624
                    tunnel: [w2741] -> w2625
                    tunnel: w2611 -> [w2741]
                    tunnel: w2610 -> [w2740]
                    tunnel: w2609 -> [w2739]
                    tunnel: w2608 -> [w2738]
                    frame #0 {
                      n1046 = local read "H1 loop counter hid"() -> (w2633:u32)
                      n1047 = Equal To 0?(x=w2633) -> (x = 0?=w2632:bool)
                      n1048 = case shown="True" w2632 {
                        frame False {
                        }
                        frame True {
                          n1049 = local read "H1 low UPH alarm (%)"() -> (w2642:dbl)
                          n1050 = local write "H1 measured Index Time"(0.0 ("H1 Index Time")) -> ()
                          n1051 = local write "H1 measured Wait Time"(0.0 ("H1 Wait Time")) -> ()
                          n1052 = local write "H1 Device Count"(0.0 ("H1 Device Count")) -> ()
                          n1053 = local write "H1 measured Test Time"(0.0 ("H1 Test Time")) -> ()
                          n1054 = Divide(x=w2642, y=100.0) -> (x/y=w2640:dbl)
                          n1055 = Bundle("y"=0.0, w2640) -> (w2638:cluster{"y":dbl, dbl})  [unwired: 1 in]
                          n1056 = local write "H1 UPH"(w2638) -> ()
                        }
                      }
                    }
                    frame #1 {
                      # "H1 testing"
                      n1057 = while {
                        stop <- w2654 stop-if-true
                        n1058 = local read "H1 Lock"() -> (w2658:bool)
                        n1059 = local read "POWER"() -> (w2652:bool)
                        n1060 = local read "Run"() -> (w2651:bool)
                        n1061 = Wait (ms)(milliseconds to wait=u32 1) -> ()  [unwired: 1 out]
                        n1062 = Not(x=w2658) -> (.not. x?=w2653:bool)
                        n1063 = Not(x=w2652) -> (.not. x?=w2656:bool)
                        n1064 = Not(x=w2651) -> (.not. x?=w2655:bool)
                        n1065 = Compound Arithmetic op=OR(w2653, w2656, w2655) -> (w2654:bool)
                      }
                    }
                    frame #2 {
                      n1066 = local read "H1 cycle yield hid"() -> (w2668:dbl)
                      n1067 = local read "H1 loop counter hid"() -> (w2667:u32)
                      n1068 = local read "Yield averaging"() -> (w2666:u32)
                      n1069 = local read "H1 low yield warning"() -> (w2676:dbl)
                      n1070 = local read "H1 low yield alarm"() -> (w2674:dbl)
                      n1071 = call "moving_avg_core.vi"("Array in"=w2662, "avg"=w2666, "accumulator in"=w2663, "i"=w2667, "data in"=w2668) -> ("Array out"=w2661:dbl[], "accumulator out"=w2660:dbl, "rolling avg out"=w2671:dbl)  [unwired: 4 in]
                      n1072 = Less?(x=w2671, y=w2676) -> (x < y?=w2675:bool)
                      n1073 = case shown="True" w2675 {
                        tunnel: w2671 -> [_ w2682]
                        tunnel: w2674 -> [_ w2681]
                        frame False {
                          n1074 = local write "H1 alarm"(FALSE ("H1 warning")) -> ()
                          n1075 = local write "H1 warning"(FALSE ("H1 warning")) -> ()
                          n1076 = local write "H1 nominal"(TRUE ("H1 nominal")) -> ()
                        }
                        frame True {
                          n1077 = Less?(x=w2682, y=w2681) -> (x < y?=w2680:bool)
                          n1078 = case shown="True" w2680 {
                            frame False {
                              n1079 = local write "H1 alarm"(FALSE ("H1 warning")) -> ()
                              n1080 = local write "H1 warning"(TRUE ("H1 warning")) -> ()
                              n1081 = local write "H1 nominal"(FALSE ("H1 nominal")) -> ()
                            }
                            frame True {
                              n1082 = local read "H1 enable halt\non yield alarm"() -> (w2686:bool)
                              n1083 = local write "H1 nominal"(FALSE ("H1 nominal")) -> ()
                              n1084 = local write "H1 warning"(FALSE ("H1 warning")) -> ()
                              n1085 = local write "H1 alarm"(TRUE ("H1 warning")) -> ()
                              n1086 = case shown="True" w2686 {
                                frame False {
                                }
                                frame True {
                                n1087 = local write "H1 online"(FALSE ("H1 Online")) -> ()
                                }
                              }
                            }
                          }
                        }
                      }
                      n1088 = local read "YieldMon"() -> (w2670:cluster{i32, i32, i32, i32})
                      n1089 = local read "H1 low yield alarm"() -> (w2673:dbl)
                      n1090 = local read "H2 low yield alarm"() -> (w2672:dbl)
                      n1091 = Unbundle(w2670) -> (w2659:i32)  [unwired: 3 out]
                      n1092 = Bundle("rolling avg out"=w2671, w2659, "H1 low yield alarm"=w2673, "H2 low yield alarm"=w2672) -> (w2669:T12)  [unwired: 1 in]
                      n1093 = local write "YieldMon"(w2669) -> ()
                    }
                    frame #3 {
                      n1094 = local read "H1 measured Index Time"() -> (w2693:dbl)
                      n1095 = local read "H1 measured Wait Time"() -> (w2691:dbl)
                      n1096 = local read "H1 measured Test Time"() -> (w2692:dbl)
                      n1097 = local read "H1 parallelism"() -> (w2710:u32)
                      n1098 = local read "H1 loop counter hid"() -> (w2705:u32)
                      n1099 = local read "UPH averaging"() -> (w2704:u32)
                      n1100 = local read "H1 low UPH warning (%)"() -> (w2714:dbl)
                      n1101 = local write "H1 IT (s/cycle)"(w2693) -> ()
                      n1102 = local write "H1 TT (s/cycle)"(w2692) -> ()
                      n1103 = local write "H1 WT (s/cycle)"(w2691) -> ()
                      n1104 = Compound Arithmetic op=ADD(w2693, w2692, w2691) -> (w2706:dbl)
                      n1105 = Compound Arithmetic op=ADD(w2693, w2692) -> (w2713:dbl)
                      n1106 = Multiply(x=w2710, y=u32 3600 ("x")) -> (x*y=w2712:u32)
                      n1107 = Divide(x=w2712, y=w2713) -> (x/y=w2696:dbl)
                      n1108 = local read "H1 low UPH alarm (%)"() -> (w2719:dbl)
                      n1109 = local write "H1 Single Handler UPH hid"(w2696) -> ()
                      n1110 = property on="H1 UPH" class="Knob (strict)"() -> ("Scale.Maximum"=w2721:dbl)  [unwired: 2 in, 2 out]
                      n1111 = Divide(x=w2714, y=100.0) -> (x/y=w2715:dbl)
                      n1112 = Multiply(x=w2721, y=w2715) -> (x*y=w2694:dbl)
                      n1113 = Divide(x=w2719, y=100.0) -> (x/y=w2717:dbl)
                      n1114 = local write "H1 UPH warning limit hid"(w2694) -> ()
                      n1115 = Multiply(x=w2721, y=w2717) -> (x*y=w2695:dbl)
                      n1116 = local write "H1 UPH alarm limit hid"(w2695) -> ()
                      n1117 = local read "H1 parallelism"() -> (w2709:u32)
                      n1118 = Multiply(x=w2709, y=u32 3600 ("x")) -> (x*y=w2707:u32)
                      n1119 = Divide(x=w2707, y=w2706) -> (x/y=w2723:dbl)
                      n1120 = call "moving_avg_core.vi"("Array in"=w2702, "avg"=w2704, "accumulator in"=w2703, "i"=w2705, "data in"=w2723) -> ("Array out"=w2701:dbl[], "accumulator out"=w2700:dbl, "rolling avg out"=w2722:dbl)  [unwired: 4 in]
                      n1121 = Less?(x=w2722, y=w2694) -> (x < y?=w2720:bool)
                      n1122 = case shown="True" w2720 {
                        tunnel: w2722 -> [_ w2728]
                        tunnel: w2695 -> [_ w2727]
                        frame False {
                          n1123 = local write "H1 alarm 2"(FALSE ("H1 warning")) -> ()
                          n1124 = local write "H1 nominal 2"(TRUE ("H1 nominal")) -> ()
                          n1125 = local write "H1 warning 2"(FALSE ("H1 warning")) -> ()
                        }
                        frame True {
                          n1126 = Less?(x=w2728, y=w2727) -> (x < y?=w2729:bool)
                          n1127 = case shown="True" w2729 {
                            frame False {
                              n1128 = local write "H1 nominal 2"(FALSE ("H1 nominal")) -> ()
                              n1129 = local write "H1 warning 2"(TRUE ("H1 warning")) -> ()
                              n1130 = local write "H1 alarm 2"(FALSE ("H1 warning")) -> ()
                            }
                            frame True {
                              n1131 = local read "H1 enable halt\non UPH alarm"() -> (w2733:bool)
                              n1132 = local write "H1 warning 2"(FALSE ("H1 warning")) -> ()
                              n1133 = local write "H1 alarm 2"(TRUE ("H1 warning")) -> ()
                              n1134 = local write "H1 nominal 2"(FALSE ("H1 nominal")) -> ()
                              n1135 = case shown="True" w2733 {
                                frame False {
                                }
                                frame True {
                                n1136 = local write "H1 online"(FALSE ("H1 Online")) -> ()
                                }
                              }
                            }
                          }
                        }
                      }
                      n1137 = Bundle("rolling avg out"=w2722, w2695) -> (w2697:cluster{"rolling avg out":dbl, dbl})  [unwired: 1 in]
                      n1138 = local write "H1 UPH"(w2697) -> ()
                    }
                    frame #4 {
                      n1139 = while {
                        stop <- w2743 continue-if-true
                        n1140 = local read "H1 Lock"() -> (w2743:bool)
                        n1141 = Wait (ms)(milliseconds to wait=u32 10) -> ()  [unwired: 1 out]
                      }
                    }
                  }
                }
              }
              n1142 = Wait (ms)(milliseconds to wait=u32 50) -> ()  [unwired: 1 out]
              n1143 = local read "POWER"() -> (w2602:bool)
              n1144 = Not(x=w2602) -> (.not. x?=w2592:bool)
            }
            n1145 = while {
              stop <- w582 continue-if-true
              n1146 = while {
                stop <- w584 stop-if-true
                n1147 = event shown="[1] \"H1 online\": Value Change" {
                  selector: _ -> [_ _]
                  dyn-events: _ -> [_ _]
                  timeout: -1 -> [_ _]
                  tunnel: [_ TRUE] -> w584
                  event Timeout {
                    n1148 = event-data() -> ()  [unwired: 1 in, 2 out]
                  }
                  event "H1 online": Value Change {
                    n1149 = event-data() -> ()  [unwired: 1 in, 5 out]
                    n1150 = local read "Enable data logging of all events"() -> (w585:bool)
                    n1151 = case shown="True" w585 {
                      frame False {
                      }
                      frame True {
                        w589 = "\r\n"
                        n1152 = Get Date/Time String(want seconds? (F)=TRUE) -> (date string=w594:string, time string=w593:string)  [unwired: 2 in]
                        n1153 = local read "H1 online"() -> (w591:bool)
                        n1154 = case shown="False" w591 {
                          tunnel: ["H1 Off-Line" "H1 On-Line"] -> w590
                          frame False {
                          }
                          frame True {
                          }
                        }
                        n1155 = local read "Data log path and filename"() -> (w588:path)
                        n1156 = Concatenate Strings(w594, "   " ("string"), w593, w589, "Change in H1 Status: ", w590, w589, w589) -> (w596:string)
                        n1157 = call "SentinelDatalog.vi"("operation (0:open)"=T9."open", "String"=w596, "data log path"=w588) -> ()  [unwired: 8 in, 1 out]
                      }
                    }
                  }
                }
              }
              n1158 = local read "POWER"() -> (w582:bool)
            }
            n1159 = while {
              stop <- w564 continue-if-true
              n1160 = while {
                stop <- w566 stop-if-true
                n1161 = event shown="[1] \"H2 online\": Value Change" {
                  selector: _ -> [_ _]
                  dyn-events: _ -> [_ _]
                  timeout: -1 -> [_ _]
                  tunnel: [_ TRUE] -> w566
                  event Timeout {
                    n1162 = event-data() -> ()  [unwired: 1 in, 2 out]
                  }
                  event "H2 online": Value Change {
                    n1163 = event-data() -> ()  [unwired: 1 in, 5 out]
                    n1164 = local read "Enable data logging of all events"() -> (w567:bool)
                    n1165 = case shown="True" w567 {
                      frame False {
                      }
                      frame True {
                        w571 = "\r\n"
                        n1166 = local read "H2 online"() -> (w573:bool)
                        n1167 = case shown="False" w573 {
                          tunnel: ["H2 Off-Line" "H2 On-Line"] -> w572
                          frame False {
                          }
                          frame True {
                          }
                        }
                        n1168 = local read "Data log path and filename"() -> (w570:path)
                        n1169 = Get Date/Time String(want seconds? (F)=TRUE) -> (date string=w576:string, time string=w575:string)  [unwired: 2 in]
                        n1170 = Concatenate Strings(w576, "   " ("string"), w575, w571, "Change in H2 Status: ", w572, w571, w571) -> (w578:string)
                        n1171 = call "SentinelDatalog.vi"("operation (0:open)"=T9."open", "String"=w578, "data log path"=w570) -> ()  [unwired: 8 in, 1 out]
                      }
                    }
                  }
                }
              }
              n1172 = local read "POWER"() -> (w564:bool)
            }
            n1173 = while {
              stop <- w712 continue-if-true
              n1174 = local read "Tester online"() -> (w713:bool)
              n1175 = case shown="True" w713 {
                frame False {
                }
                frame True {
                  n1176 = flat-sequence {
                    frame #0 {
                      n1177 = local write "Exit SC handler StMach hid"(FALSE ("Exit tester state machine hid")) -> ()
                      n1178 = local write "SC handler states hid"(SC_handler_states."initializing bus" ("SC virtual handler states")) -> ()
                    }
                    frame #1 {
                      n1179 = flat-sequence {
                        tunnel: [w720] -> w717
                        tunnel: [w719] -> w718
                        frame #0 {
                          w719 = 0.0
                          # "These are consumed in the \"responding to sites\"\nstate when at least one handler has sites ready.  \nIt is executed only after one cycle. At that point,\nthere is at least one test period and one wait period\nto make a utilization calculation."
                          n1180 = local read "Utilization averaging"() -> (w721:i32)
                          n1181 = Initialize Array(w719, w721) -> (w720:dbl[])
                        }
                      }
                      n1182 = while {
                        shift-right: [w728] -> _
                        shift-left: w718 -> [w723]
                        shift-right: [w724] -> _
                        shift-left: w717 -> [w722]
                        stop <- w725 stop-if-true
                        n1183 = flat-sequence {
                          tunnel: [w734] -> w727
                          tunnel: [w733] -> w726
                          tunnel: w723 -> [w732]
                          tunnel: w722 -> [w731]
                          tunnel: [w1509] -> w724
                          tunnel: [w1510] -> w728
                          tunnel: w727 -> [w1510]
                          tunnel: w726 -> [w1509]
                          frame #0 {
                            n1184 = local read "SC handler states hid"() -> (w730:T6)
                            n1185 = case shown="\"waiting on serial poll\"" w730 {
                              tunnel: w732 -> [w735 w758 w811 w840 w908 w924 w959 w994 w1034 w1068 w1144 w1246 w1346 w1374 w1490 w1501]
                              tunnel: [w736 w759 w812 w841 w909 w925 w958 w993 w1031 w1067 w1143 w1245 w1345 w1373 w1489 w1500] -> w733
                              tunnel: w731 -> [w736 w759 w812 w841 w909 w925 w958 w993 w1033 w1067 w1143 w1245 w1345 w1373 w1489 w1500]
                              tunnel: [w735 w758 w811 w840 w908 w924 w959 w994 w1032 w1068 w1144 w1246 w1346 w1374 w1490 w1501] -> w734
                              frame "initializing bus", Default {
                                n1186 = flat-sequence {
                                frame #0 {
                                n1187 = local write "VISA bus 0 close error"(FALSE ("VISA bus 0 close error")) -> ()
                                }
                                frame #1 {
                                w745 = T13 1073684500 items=["Service Request"=1073684491, "Trigger"=3221168138, "Clear"=1073684493, "VXI Signal"=1073684512, "VXI/VME Interrupt"=3221168161, "VXI/VME Sysfail"=1073684509, "VXI/VME Sysreset"=1073684510, "GPIB CIC"=1073684498, "GPIB Talk"=1073684499, "GPIB Listen"=1073684500, "PXI Interrupt"=1073684514, "Serial Break"=1073684515, "Serial TermChar"=1073684516, "Serial CTS"=1073684521, "Serial DSR"=1073684522, "Serial DCD"=1073684524, "Serial RI"=1073684526, "Serial Character"=1073684533, "USB Interrupt"=1073684535, "All Enabled"=1073709055] ("Event Type")
                                n1188 = local read "SentCtrl listens to tester at"() -> (w742:refnum<visa-resource-name>)
                                n1189 = local read "GPIB wait timeout hid"() -> (w740:u32)
                                n1190 = VISA Open(VISA resource name=w742) -> (VISA resource name=w747:refnum<visa-resource-name>, error out=w746:errorcluster)  [unwired: 1 in, 3 out]
                                n1191 = Unbundle By Name(w746) -> ()  [unwired: 1 out]
                                n1192 = property class="GPIB BoardInterface"(reference=w747, error in=w746, "General Settings:Timeout Value"=w740) -> (reference out=w744:refnum<visa-resource-name>, error out=w743:errorcluster)
                                n1193 = VISA Enable Event(8:w743, 10:w745, 11:w744) -> (0:w739:errorcluster, 3:→"VISA bus 0 resource name out hid":refnum<visa-resource-name>)  [unwired: 1 out]
                                "VISA bus 0 error out hid" <- w739
                                n1194 = Unbundle By Name(w739) -> ("status"=w738:bool)
                                n1195 = local write "VISA bus 0 open error"(w738) -> ()
                                }
                                frame #2 {
                                n1196 = Concatenate Strings("Bus 0 initializing " ("string"), "\r\n") -> (w749:string)
                                n1197 = local write "GPIB Bus 0 traffic"(w749) -> ()
                                }
                                frame #3 {
                                n1198 = local write "Exit SC handler StMach hid"(FALSE ("Exit tester state machine hid")) -> ()
                                n1199 = local write "Last locked handler hid"(enum16{"H1", "H2"}."H1" ("Last locked handler hid")) -> ()
                                n1200 = local write "H1 Lock"(FALSE ("H1 Lock")) -> ()
                                n1201 = local write "H2 Lock"(FALSE ("H1 Lock")) -> ()
                                }
                                frame #4 {
                                n1202 = local read "Tester Handler Config"() -> (w755:T2)
                                n1203 = case shown="\"Seiko-Epson NS6040\"" w755 {
                                frame "Multitest", Default {
                                n1204 = local write "SC handler states hid"(SC_handler_states."waiting on event" ("SC Test Interface States")) -> ()
                                }
                                frame "Seiko-Epson NS6040" {
                                n1205 = local write "SC handler states hid"(SC_handler_states."waiting on serial poll" ("SC Test Interface States")) -> ()
                                }
                                }
                                }
                                }
                              }
                              frame "waiting on serial poll" {
                                n1206 = flat-sequence {
                                frame #0 {
                                n1207 = property class="GPIB BoardInterface"(reference=refnum<visa-resource-name> "GPIB0::INTFC", "Device STB"=u8 0 ("Message Based Settings:Device Status Byte")) -> ()  [unwired: 1 in, 2 out]
                                n1208 = local write "GPIB Bus 0 traffic"("Bus 0 waiting on SPOLL" ("string")) -> ()
                                }
                                frame #1 {
                                n1209 = while {
                                stop <- w764 stop-if-true
                                n1210 = local read "H2 Ready with sites hid"() -> (w765:bool)
                                n1211 = local read "H1 Ready with sites hid"() -> (w766:bool)
                                n1212 = Wait (ms)(milliseconds to wait=u32 20) -> ()  [unwired: 1 out]
                                n1213 = Or(x=w765, y=w766) -> (x .or. y?=w764:bool)
                                }
                                }
                                frame #2 {
                                n1214 = property class="GPIB BoardInterface"(reference=refnum<visa-resource-name> "GPIB0::INTFC", "Device STB"=u8 65 ("Message Based Settings:Device Status Byte")) -> ()  [unwired: 1 in, 2 out]
                                }
                                frame #3 {
                                w772 = T13 1073684500 items=["Service Request"=1073684491, "Trigger"=3221168138, "Clear"=1073684493, "VXI Signal"=1073684512, "VXI/VME Interrupt"=3221168161, "VXI/VME Sysfail"=1073684509, "VXI/VME Sysreset"=1073684510, "GPIB CIC"=1073684498, "GPIB Talk"=1073684499, "GPIB Listen"=1073684500, "PXI Interrupt"=1073684514, "Serial Break"=1073684515, "Serial TermChar"=1073684516, "Serial CTS"=1073684521, "Serial DSR"=1073684522, "Serial DCD"=1073684524, "Serial RI"=1073684526, "Serial Character"=1073684533, "USB Interrupt"=1073684535, "All Enabled"=1073709055] ("Event Type")
                                n1215 = local read "VISA bus 0 resource name out hid"() -> (w774:refnum<visa-resource-name>)
                                n1216 = local read "GPIB wait timeout hid"() -> (w770:u32)
                                n1217 = local read "VISA bus 0 error out hid"() -> (w773:errorcluster)
                                n1218 = VISA Wait on Event(7:w770, 8:w773, 10:w772, 11:w774) -> (0:w771:errorcluster)  [unwired: 1 in, 3 out]
                                n1219 = Unbundle By Name(w771) -> ("status"=w769:bool)
                                n1220 = local write "GPIB bus 0 read error"(w769) -> ()
                                n1221 = case shown="False" w769 {
                                frame False {
                                n1222 = flat-sequence {
                                frame #0 {
                                n1223 = while {
                                stop <- w780 stop-if-true
                                n1224 = property class="GPIB BoardInterface"(reference=refnum<visa-resource-name> "GPIB0::INTFC") -> ("ATN State"=w781:i16)  [unwired: 1 in, 2 out]
                                n1225 = local read "GPIB Bus 0 traffic"() -> (w778:string)
                                n1226 = Equal To 0?(x=w781) -> (x = 0?=w780:bool)
                                n1227 = Concatenate Strings(w778, "\r\n", "Bus 0 wait for ATT to go low" ("string")) -> (w775:string)
                                n1228 = local write "GPIB Bus 0 traffic"(w775) -> ()
                                n1229 = Wait (ms)(milliseconds to wait=u32 5) -> ()  [unwired: 1 out]
                                }
                                }
                                frame #1 {
                                n1230 = local read "Last locked handler hid"() -> (w783:enum16{"H1", "H2"})
                                n1231 = case shown="\"H1\", Default" w783 {
                                frame "H1", Default {
                                n1232 = local read "H2 Ready with sites hid"() -> (w784:bool)
                                n1233 = case shown="True" w784 {
                                frame False {
                                n1234 = local read "H1 Ready with sites hid"() -> (w785:bool)
                                n1235 = case shown="False" w785 {
                                frame False {
                                }
                                frame True {
                                n1236 = local write "H1 Lock"(TRUE ("H1 Lock")) -> ()
                                n1237 = local read "H1 loop counter hid"() -> (w789:u32)
                                n1238 = local write "Last locked handler hid"(enum16{"H1", "H2"}."H1" ("Last locked handler hid")) -> ()
                                n1239 = Increment(x=w789) -> (x+1=w788:u32)
                                n1240 = local write "H1 loop counter hid"(w788) -> ()
                                }
                                }
                                }
                                frame True {
                                n1241 = local read "H2 loop counter hid"() -> (w792:u32)
                                n1242 = local write "H2 Lock"(TRUE ("H2 Lock")) -> ()
                                n1243 = local write "Last locked handler hid"(enum16{"H1", "H2"}."H2" ("Last locked handler hid")) -> ()
                                n1244 = Increment(x=w792) -> (x+1=w793:u32)
                                n1245 = local write "H2 loop counter hid"(w793) -> ()
                                }
                                }
                                }
                                frame "H2" {
                                n1246 = local read "H1 Ready with sites hid"() -> (w794:bool)
                                n1247 = case shown="True" w794 {
                                frame False {
                                n1248 = local read "H2 Ready with sites hid"() -> (w795:bool)
                                n1249 = case shown="False" w795 {
                                frame False {
                                }
                                frame True {
                                n1250 = local write "H2 Lock"(TRUE ("H2 Lock")) -> ()
                                n1251 = local read "H2 loop counter hid"() -> (w798:u32)
                                n1252 = local write "Last locked handler hid"(enum16{"H1", "H2"}."H2" ("Last locked handler hid")) -> ()
                                n1253 = Increment(x=w798) -> (x+1=w799:u32)
                                n1254 = local write "H2 loop counter hid"(w799) -> ()
                                }
                                }
                                }
                                frame True {
                                n1255 = local read "H1 loop counter hid"() -> (w804:u32)
                                n1256 = local write "H1 Lock"(TRUE ("H1 Lock")) -> ()
                                n1257 = local write "Last locked handler hid"(enum16{"H1", "H2"}."H1" ("Last locked handler hid")) -> ()
                                n1258 = Increment(x=w804) -> (x+1=w803:u32)
                                n1259 = local write "SC handler states hid"(SC_handler_states."waiting on event" ("SC Test Interface States")) -> ()
                                n1260 = local write "H1 loop counter hid"(w803) -> ()
                                }
                                }
                                }
                                }
                                }
                                frame #2 {
                                n1261 = local write "SC handler states hid"(SC_handler_states."waiting on event" ("SC Test Interface States")) -> ()
                                }
                                }
                                }
                                frame True {
                                n1262 = flat-sequence {
                                frame #0 {
                                n1263 = local read "VISA bus 0 resource name out hid"() -> (w807:refnum<visa-resource-name>)
                                n1264 = local read "VISA bus 0 error out hid"() -> (w808:errorcluster)
                                n1265 = VISA Close(VISA resource name=w807, error in (no error)=w808) -> (error out=w806:errorcluster)
                                n1266 = Unbundle By Name(w806) -> ("status"=w809:bool)
                                n1267 = local write "VISA bus 0 close error"(w809) -> ()
                                }
                                frame #1 {
                                n1268 = local write "SC handler states hid"(SC_handler_states."initializing bus" ("SC Test Interface States")) -> ()
                                }
                                }
                                }
                                }
                                }
                                }
                              }
                              frame "waiting on event" {
                                n1269 = flat-sequence {
                                frame #0 {
                                n1270 = local read "GPIB Bus 0 traffic"() -> (w813:string)
                                n1271 = Concatenate Strings(w813, "\r\n", "Bus 0 waiting on event" ("string")) -> (w816:string)
                                n1272 = local write "GPIB Bus 0 traffic"(w816) -> ()
                                }
                                frame #1 {
                                n1273 = local read "VISA bus 0 resource name out hid"() -> (w826:refnum<visa-resource-name>)
                                n1274 = local read "VISA bus 0 error out hid"() -> (w825:errorcluster)
                                n1275 = local read "GPIB wait timeout hid"() -> (w824:u32)
                                n1276 = VISA Wait on Event(7:w824, 8:w825, 11:w826) -> (0:w817:errorcluster, 3:w818:refnum<visa-resource-name>)  [unwired: 2 in, 2 out]
                                n1277 = local write "VISA bus 0 resource name out hid"(w818) -> ()
                                n1278 = local write "VISA bus 0 error out hid"(w817) -> ()
                                n1279 = Unbundle By Name(w817) -> ("status"=w821:bool)
                                n1280 = Unbundle By Name(w817) -> ("code"=w823:i32)
                                n1281 = Equal?(x=w823, y=-1073807339) -> (x = y?=w820:bool)
                                n1282 = Or(x=w821, y=w820) -> (x .or. y?=w819:bool)
                                n1283 = case shown="False" w819 {
                                tunnel: w818 -> [_ w829]
                                tunnel: w817 -> [_ w828]
                                frame False {
                                n1284 = local write "SC handler states hid"(SC_handler_states."reading" ("SC Test Interface States")) -> ()
                                }
                                frame True {
                                n1285 = flat-sequence {
                                tunnel: w829 -> [w833]
                                tunnel: w828 -> [w832]
                                frame #0 {
                                n1286 = VISA Close(VISA resource name=w833, error in (no error)=w832) -> (error out=w831:errorcluster)
                                n1287 = Unbundle By Name(w831) -> ("status"=w830:bool)
                                n1288 = local write "VISA bus 0 close error"(w830) -> ()
                                }
                                frame #1 {
                                n1289 = Concatenate Strings("GPIB bus 0 error or time out waiting on event,\nclosing Bus 0 and re-initializing." ("string"), "\r\n") -> (w836:string)
                                n1290 = local write "GPIB Bus 0 traffic"(w836) -> ()
                                }
                                frame #2 {
                                n1291 = local write "SC handler states hid"(SC_handler_states."initializing bus" ("SC Test Interface States")) -> ()
                                }
                                }
                                }
                                }
                                }
                                }
                              }
                              frame "reading" {
                                n1292 = flat-sequence {
                                tunnel: [w842] -> w839
                                tunnel: [w845] -> w838
                                tunnel: w839 -> [w857]
                                tunnel: w838 -> [w856]
                                frame #0 {
                                n1293 = local read "VISA bus 0 resource name out hid"() -> (w852:refnum<visa-resource-name>)
                                n1294 = local read "VISA bus 0 error out hid"() -> (w853:errorcluster)
                                n1295 = VISA Read(VISA resource name=w852, byte count=128, error in (no error)=w853) -> (VISA resource name out=w851:refnum<visa-resource-name>, read buffer=w847:string, return count=w846:u32, error out=w843:errorcluster)
                                n1296 = local write "VISA bus 0 resource name out hid"(w851) -> ()
                                n1297 = local write "Message from tester hid"(w847) -> ()
                                n1298 = Unbundle By Name(w843) -> ("status"=w844:bool)
                                n1299 = call <vilib>:"Trim Whitespace.vi"("string"=w847) -> ("trimmed string"=w842:string)  [unwired: 1 in]
                                n1300 = Greater Than 0?(x=w846) -> (x > 0?=w845:bool)
                                n1301 = local write "GPIB bus 0 read error"(w844) -> ()
                                n1302 = local read "GPIB Bus 0 traffic"() -> (w850:string)
                                n1303 = Concatenate Strings(w850, "\r\n", "Bus 0 read: " ("string"), w842) -> (w848:string)
                                n1304 = local write "GPIB Bus 0 traffic"(w848) -> ()
                                }
                                frame #1 {
                                n1305 = case shown="True" w856 {
                                tunnel: w857 -> [_ w860]
                                frame False {
                                n1306 = local write "SC handler states hid"(SC_handler_states."waiting on event" ("SC Test Interface States")) -> ()
                                n1307 = Wait (ms)(milliseconds to wait=u32 1) -> ()  [unwired: 1 out]
                                }
                                frame True {
                                n1308 = flat-sequence {
                                tunnel: w860 -> [w861]
                                frame #0 {
                                n1309 = Match Pattern(string=w861, regular expression="?") -> (offset past match=w864:i32)  [unwired: 1 in, 3 out]
                                n1310 = Greater Or Equal To 0?(x=w864) -> (x >= 0?=w862:bool)
                                n1311 = case shown="False" w862 {
                                tunnel: w861 -> [w868 w883]
                                frame False {
                                n1312 = Match Pattern(string=w868, regular expression=":" ("true string")) -> (offset past match=w865:i32)  [unwired: 1 in, 3 out]
                                n1313 = Greater Or Equal To 0?(x=w865) -> (x >= 0?=w866:bool)
                                n1314 = case shown="False" w866 {
                                tunnel: w868 -> [w871 w878]
                                frame False {
                                n1315 = call <vilib>:"Space Constant.vi"() -> ("String"=w872:string)
                                n1316 = Match Pattern(string=w871, regular expression=w872) -> (offset past match=w870:i32)  [unwired: 1 in, 3 out]
                                n1317 = Greater Or Equal To 0?(x=w870) -> (x >= 0?=w869:bool)
                                n1318 = case shown="False" w869 {
                                tunnel: w871 -> [w873 w875]
                                frame False {
                                n1319 = local write "GPIB parsed msg from tester hid"(w873) -> ()
                                }
                                frame True {
                                n1320 = call <vilib>:"Space Constant.vi"() -> ("String"=w876:string)
                                n1321 = Match Pattern(string=w875, regular expression=w876) -> (before substring=w874:string)  [unwired: 1 in, 3 out]
                                n1322 = local write "GPIB parsed msg from tester hid"(w874) -> ()
                                }
                                }
                                }
                                frame True {
                                n1323 = Match Pattern(string=w878, regular expression=":") -> (before substring=w877:string)  [unwired: 1 in, 3 out]
                                n1324 = local write "GPIB parsed msg from tester hid"(w877) -> ()
                                }
                                }
                                }
                                frame True {
                                w881 = "?" ("regular expression")
                                n1325 = Match Pattern(string=w883, regular expression=w881) -> (before substring=w882:string)  [unwired: 1 in, 3 out]
                                n1326 = Concatenate Strings(w882, w881) -> (w880:string)
                                n1327 = local write "GPIB parsed msg from tester hid"(w880) -> ()
                                }
                                }
                                }
                                frame #1 {
                                n1328 = local read "GPIB parsed msg from tester hid"() -> (w884:string)
                                n1329 = case shown="\"ECHOOK\"" w884 {
                                frame "*IDN?" {
                                n1330 = local write "SC handler states hid"(SC_handler_states."responding to *IDN?" ("SC Test Interface States")) -> ()
                                }
                                frame "SITES?" {
                                n1331 = local read "Tester online"() -> (w888:bool)
                                n1332 = local read "POWER"() -> (w886:bool)
                                n1333 = Compound Arithmetic op=AND(w888, w886) -> (w887:bool)
                                n1334 = case shown="True" w887 {
                                frame False {
                                n1335 = local write "SC handler states hid"(SC_handler_states."closing bus" ("SC virtual handler states")) -> ()
                                }
                                frame True {
                                n1336 = flat-sequence {
                                frame #0 {
                                # "this could be a problem or uneccessary"
                                n1337 = while {
                                stop <- w891 stop-if-true
                                n1338 = local read "H1 Waiting"() -> (w893:bool)
                                n1339 = local read "H2 Waiting"() -> (w892:bool)
                                n1340 = Or(x=w893, y=w892) -> (x .or. y?=w891:bool)
                                n1341 = Wait (ms)(milliseconds to wait=u32 5) -> ()  [unwired: 1 out]
                                }
                                }
                                frame #1 {
                                n1342 = local write "SC handler states hid"(SC_handler_states."responding to SITES?" ("SC Test Interface States")) -> ()
                                }
                                }
                                }
                                }
                                }
                                frame "Fullsites?" {
                                n1343 = local write "SC handler states hid"(SC_handler_states."responding to Fullsites?" ("SC Test Interface States")) -> ()
                                }
                                frame "HIDN?" {
                                n1344 = local write "SC handler states hid"(SC_handler_states."responding to HIDN?" ("SC Test Interface States")) -> ()
                                }
                                frame "HAND?" {
                                n1345 = local write "SC handler states hid"(SC_handler_states."respond to HAND?" ("SC Test Interface States")) -> ()
                                }
                                frame "A BIN" {
                                n1346 = flat-sequence {
                                frame #0 {
                                n1347 = local read "Message from tester hid"() -> (w898:string)
                                n1348 = local write "Binning string from tester hid"(w898) -> ()
                                }
                                frame #1 {
                                n1349 = local write "SC handler states hid"(SC_handler_states."responding to A BIN" ("SC Test Interface States")) -> ()
                                }
                                }
                                }
                                frame "BINON" {
                                n1350 = flat-sequence {
                                frame #0 {
                                n1351 = local write "Binning string from tester hid"("") -> ()
                                }
                                frame #1 {
                                n1352 = local read "Message from tester hid"() -> (w903:string)
                                n1353 = local write "H1 Lock"(FALSE ("H1 Lock")) -> ()
                                n1354 = local write "H2 Lock"(FALSE ("H2 Lock")) -> ()
                                n1355 = local write "Binning string from tester hid"(w903) -> ()
                                }
                                frame #2 {
                                n1356 = local write "SC handler states hid"(SC_handler_states."responding to BINON" ("SC Test Interface States")) -> ()
                                }
                                }
                                }
                                frame "ECHOOK" {
                                n1357 = local write "SC handler states hid"(SC_handler_states."ECHOOK" ("SC Test Interface States")) -> ()
                                }
                                frame "ECHONG" {
                                n1358 = local write "SC handler states hid"(SC_handler_states."ECHONG" ("SC Test Interface States")) -> ()
                                }
                                frame Default {
                                n1359 = local write "SC handler states hid"(SC_handler_states."responding to unknown command" ("SC Test Interface States")) -> ()
                                }
                                }
                                }
                                }
                                }
                                }
                                }
                                }
                              }
                              frame "responding to *IDN?" {
                                n1360 = flat-sequence {
                                frame #0 {
                                n1361 = while {
                                stop <- w913 stop-if-true
                                w910 = "Sentinel Controller Handler Interface"
                                n1362 = local read "VISA bus 0 resource name out hid"() -> (w922:refnum<visa-resource-name>)
                                n1363 = local read "VISA bus 0 error out hid"() -> (w921:errorcluster)
                                n1364 = local read "GPIB Bus 0 traffic"() -> (w918:string)
                                n1365 = VISA Write(VISA resource name=w922, write buffer=w910, error in (no error)=w921) -> (VISA resource name out=w920:refnum<visa-resource-name>, return count=w914:u32, error out=w919:errorcluster)
                                n1366 = call <vilib>:"Trim Whitespace.vi"("string"=w910) -> ("trimmed string"=w911:string)  [unwired: 1 in]
                                n1367 = local write "VISA bus 0 resource name out hid"(w920) -> ()
                                n1368 = local write "VISA bus 0 error out hid"(w919) -> ()
                                n1369 = Unbundle By Name(w919) -> ("status"=w912:bool)
                                n1370 = Concatenate Strings(w918, "\r\n", "Bus 0 write: " ("string"), w911) -> (w916:string)
                                n1371 = Greater Than 0?(x=w914) -> (x > 0?=w913:bool)
                                n1372 = local write "GPIB bus 0 write error"(w912) -> ()
                                n1373 = local write "GPIB Bus 0 traffic"(w916) -> ()
                                }
                                }
                                frame #1 {
                                n1374 = local write "SC handler states hid"(SC_handler_states."waiting on event" ("SC Test Interface States")) -> ()
                                }
                                }
                              }
                              frame "respond to HAND?" {
                                n1375 = local read "H1 Lock"() -> (w926:bool)
                                n1376 = case shown="True" w926 {
                                frame False {
                                n1377 = local read "H2 Lock"() -> (w927:bool)
                                n1378 = case shown="True" w927 {
                                frame False {
                                n1379 = flat-sequence {
                                frame #0 {
                                n1380 = One Button Dialog(message="Fatal error 200:\nThe SC responded to a handler being ready with devices\nto test, but when the SC check for a lock when responding\nto *HAND?, no handler had a lock. \nPlease report this bug to Celerint at www.celerint.com  ") -> ()  [unwired: 1 in, 1 out]
                                }
                                frame #1 {
                                n1381 = local write "SC handler states hid"(SC_handler_states."closing bus" ("SC Test Interface States")) -> ()
                                }
                                }
                                }
                                frame True {
                                n1382 = flat-sequence {
                                frame #0 {
                                n1383 = while {
                                stop <- w933 stop-if-true
                                w931 = "H2" ("string")
                                n1384 = local read "VISA bus 0 resource name out hid"() -> (w939:refnum<visa-resource-name>)
                                n1385 = local read "GPIB Bus 0 traffic"() -> (w937:string)
                                n1386 = local read "VISA bus 0 error out hid"() -> (w938:errorcluster)
                                n1387 = call <vilib>:"Trim Whitespace.vi"("string"=w931) -> ("trimmed string"=w930:string)  [unwired: 1 in]
                                n1388 = VISA Write(VISA resource name=w939, write buffer=w931, error in (no error)=w938) -> (VISA resource name out=w940:refnum<visa-resource-name>, return count=w932:u32, error out=w941:errorcluster)
                                n1389 = Concatenate Strings(w937, "\r\n", "H2: Bus 0 write: " ("string"), w930) -> (w935:string)
                                n1390 = local write "VISA bus 0 error out hid"(w941) -> ()
                                n1391 = Unbundle By Name(w941) -> ("status"=w942:bool)
                                n1392 = local write "GPIB Bus 0 traffic"(w935) -> ()
                                n1393 = Greater Than 0?(x=w932) -> (x > 0?=w933:bool)
                                n1394 = local write "VISA bus 0 resource name out hid"(w940) -> ()
                                n1395 = local write "GPIB bus 0 write error"(w942) -> ()
                                }
                                }
                                frame #1 {
                                n1396 = local write "SC handler states hid"(SC_handler_states."waiting on event" ("SC Test Interface States")) -> ()
                                }
                                }
                                }
                                }
                                }
                                frame True {
                                n1397 = flat-sequence {
                                frame #0 {
                                n1398 = while {
                                stop <- w947 stop-if-true
                                w945 = "H1" ("string")
                                n1399 = local read "VISA bus 0 resource name out hid"() -> (w953:refnum<visa-resource-name>)
                                n1400 = local read "GPIB Bus 0 traffic"() -> (w951:string)
                                n1401 = local read "VISA bus 0 error out hid"() -> (w952:errorcluster)
                                n1402 = call <vilib>:"Trim Whitespace.vi"("string"=w945) -> ("trimmed string"=w944:string)  [unwired: 1 in]
                                n1403 = Concatenate Strings(w951, "\r\n", "H1: Bus 0 write: " ("string"), w944) -> (w949:string)
                                n1404 = VISA Write(VISA resource name=w953, write buffer=w945, error in (no error)=w952) -> (VISA resource name out=w954:refnum<visa-resource-name>, return count=w946:u32, error out=w955:errorcluster)
                                n1405 = local write "VISA bus 0 resource name out hid"(w954) -> ()
                                n1406 = local write "VISA bus 0 error out hid"(w955) -> ()
                                n1407 = Unbundle By Name(w955) -> ("status"=w956:bool)
                                n1408 = local write "GPIB Bus 0 traffic"(w949) -> ()
                                n1409 = Greater Than 0?(x=w946) -> (x > 0?=w947:bool)
                                n1410 = local write "GPIB bus 0 write error"(w956) -> ()
                                }
                                }
                                frame #1 {
                                n1411 = local write "SC handler states hid"(SC_handler_states."waiting on event" ("SC Test Interface States")) -> ()
                                }
                                }
                                }
                                }
                              }
                              frame "responding to HIDN?" {
                                n1412 = local read "H1 Lock"() -> (w960:bool)
                                n1413 = case shown="True" w960 {
                                frame False {
                                n1414 = local read "H2 Lock"() -> (w961:bool)
                                n1415 = case shown="True" w961 {
                                frame False {
                                n1416 = flat-sequence {
                                frame #0 {
                                n1417 = One Button Dialog(message="Fatal error 201:\nThe SC responded to a handler being ready with devices\nto test, but when the SC check for a lock when responding\nto *HIDN?, no handler had a lock. \nPlease report this bug to Celerint at www.celerint.com  ") -> ()  [unwired: 1 in, 1 out]
                                }
                                frame #1 {
                                n1418 = local write "SC handler states hid"(SC_handler_states."testing" ("SC Test Interface States")) -> ()
                                }
                                }
                                }
                                frame True {
                                n1419 = flat-sequence {
                                frame #0 {
                                n1420 = while {
                                stop <- w967 stop-if-true
                                n1421 = local read "VISA bus 0 resource name out hid"() -> (w973:refnum<visa-resource-name>)
                                n1422 = local read "H2 response to *HAND? hid"() -> (w965:string)
                                n1423 = local read "VISA bus 0 error out hid"() -> (w972:errorcluster)
                                n1424 = local read "GPIB Bus 0 traffic"() -> (w971:string)
                                n1425 = VISA Write(VISA resource name=w973, write buffer=w965, error in (no error)=w972) -> (VISA resource name out=w974:refnum<visa-resource-name>, return count=w966:u32, error out=w975:errorcluster)
                                n1426 = call <vilib>:"Trim Whitespace.vi"("string"=w965) -> ("trimmed string"=w964:string)  [unwired: 1 in]
                                n1427 = local write "VISA bus 0 error out hid"(w975) -> ()
                                n1428 = Unbundle By Name(w975) -> ("status"=w976:bool)
                                n1429 = Concatenate Strings(w971, "\r\n", "H2: Bus 0 write: " ("string"), w964) -> (w969:string)
                                n1430 = Greater Than 0?(x=w966) -> (x > 0?=w967:bool)
                                n1431 = local write "VISA bus 0 resource name out hid"(w974) -> ()
                                n1432 = local write "GPIB Bus 0 traffic"(w969) -> ()
                                n1433 = local write "GPIB bus 0 write error"(w976) -> ()
                                }
                                }
                                frame #1 {
                                n1434 = local write "SC handler states hid"(SC_handler_states."waiting on event" ("SC Test Interface States")) -> ()
                                }
                                }
                                }
                                }
                                }
                                frame True {
                                n1435 = flat-sequence {
                                frame #0 {
                                n1436 = while {
                                stop <- w981 stop-if-true
                                n1437 = local read "VISA bus 0 resource name out hid"() -> (w987:refnum<visa-resource-name>)
                                n1438 = local read "H1 response to *HAND? hid"() -> (w979:string)
                                n1439 = local read "VISA bus 0 error out hid"() -> (w986:errorcluster)
                                n1440 = local read "GPIB Bus 0 traffic"() -> (w985:string)
                                n1441 = call <vilib>:"Trim Whitespace.vi"("string"=w979) -> ("trimmed string"=w978:string)  [unwired: 1 in]
                                n1442 = VISA Write(VISA resource name=w987, write buffer=w979, error in (no error)=w986) -> (VISA resource name out=w988:refnum<visa-resource-name>, return count=w980:u32, error out=w989:errorcluster)
                                n1443 = local write "VISA bus 0 resource name out hid"(w988) -> ()
                                n1444 = local write "VISA bus 0 error out hid"(w989) -> ()
                                n1445 = Unbundle By Name(w989) -> ("status"=w990:bool)
                                n1446 = Concatenate Strings(w985, "\r\n", "H1: Bus 0 write: " ("string"), w978) -> (w983:string)
                                n1447 = Greater Than 0?(x=w980) -> (x > 0?=w981:bool)
                                n1448 = local write "GPIB Bus 0 traffic"(w983) -> ()
                                n1449 = local write "GPIB bus 0 write error"(w990) -> ()
                                }
                                }
                                frame #1 {
                                n1450 = local write "SC handler states hid"(SC_handler_states."waiting on event" ("SC Test Interface States")) -> ()
                                }
                                }
                                }
                                }
                              }
                              frame "responding to Fullsites?" {
                                n1451 = local read "Last locked handler hid"() -> (w992:enum16{"H1", "H2"})
                                n1452 = case shown="\"H1\", Default" w992 {
                                frame "H1", Default {
                                n1453 = flat-sequence {
                                frame #0 {
                                n1454 = while {
                                stop <- w1000 stop-if-true
                                n1455 = local read "VISA bus 0 resource name out hid"() -> (w998:refnum<visa-resource-name>)
                                n1456 = local read "VISA bus 0 error out hid"() -> (w997:errorcluster)
                                n1457 = local read "H1 FULLSITES? response hid"() -> (w1001:string)
                                n1458 = local read "GPIB Bus 0 traffic"() -> (w1003:string)
                                n1459 = call <vilib>:"Trim Whitespace.vi"("string"=w1001) -> ("trimmed string"=w1002:string)  [unwired: 1 in]
                                n1460 = VISA Write(VISA resource name=w998, write buffer=w1001, error in (no error)=w997) -> (return count=w999:u32, error out=w1007:errorcluster)  [unwired: 1 out]
                                n1461 = Wait (ms)(milliseconds to wait=u32 10) -> ()  [unwired: 1 out]
                                n1462 = Unbundle By Name(w1007) -> ("status"=w996:bool)
                                n1463 = local write "VISA bus 0 error out hid"(w1007) -> ()
                                n1464 = Concatenate Strings(w1003, "\r\n", "Bus 0 write: " ("string"), w1002) -> (w1005:string)
                                n1465 = local write "GPIB bus 0 write error"(w996) -> ()
                                n1466 = local write "GPIB Bus 0 traffic"(w1005) -> ()
                                n1467 = Greater Than 0?(x=w999) -> (x > 0?=w1000:bool)
                                }
                                }
                                frame #1 {
                                n1468 = local write "SC handler states hid"(SC_handler_states."testing" ("SC Test Interface States")) -> ()
                                }
                                }
                                }
                                frame "H2" {
                                n1469 = flat-sequence {
                                frame #0 {
                                n1470 = while {
                                stop <- w1013 stop-if-true
                                n1471 = local read "VISA bus 0 resource name out hid"() -> (w1010:refnum<visa-resource-name>)
                                n1472 = local read "H2 FULLSITES? response hid"() -> (w1014:string)
                                n1473 = local read "VISA bus 0 error out hid"() -> (w1011:errorcluster)
                                n1474 = local read "GPIB Bus 0 traffic"() -> (w1016:string)
                                n1475 = VISA Write(VISA resource name=w1010, write buffer=w1014, error in (no error)=w1011) -> (return count=w1012:u32, error out=w1020:errorcluster)  [unwired: 1 out]
                                n1476 = call <vilib>:"Trim Whitespace.vi"("string"=w1014) -> ("trimmed string"=w1015:string)  [unwired: 1 in]
                                n1477 = local write "VISA bus 0 error out hid"(w1020) -> ()
                                n1478 = Unbundle By Name(w1020) -> ("status"=w1021:bool)
                                n1479 = Wait (ms)(milliseconds to wait=u32 10) -> ()  [unwired: 1 out]
                                n1480 = Concatenate Strings(w1016, "\r\n", "Bus 0 write: " ("string"), w1015) -> (w1018:string)
                                n1481 = local write "GPIB bus 0 write error"(w1021) -> ()
                                n1482 = local write "GPIB Bus 0 traffic"(w1018) -> ()
                                n1483 = Greater Than 0?(x=w1012) -> (x > 0?=w1013:bool)
                                }
                                }
                                frame #1 {
                                n1484 = local write "SC handler states hid"(SC_handler_states."testing" ("SC Test Interface States")) -> ()
                                }
                                }
                                }
                                }
                              }
                              frame "testing" {
                                n1485 = flat-sequence {
                                tunnel: w1033 -> [w1037]
                                tunnel: w1034 -> [w1038]
                                tunnel: [w1036] -> w1030
                                tunnel: [w1035] -> w1029
                                tunnel: w1030 -> [w1052]
                                tunnel: [w1052] -> w1028
                                tunnel: w1029 -> [w1051]
                                tunnel: [w1051] -> w1027
                                tunnel: w1028 -> [w1054]
                                tunnel: w1027 -> [w1053]
                                tunnel: [w1054] -> w1026
                                tunnel: [w1053] -> w1025
                                tunnel: w1026 -> [w1063]
                                tunnel: w1025 -> [w1062]
                                tunnel: [w1063] -> w1024
                                tunnel: [w1062] -> w1023
                                tunnel: [w1065] -> w1032
                                tunnel: [w1066] -> w1031
                                tunnel: w1024 -> [w1066]
                                tunnel: w1023 -> [w1065]
                                frame #0 {
                                n1486 = local read "SC measured test time hid"() -> (w1039:dbl)
                                n1487 = local read "SC measured wait time hid"() -> (w1040:dbl)
                                n1488 = local read "Tester loop counter hid"() -> (w1042:u32)
                                n1489 = Add(x=w1039, y=w1040) -> (x+y=w1046:dbl)
                                n1490 = local read "Utilization averaging"() -> (w1041:i32)
                                n1491 = Divide(x=w1039, y=w1046) -> (x/y=w1047:dbl)
                                n1492 = Multiply(x=100.0, y=w1047) -> (x*y=w1043:dbl)
                                n1493 = call "moving_avg_core.vi"("Array in"=w1037, "avg"=w1041, "accumulator in"=w1038, "i"=w1042, "data in"=w1043) -> ("Array out"=w1036:dbl[], "accumulator out"=w1035:dbl, "rolling avg out"=w1044:dbl)  [unwired: 4 in]
                                n1494 = Bundle(w1043, "rolling avg out"=w1044) -> (w1045:cluster{dbl, "rolling avg out":dbl})  [unwired: 1 in]
                                n1495 = local write "Sys utilization"(w1044) -> ()
                                n1496 = local write "SysUtilMon"(w1045) -> ()
                                }
                                frame #1 {
                                # "empty binning string wiill hold handlers at BINON until valid"
                                n1497 = local read "H1 loop counter hid"() -> (w1049:u32)
                                n1498 = Increment(x=w1049) -> (x+1=w1050:u32)
                                n1499 = local write "H1 loop counter hid"(w1050) -> ()
                                }
                                frame #2 {
                                n1500 = Tick Count (ms)() -> (millisecond timer value=w1056:u32)
                                n1501 = Tick Count (ms)() -> (millisecond timer value=w1055:u32)
                                n1502 = local write "tester wt end hid"(w1056) -> ()
                                n1503 = local write "tester tt start hid"(w1055) -> ()
                                }
                                frame #3 {
                                n1504 = local read "tester wt start hid"() -> (w1060:u32)
                                n1505 = local read "tester wt end hid"() -> (w1061:u32)
                                n1506 = Subtract(x=w1061, y=w1060) -> (x-y=w1059:u32)
                                n1507 = Divide(x=w1059, y=u32 1000) -> (x/y=w1057:dbl)
                                n1508 = local write "SC measured wait time hid"(w1057) -> ()
                                }
                                frame #4 {
                                n1509 = local write "SC handler states hid"(SC_handler_states."waiting on event" ("SC Test Interface States")) -> ()
                                }
                                }
                              }
                              frame "responding to SITES?" {
                                n1510 = flat-sequence {
                                frame #0 {
                                # "This is the engine that decides if H1 is checked first or H2"
                                n1511 = local read "Last locked handler hid"() -> (w1069:enum16{"H1", "H2"})
                                n1512 = case shown="\"H2\"" w1069 {
                                frame "H1", Default {
                                n1513 = local read "H2 Waiting"() -> (w1070:bool)
                                n1514 = case shown="False" w1070 {
                                frame False {
                                n1515 = local read "H1 Waiting"() -> (w1071:bool)
                                n1516 = case shown="True" w1071 {
                                frame False {
                                # "end up here only if neither handler is waiting and ready"
                                }
                                frame True {
                                n1517 = flat-sequence {
                                frame #0 {
                                n1518 = local write "H2 Lock"(FALSE ("H1 Lock")) -> ()
                                n1519 = local write "H1 Lock"(TRUE ("H1 Lock")) -> ()
                                n1520 = local write "Last locked handler hid"(enum16{"H1", "H2"}."H1" ("Last locked handler")) -> ()
                                }
                                frame #1 {
                                n1521 = while {
                                stop <- w1077 stop-if-true
                                n1522 = local read "VISA bus 0 resource name out hid"() -> (w1085:refnum<visa-resource-name>)
                                n1523 = local read "VISA bus 0 error out hid"() -> (w1086:errorcluster)
                                n1524 = local read "H1 SITES? response hid"() -> (w1075:string)
                                n1525 = call <vilib>:"Trim Whitespace.vi"("string"=w1075) -> ("trimmed string"=w1076:string)  [unwired: 1 in]
                                n1526 = VISA Write(VISA resource name=w1085, write buffer=w1075, error in (no error)=w1086) -> (VISA resource name out=w1084:refnum<visa-resource-name>, return count=w1078:u32, error out=w1083:errorcluster)
                                n1527 = local write "VISA bus 0 resource name out hid"(w1084) -> ()
                                n1528 = Unbundle By Name(w1083) -> ("status"=w1087:bool)
                                n1529 = local write "VISA bus 0 error out hid"(w1083) -> ()
                                n1530 = Greater Than 0?(x=w1078) -> (x > 0?=w1077:bool)
                                n1531 = local write "GPIB bus 0 write error"(w1087) -> ()
                                n1532 = Concatenate Strings("H1: Tester test cycle start" ("string"), "\r\n", "Bus 0 write: " ("string"), w1076) -> (w1081:string)
                                n1533 = local write "GPIB Bus 0 traffic"(w1081) -> ()
                                }
                                }
                                }
                                }
                                }
                                }
                                frame True {
                                n1534 = flat-sequence {
                                frame #0 {
                                n1535 = local write "H2 Lock"(TRUE ("H1 Lock")) -> ()
                                n1536 = local write "H1 Lock"(FALSE ("H1 Lock")) -> ()
                                n1537 = local write "Last locked handler hid"(enum16{"H1", "H2"}."H2" ("Last locked handler")) -> ()
                                }
                                frame #1 {
                                n1538 = while {
                                stop <- w1094 stop-if-true
                                n1539 = local read "VISA bus 0 resource name out hid"() -> (w1101:refnum<visa-resource-name>)
                                n1540 = local read "VISA bus 0 error out hid"() -> (w1102:errorcluster)
                                n1541 = local read "H2 SITES? response hid"() -> (w1091:string)
                                n1542 = call <vilib>:"Trim Whitespace.vi"("string"=w1091) -> ("trimmed string"=w1092:string)  [unwired: 1 in]
                                n1543 = VISA Write(VISA resource name=w1101, write buffer=w1091, error in (no error)=w1102) -> (VISA resource name out=w1100:refnum<visa-resource-name>, return count=w1093:u32, error out=w1099:errorcluster)
                                n1544 = local write "VISA bus 0 resource name out hid"(w1100) -> ()
                                n1545 = Unbundle By Name(w1099) -> ("status"=w1103:bool)
                                n1546 = local write "VISA bus 0 error out hid"(w1099) -> ()
                                n1547 = Greater Than 0?(x=w1093) -> (x > 0?=w1094:bool)
                                n1548 = local write "GPIB bus 0 write error"(w1103) -> ()
                                n1549 = Concatenate Strings("H2: Tester test cycle start" ("string"), "\r\n", "Bus 0 write: " ("string"), w1092) -> (w1097:string)
                                n1550 = local write "GPIB Bus 0 traffic"(w1097) -> ()
                                }
                                }
                                frame #2 {
                                n1551 = local read "H2 loop counter hid"() -> (w1104:u32)
                                n1552 = Increment(x=w1104) -> (x+1=w1105:u32)
                                n1553 = local write "H2 loop counter hid"(w1105) -> ()
                                }
                                }
                                }
                                }
                                }
                                frame "H2" {
                                n1554 = local read "H1 Waiting"() -> (w1106:bool)
                                n1555 = case shown="True" w1106 {
                                frame False {
                                n1556 = local read "H2 Waiting"() -> (w1107:bool)
                                n1557 = case shown="True" w1107 {
                                frame False {
                                # "end up here only if neither handler is waiting and ready"
                                }
                                frame True {
                                n1558 = flat-sequence {
                                frame #0 {
                                n1559 = local write "H2 Lock"(TRUE ("H1 Lock")) -> ()
                                n1560 = local write "H1 Lock"(FALSE ("H1 Lock")) -> ()
                                n1561 = local write "Last locked handler hid"(enum16{"H1", "H2"}."H2" ("Last locked handler")) -> ()
                                }
                                frame #1 {
                                n1562 = while {
                                stop <- w1114 stop-if-true
                                n1563 = local read "VISA bus 0 resource name out hid"() -> (w1121:refnum<visa-resource-name>)
                                n1564 = local read "VISA bus 0 error out hid"() -> (w1122:errorcluster)
                                n1565 = local read "H2 SITES? response hid"() -> (w1111:string)
                                n1566 = call <vilib>:"Trim Whitespace.vi"("string"=w1111) -> ("trimmed string"=w1112:string)  [unwired: 1 in]
                                n1567 = VISA Write(VISA resource name=w1121, write buffer=w1111, error in (no error)=w1122) -> (VISA resource name out=w1120:refnum<visa-resource-name>, return count=w1113:u32, error out=w1119:errorcluster)
                                n1568 = local write "VISA bus 0 resource name out hid"(w1120) -> ()
                                n1569 = Unbundle By Name(w1119) -> ("status"=w1123:bool)
                                n1570 = local write "VISA bus 0 error out hid"(w1119) -> ()
                                n1571 = Greater Than 0?(x=w1113) -> (x > 0?=w1114:bool)
                                n1572 = local write "GPIB bus 0 write error"(w1123) -> ()
                                n1573 = Concatenate Strings("H2: Tester test cycle start" ("string"), "\r\n", "Bus 0 write: " ("string"), w1112) -> (w1117:string)
                                n1574 = local write "GPIB Bus 0 traffic"(w1117) -> ()
                                }
                                }
                                frame #2 {
                                n1575 = local read "H2 loop counter hid"() -> (w1124:u32)
                                n1576 = Increment(x=w1124) -> (x+1=w1125:u32)
                                n1577 = local write "H2 loop counter hid"(w1125) -> ()
                                }
                                }
                                }
                                }
                                }
                                frame True {
                                n1578 = flat-sequence {
                                frame #0 {
                                n1579 = local write "Last locked handler hid"(enum16{"H1", "H2"}."H1" ("Last locked handler")) -> ()
                                }
                                frame #1 {
                                n1580 = while {
                                stop <- w1129 stop-if-true
                                n1581 = local read "VISA bus 0 resource name out hid"() -> (w1137:refnum<visa-resource-name>)
                                n1582 = local read "VISA bus 0 error out hid"() -> (w1138:errorcluster)
                                n1583 = local read "H1 SITES? response hid"() -> (w1127:string)
                                n1584 = call <vilib>:"Trim Whitespace.vi"("string"=w1127) -> ("trimmed string"=w1128:string)  [unwired: 1 in]
                                n1585 = VISA Write(VISA resource name=w1137, write buffer=w1127, error in (no error)=w1138) -> (VISA resource name out=w1136:refnum<visa-resource-name>, return count=w1130:u32, error out=w1135:errorcluster)
                                n1586 = local write "VISA bus 0 resource name out hid"(w1136) -> ()
                                n1587 = Unbundle By Name(w1135) -> ("status"=w1139:bool)
                                n1588 = local write "VISA bus 0 error out hid"(w1135) -> ()
                                n1589 = Greater Than 0?(x=w1130) -> (x > 0?=w1129:bool)
                                n1590 = local write "GPIB bus 0 write error"(w1139) -> ()
                                n1591 = Concatenate Strings("H1: Tester test cycle start" ("string"), "\r\n", "Bus 0 write: " ("string"), w1128) -> (w1133:string)
                                n1592 = local write "GPIB Bus 0 traffic"(w1133) -> ()
                                }
                                }
                                frame #2 {
                                n1593 = local read "H1 loop counter hid"() -> (w1141:u32)
                                n1594 = Increment(x=w1141) -> (x+1=w1140:u32)
                                n1595 = local write "H1 loop counter hid"(w1140) -> ()
                                }
                                }
                                }
                                }
                                }
                                }
                                }
                                frame #1 {
                                n1596 = local write "SC handler states hid"(SC_handler_states."testing" ("SC Test Interface States")) -> ()
                                }
                                }
                              }
                              frame "responding to A BIN" {
                                n1597 = flat-sequence {
                                frame #0 {
                                n1598 = local read "H1 Lock"() -> (w1145:bool)
                                n1599 = case shown="True" w1145 {
                                frame False {
                                n1600 = local read "H2 Lock"() -> (w1146:bool)
                                n1601 = case shown="True" w1146 {
                                frame False {
                                }
                                frame True {
                                n1602 = local read "GPIB Bus 0 traffic"() -> (w1150:string)
                                n1603 = Concatenate Strings(w1150, "\r\n", "Bus 0: binning" ("string")) -> (w1148:string)
                                n1604 = local write "GPIB Bus 0 traffic"(w1148) -> ()
                                }
                                }
                                }
                                frame True {
                                n1605 = local read "GPIB Bus 0 traffic"() -> (w1154:string)
                                n1606 = Concatenate Strings(w1154, "\r\n", "Bus 0: binning" ("string")) -> (w1152:string)
                                n1607 = local write "GPIB Bus 0 traffic"(w1152) -> ()
                                }
                                }
                                }
                                frame #1 {
                                n1608 = Tick Count (ms)() -> (millisecond timer value=w1156:u32)
                                n1609 = Tick Count (ms)() -> (millisecond timer value=w1155:u32)
                                n1610 = local write "tester tt end hid"(w1156) -> ()
                                n1611 = local write "tester wt start hid"(w1155) -> ()
                                }
                                frame #2 {
                                n1612 = local read "tester tt start hid"() -> (w1160:u32)
                                n1613 = local read "tester tt end hid"() -> (w1161:u32)
                                n1614 = Subtract(x=w1161, y=w1160) -> (x-y=w1159:u32)
                                n1615 = Divide(x=w1159, y=u32 1000) -> (x/y=w1157:dbl)
                                n1616 = local write "SC measured test time hid"(w1157) -> ()
                                }
                                frame #3 {
                                n1617 = local read "H1 Lock"() -> (w1162:bool)
                                n1618 = case shown="False" w1162 {
                                frame False {
                                n1619 = local read "H2 Lock"() -> (w1163:bool)
                                n1620 = case shown="False" w1163 {
                                frame False {
                                n1621 = One Button Dialog(message="Fatal error 202:\nThe SC responded to a handler being ready with devices\nto test, but when the SC received binning data, no handler had a lock. \nPlease report this bug to Celerint at www.celerint.com  ") -> ()  [unwired: 1 in, 1 out]
                                }
                                frame True {
                                n1622 = local read "H2 online"() -> (w1184:bool)
                                n1623 = local read "Tandem\nfloorspace area"() -> (w1167:i32)
                                n1624 = local read "Std cell \nfloorspace area"() -> (w1195:i32)
                                n1625 = case shown="True" w1184 {
                                tunnel: [0 w1199] -> w1185
                                frame False {
                                }
                                frame True {
                                n1626 = local read "H2 UPH"() -> (w1200:cluster{u32, u32})
                                n1627 = Unbundle(w1200) -> (w1199:u32)  [unwired: 1 out]
                                }
                                }
                                n1628 = local read "System UPH"() -> (w1166:u32)
                                n1629 = local read "UPH"() -> (w1196:dbl)
                                n1630 = Divide(x=w1166, y=w1167) -> (x/y=w1165:dbl)
                                n1631 = local write "Tandem UPH\nper unit area"(w1165) -> ()
                                n1632 = Divide(x=w1196, y=w1195) -> (x/y=w1197:dbl)
                                n1633 = local read "Std hourly\ncost ($/hr)"() -> (w1192:dbl)
                                n1634 = local read "H1 UPH"() -> (w1194:cluster{u32, u32})
                                n1635 = local write "H1 UPH per unit area"(w1197) -> ()
                                n1636 = local read "Utilization (%)"() -> (w1177:u32)
                                n1637 = local read "Tandem hourly\ncost ($/hr)"() -> (w1193:dbl)
                                n1638 = local read "# of devices to test"() -> (w1183:u32)
                                n1639 = Unbundle(w1194) -> (w1186:u32)  [unwired: 1 out]
                                n1640 = local read "Hours per month"() -> (w1178:i32)
                                n1641 = local write "Calc H2 UPH"(w1185) -> ()
                                n1642 = local write "Calc H1 UPH"(w1186) -> ()
                                n1643 = local read "UPH"() -> (w1191:dbl)
                                n1644 = Add(x=w1186, y=w1185) -> (x+y=w1173:u32)
                                n1645 = Divide(x=w1177, y=u32 100) -> (x/y=w1176:dbl)
                                n1646 = Divide(x=w1183, y=w1173) -> (x/y=w1182:dbl)
                                n1647 = Multiply(x=w1178, y=w1176) -> (x*y=w1174:dbl)
                                n1648 = Divide(x=w1192, y=w1191) -> (x/y=w1190:dbl)
                                n1649 = Divide(x=w1193, y=w1173) -> (x/y=w1188:dbl)
                                n1650 = local write "System UPH"(w1173) -> ()
                                n1651 = local write "Calc\nsystem UPH"(w1173) -> ()
                                n1652 = local read "# of devices to test"() -> (w1171:u32)
                                n1653 = Divide(x=w1182, y=w1174) -> (x/y=w1181:dbl)
                                n1654 = Multiply(x=w1190, y=100.0) -> (x*y=w1169:dbl)
                                n1655 = Multiply(x=w1188, y=100.0) -> (x*y=w1168:dbl)
                                n1656 = local write "Std unit cost\n(cents/device)"(w1169) -> ()
                                n1657 = local write "Tandem unit cost\n(cents/device)"(w1168) -> ()
                                n1658 = Subtract(x=w1169, y=w1168) -> (x-y=w1172:dbl)
                                n1659 = Multiply(x=w1181, y=30) -> (x*y=w1179:dbl)
                                n1660 = Multiply(x=w1171, y=w1172) -> (x*y=w1170:dbl)
                                n1661 = local write "Calendar days required\nfor testing all units"(w1179) -> ()
                                n1662 = local write "$ saved"(w1170) -> ()
                                }
                                }
                                }
                                frame True {
                                n1663 = local read "H1 online"() -> (w1221:bool)
                                n1664 = local read "Tandem\nfloorspace area"() -> (w1233:i32)
                                n1665 = local read "Std cell \nfloorspace area"() -> (w1226:i32)
                                n1666 = case shown="True" w1221 {
                                tunnel: [0 w1235] -> w1201
                                frame False {
                                }
                                frame True {
                                n1667 = local read "H1 UPH"() -> (w1236:cluster{u32, u32})
                                n1668 = Unbundle(w1236) -> (w1235:u32)  [unwired: 1 out]
                                }
                                }
                                n1669 = local read "System UPH"() -> (w1232:u32)
                                n1670 = local read "H2 calc UPH"() -> (w1227:dbl)
                                n1671 = Divide(x=w1232, y=w1233) -> (x/y=w1204:dbl)
                                n1672 = Divide(x=w1227, y=w1226) -> (x/y=w1205:dbl)
                                n1673 = local write "Tandem UPH\nper unit area"(w1204) -> ()
                                n1674 = local write "H2 UPH per unit area"(w1205) -> ()
                                n1675 = local read "Std hourly\ncost ($/hr)"() -> (w1229:dbl)
                                n1676 = local read "H2 UPH"() -> (w1231:cluster{u32, u32})
                                n1677 = local read "Utilization (%)"() -> (w1211:u32)
                                n1678 = local read "Tandem hourly\ncost ($/hr)"() -> (w1230:dbl)
                                n1679 = local read "# of devices to test"() -> (w1217:u32)
                                n1680 = local read "Hours per month"() -> (w1212:i32)
                                n1681 = Unbundle(w1231) -> (w1207:u32)  [unwired: 1 out]
                                n1682 = local write "Calc H1 UPH"(w1201) -> ()
                                n1683 = local write "Calc H2 UPH"(w1207) -> ()
                                n1684 = local read "UPH"() -> (w1228:dbl)
                                n1685 = Add(x=w1201, y=w1207) -> (x+y=w1206:u32)
                                n1686 = Divide(x=w1211, y=u32 100) -> (x/y=w1210:dbl)
                                n1687 = local write "System UPH"(w1206) -> ()
                                n1688 = local write "Calc\nsystem UPH"(w1206) -> ()
                                n1689 = Divide(x=w1217, y=w1206) -> (x/y=w1216:dbl)
                                n1690 = Multiply(x=w1212, y=w1210) -> (x*y=w1208:dbl)
                                n1691 = Divide(x=w1229, y=w1228) -> (x/y=w1225:dbl)
                                n1692 = Divide(x=w1230, y=w1206) -> (x/y=w1223:dbl)
                                n1693 = local read "# of devices to test"() -> (w1219:u32)
                                n1694 = Divide(x=w1216, y=w1208) -> (x/y=w1215:dbl)
                                n1695 = Multiply(x=w1225, y=100.0) -> (x*y=w1203:dbl)
                                n1696 = Multiply(x=w1223, y=100.0) -> (x*y=w1202:dbl)
                                n1697 = local write "Std unit cost\n(cents/device)"(w1203) -> ()
                                n1698 = local write "Tandem unit cost\n(cents/device)"(w1202) -> ()
                                n1699 = Subtract(x=w1203, y=w1202) -> (x-y=w1220:dbl)
                                n1700 = Multiply(x=w1215, y=30) -> (x*y=w1213:dbl)
                                n1701 = Multiply(x=w1219, y=w1220) -> (x*y=w1218:dbl)
                                n1702 = local write "Calendar days required\nfor testing all units"(w1213) -> ()
                                n1703 = local write "$ saved"(w1218) -> ()
                                }
                                }
                                }
                                frame #4 {
                                # "when this loop unlocks the handlers,\nthe handler interface loops are free to continue\nto send the binning information to their\nrespective handlers.  Each handler interface \nloop using the \"binning string hidden\" to do\nthis.  That is why, here, there is no writing of\nthe binning informatrion to a handler.  \nThat is done in the handler interface loops."
                                n1704 = local write "H1 Lock"(FALSE ("H1 Lock")) -> ()
                                n1705 = local write "H2 Lock"(FALSE ("H1 Lock")) -> ()
                                }
                                frame #5 {
                                n1706 = local read "Tester online"() -> (w1239:bool)
                                n1707 = local read "POWER"() -> (w1241:bool)
                                n1708 = Compound Arithmetic op=AND(w1239, w1241) -> (w1240:bool)
                                n1709 = case shown="True" w1240 {
                                frame False {
                                n1710 = local write "SC handler states hid"(SC_handler_states."closing bus" ("SC virtual handler states")) -> ()
                                }
                                frame True {
                                n1711 = local write "SC handler states hid"(SC_handler_states."waiting on event" ("SC virtual handler states")) -> ()
                                }
                                }
                                }
                                }
                              }
                              frame "responding to BINON" {
                                n1712 = local read "Last locked handler hid"() -> (w1244:enum16{"H1", "H2"})
                                n1713 = case shown="\"H1\", Default" w1244 {
                                frame "H1", Default {
                                n1714 = flat-sequence {
                                tunnel: [w1257] -> w1249
                                tunnel: [w1256] -> w1248
                                tunnel: [w1265] -> w1247
                                tunnel: w1248 -> [w1266]
                                tunnel: w1249 -> [w1267]
                                tunnel: w1247 -> [w1284]
                                frame #0 {
                                n1715 = while {
                                stop <- w1251 stop-if-true
                                n1716 = local read "NS6040 tester states H1 hid"() -> (w1253:T3)
                                n1717 = Wait (ms)(milliseconds to wait=u32 10) -> ()  [unwired: 1 out]
                                n1718 = Equal?(x=w1253, y=SC_NS6040_tester_states_v2."binning") -> (x = y?=w1251:bool)
                                }
                                }
                                frame #1 {
                                # "write binning to active handler"
                                n1719 = local read "VISA bus 1 resource name out hid"() -> (w1263:refnum<visa-resource-name>)
                                n1720 = local read "Binning string from tester hid"() -> (w1254:string)
                                n1721 = local read "VISA bus 1 error out hid"() -> (w1264:errorcluster)
                                n1722 = local read "GPIB bus 1 traffic"() -> (w1261:string)
                                n1723 = call <vilib>:"Trim Whitespace.vi"("string"=w1254) -> ("trimmed string"=w1255:string)  [unwired: 1 in]
                                n1724 = VISA Write(VISA resource name=w1263, write buffer=w1254, error in (no error)=w1264) -> (VISA resource name out=w1256:refnum<visa-resource-name>, error out=w1257:errorcluster)  [unwired: 1 out]
                                n1725 = local write "VISA bus 1 error out hid"(w1257) -> ()
                                n1726 = Unbundle By Name(w1257) -> ("status"=w1262:bool)
                                n1727 = Concatenate Strings(w1261, "\r\n", "Bus 1 write: " ("string"), w1255) -> (w1259:string)
                                n1728 = local write "GPIB bus 1 write error"(w1262) -> ()
                                n1729 = local write "GPIB bus 1 traffic"(w1259) -> ()
                                }
                                frame #2 {
                                # "read echo from active handler"
                                n1730 = while {
                                tunnel: w1267 -> [w1283]
                                tunnel: w1266 -> [w1282]
                                tunnel: [w1272] -> w1265
                                stop <- w1269 stop-if-true
                                n1731 = local read "GPIB bus 1 traffic"() -> (w1275:string)
                                n1732 = VISA Read(VISA resource name=w1282, byte count=u32 128, error in (no error)=w1283) -> (VISA resource name out=w1280:refnum<visa-resource-name>, read buffer=w1272:string, error out=w1279:errorcluster)  [unwired: 1 out]
                                n1733 = local write "VISA bus 1 resource name out hid"(w1280) -> ()
                                n1734 = Unbundle By Name(w1279) -> ("status"=w1274:bool)
                                n1735 = call <vilib>:"Trim Whitespace.vi"("string"=w1272) -> ("trimmed string"=w1273:string)  [unwired: 1 in]
                                n1736 = local write "GPIB bus 1 read error"(w1274) -> ()
                                n1737 = Match True/False String(2:"X" ("false string"), 3:"ECHO" ("true string"), 4:w1272) -> (0:w1269:bool)  [unwired: 1 out]
                                n1738 = Concatenate Strings(w1275, "\r\n", "Bus 1 read: " ("string"), w1273) -> (w1277:string)
                                n1739 = local write "GPIB bus 1 traffic"(w1277) -> ()
                                n1740 = Wait (ms)(milliseconds to wait=u32 5) -> ()  [unwired: 1 out]
                                }
                                }
                                frame #3 {
                                # "write echo back to H1"
                                n1741 = call <vilib>:"Trim Whitespace.vi"("string"=w1284) -> ("trimmed string"=w1285:string)  [unwired: 1 in]
                                n1742 = local read "GPIB Bus 0 traffic"() -> (w1290:string)
                                n1743 = local read "VISA bus 0 resource name out hid"() -> (w1294:refnum<visa-resource-name>)
                                n1744 = local read "VISA bus 0 error out hid"() -> (w1293:errorcluster)
                                n1745 = Concatenate Strings(w1290, "\r\n", "Bus 0 write: " ("string"), w1285) -> (w1288:string)
                                n1746 = local write "GPIB Bus 0 traffic"(w1288) -> ()
                                n1747 = VISA Write(VISA resource name=w1294, write buffer=w1284, error in (no error)=w1293) -> (VISA resource name out=w1292:refnum<visa-resource-name>, error out=w1291:errorcluster)  [unwired: 1 out]
                                n1748 = local write "VISA bus 0 resource name out hid"(w1292) -> ()
                                n1749 = Unbundle By Name(w1291) -> ("status"=w1286:bool)
                                n1750 = local write "VISA bus 0 error out hid"(w1291) -> ()
                                n1751 = local write "GPIB bus 0 write error"(w1286) -> ()
                                }
                                frame #4 {
                                # "go wait for results from tester:\nECHONG\nECHOOK\nActive handler is waiting for\nEcho state of tester to become\nECHOOK"
                                n1752 = local write "SC handler states hid"(SC_handler_states."waiting on event" ("SC Test Interface States")) -> ()
                                }
                                }
                                }
                                frame "H2" {
                                n1753 = flat-sequence {
                                tunnel: [w1306] -> w1298
                                tunnel: [w1305] -> w1297
                                tunnel: [w1314] -> w1296
                                tunnel: w1297 -> [w1315]
                                tunnel: w1298 -> [w1316]
                                tunnel: w1296 -> [w1333]
                                frame #0 {
                                n1754 = while {
                                stop <- w1301 stop-if-true
                                n1755 = local read "NS6040 tester states H2 hid"() -> (w1299:T3)
                                n1756 = Wait (ms)(milliseconds to wait=u32 10) -> ()  [unwired: 1 out]
                                n1757 = Equal?(x=w1299, y=SC_NS6040_tester_states_v2."binning") -> (x = y?=w1301:bool)
                                }
                                }
                                frame #1 {
                                n1758 = local read "VISA bus 2 resource name out hid"() -> (w1312:refnum<visa-resource-name>)
                                n1759 = local read "Binning string from tester hid"() -> (w1303:string)
                                n1760 = local read "VISA bus 2 error out hid"() -> (w1313:errorcluster)
                                n1761 = local read "GPIB bus 2 traffic"() -> (w1310:string)
                                n1762 = call <vilib>:"Trim Whitespace.vi"("string"=w1303) -> ("trimmed string"=w1304:string)  [unwired: 1 in]
                                n1763 = VISA Write(VISA resource name=w1312, write buffer=w1303, error in (no error)=w1313) -> (VISA resource name out=w1306:refnum<visa-resource-name>, error out=w1305:errorcluster)  [unwired: 1 out]
                                n1764 = local write "VISA bus 2 error out hid"(w1305) -> ()
                                n1765 = Unbundle By Name(w1305) -> ("status"=w1311:bool)
                                n1766 = Concatenate Strings(w1310, "\r\n", "Bus 2 write: " ("string"), w1304) -> (w1308:string)
                                n1767 = local write "GPIB bus 2 write error"(w1311) -> ()
                                n1768 = local write "GPIB bus 2 traffic"(w1308) -> ()
                                }
                                frame #2 {
                                n1769 = while {
                                tunnel: w1316 -> [w1332]
                                tunnel: w1315 -> [w1331]
                                tunnel: [w1319] -> w1314
                                stop <- w1318 stop-if-true
                                n1770 = local read "GPIB bus 2 traffic"() -> (w1324:string)
                                n1771 = VISA Read(VISA resource name=w1332, byte count=u32 128, error in (no error)=w1331) -> (VISA resource name out=w1329:refnum<visa-resource-name>, read buffer=w1319:string, error out=w1328:errorcluster)  [unwired: 1 out]
                                n1772 = local write "VISA bus 2 resource name out hid"(w1329) -> ()
                                n1773 = Unbundle By Name(w1328) -> ("status"=w1323:bool)
                                n1774 = call <vilib>:"Trim Whitespace.vi"("string"=w1319) -> ("trimmed string"=w1322:string)  [unwired: 1 in]
                                n1775 = local write "GPIB bus 2 read error"(w1323) -> ()
                                n1776 = Match True/False String(2:"X" ("false string"), 3:"ECHO" ("true string"), 4:w1319) -> (0:w1318:bool)  [unwired: 1 out]
                                n1777 = Concatenate Strings(w1324, "\r\n", "Bus 2 read: " ("string"), w1322) -> (w1326:string)
                                n1778 = local write "GPIB bus 2 traffic"(w1326) -> ()
                                n1779 = Wait (ms)(milliseconds to wait=u32 5) -> ()  [unwired: 1 out]
                                }
                                }
                                frame #3 {
                                n1780 = call <vilib>:"Trim Whitespace.vi"("string"=w1333) -> ("trimmed string"=w1335:string)  [unwired: 1 in]
                                n1781 = local read "GPIB Bus 0 traffic"() -> (w1334:string)
                                n1782 = local read "VISA bus 0 resource name out hid"() -> (w1341:refnum<visa-resource-name>)
                                n1783 = local read "VISA bus 0 error out hid"() -> (w1342:errorcluster)
                                n1784 = Concatenate Strings(w1334, "\r\n", "Bus 0 write: " ("string"), w1335) -> (w1337:string)
                                n1785 = local write "GPIB Bus 0 traffic"(w1337) -> ()
                                n1786 = VISA Write(VISA resource name=w1341, write buffer=w1333, error in (no error)=w1342) -> (VISA resource name out=w1340:refnum<visa-resource-name>, error out=w1339:errorcluster)  [unwired: 1 out]
                                n1787 = Unbundle By Name(w1339) -> ("status"=w1343:bool)
                                n1788 = local write "VISA bus 0 resource name out hid"(w1340) -> ()
                                n1789 = local write "VISA bus 0 error out hid"(w1339) -> ()
                                n1790 = local write "GPIB bus 0 write error"(w1343) -> ()
                                }
                                frame #4 {
                                n1791 = local write "SC handler states hid"(SC_handler_states."waiting on event" ("SC Test Interface States")) -> ()
                                }
                                }
                                }
                                }
                              }
                              frame "ECHONG" {
                                n1792 = flat-sequence {
                                frame #0 {
                                n1793 = local read "GPIB Bus 0 traffic"() -> (w1347:string)
                                n1794 = Concatenate Strings(w1347, "\r\n", "Bus 0: ECHONG received from tester" ("string")) -> (w1349:string)
                                n1795 = local write "GPIB Bus 0 traffic"(w1349) -> ()
                                }
                                frame #1 {
                                n1796 = local read "Last locked handler hid"() -> (w1351:enum16{"H1", "H2"})
                                n1797 = case shown="\"H2\"" w1351 {
                                frame "H1", Default {
                                w1352 = "ECHONG\n"
                                n1798 = local read "VISA bus 1 resource name out hid"() -> (w1360:refnum<visa-resource-name>)
                                n1799 = local read "VISA bus 1 error out hid"() -> (w1361:errorcluster)
                                n1800 = local read "GPIB bus 1 traffic"() -> (w1358:string)
                                n1801 = call <vilib>:"Trim Whitespace.vi"("string"=w1352) -> ("trimmed string"=w1353:string)  [unwired: 1 in]
                                n1802 = VISA Write(VISA resource name=w1360, write buffer=w1352, error in (no error)=w1361) -> (error out=w1354:errorcluster)  [unwired: 2 out]
                                n1803 = local write "VISA bus 1 error out hid"(w1354) -> ()
                                n1804 = Unbundle By Name(w1354) -> ("status"=w1359:bool)
                                n1805 = Concatenate Strings(w1358, "\r\n", "Bus 1 write: " ("string"), w1353) -> (w1356:string)
                                n1806 = local write "GPIB bus 1 write error"(w1359) -> ()
                                n1807 = local write "GPIB bus 1 traffic"(w1356) -> ()
                                }
                                frame "H2" {
                                w1362 = "ECHONG\n"
                                n1808 = local read "VISA bus 2 resource name out hid"() -> (w1370:refnum<visa-resource-name>)
                                n1809 = local read "VISA bus 2 error out hid"() -> (w1371:errorcluster)
                                n1810 = local read "GPIB bus 2 traffic"() -> (w1368:string)
                                n1811 = call <vilib>:"Trim Whitespace.vi"("string"=w1362) -> ("trimmed string"=w1363:string)  [unwired: 1 in]
                                n1812 = VISA Write(VISA resource name=w1370, write buffer=w1362, error in (no error)=w1371) -> (error out=w1364:errorcluster)  [unwired: 2 out]
                                n1813 = local write "VISA bus 2 error out hid"(w1364) -> ()
                                n1814 = Unbundle By Name(w1364) -> ("status"=w1369:bool)
                                n1815 = Concatenate Strings(w1368, "\r\n", "Bus 2 write: " ("string"), w1363) -> (w1366:string)
                                n1816 = local write "GPIB bus 2 write error"(w1369) -> ()
                                n1817 = local write "GPIB bus 2 traffic"(w1366) -> ()
                                }
                                }
                                }
                                frame #2 {
                                n1818 = local write "SC handler states hid"(SC_handler_states."waiting on event" ("SC Test Interface States")) -> ()
                                }
                                }
                              }
                              frame "ECHOOK" {
                                n1819 = flat-sequence {
                                frame #0 {
                                n1820 = local read "GPIB Bus 0 traffic"() -> (w1375:string)
                                n1821 = Concatenate Strings(w1375, "\r\n", "Bus 0: ECHOOK received from tester." ("string")) -> (w1377:string)
                                n1822 = local write "GPIB Bus 0 traffic"(w1377) -> ()
                                }
                                frame #1 {
                                n1823 = local read "Last locked handler hid"() -> (w1379:enum16{"H1", "H2"})
                                n1824 = case shown="\"H2\"" w1379 {
                                frame "H1", Default {
                                n1825 = while {
                                stop <- w1381 stop-if-true
                                w1383 = "ECHOOK\n"
                                n1826 = Wait (ms)(milliseconds to wait=u32 5) -> ()  [unwired: 1 out]
                                n1827 = local read "VISA bus 1 resource name out hid"() -> (w1391:refnum<visa-resource-name>)
                                n1828 = local read "VISA bus 1 error out hid"() -> (w1392:errorcluster)
                                n1829 = local read "GPIB bus 1 traffic"() -> (w1389:string)
                                n1830 = call <vilib>:"Trim Whitespace.vi"("string"=w1383) -> ("trimmed string"=w1384:string)  [unwired: 1 in]
                                n1831 = VISA Write(VISA resource name=w1391, write buffer=w1383, error in (no error)=w1392) -> (return count=w1380:u32, error out=w1385:errorcluster)  [unwired: 1 out]
                                n1832 = local write "VISA bus 1 error out hid"(w1385) -> ()
                                n1833 = Unbundle By Name(w1385) -> ("status"=w1390:bool)
                                n1834 = Greater Than 0?(x=w1380) -> (x > 0?=w1381:bool)
                                n1835 = Concatenate Strings(w1389, "\r\n", "Bus 1 write: " ("string"), w1384) -> (w1387:string)
                                n1836 = local write "GPIB bus 1 write error"(w1390) -> ()
                                n1837 = local write "GPIB bus 1 traffic"(w1387) -> ()
                                }
                                }
                                frame "H2" {
                                n1838 = while {
                                stop <- w1395 stop-if-true
                                w1396 = "ECHOOK\n"
                                n1839 = Wait (ms)(milliseconds to wait=u32 5) -> ()  [unwired: 1 out]
                                n1840 = local read "VISA bus 2 resource name out hid"() -> (w1404:refnum<visa-resource-name>)
                                n1841 = local read "VISA bus 2 error out hid"() -> (w1405:errorcluster)
                                n1842 = local read "GPIB bus 2 traffic"() -> (w1402:string)
                                n1843 = call <vilib>:"Trim Whitespace.vi"("string"=w1396) -> ("trimmed string"=w1397:string)  [unwired: 1 in]
                                n1844 = VISA Write(VISA resource name=w1404, write buffer=w1396, error in (no error)=w1405) -> (return count=w1394:u32, error out=w1398:errorcluster)  [unwired: 1 out]
                                n1845 = local write "VISA bus 2 error out hid"(w1398) -> ()
                                n1846 = Unbundle By Name(w1398) -> ("status"=w1403:bool)
                                n1847 = Greater Than 0?(x=w1394) -> (x > 0?=w1395:bool)
                                n1848 = Concatenate Strings(w1402, "\r\n", "Bus 2 write: " ("string"), w1397) -> (w1400:string)
                                n1849 = local write "GPIB bus 2 write error"(w1403) -> ()
                                n1850 = local write "GPIB bus 2 traffic"(w1400) -> ()
                                }
                                }
                                }
                                }
                                frame #2 {
                                n1851 = Tick Count (ms)() -> (millisecond timer value=w1406:u32)
                                n1852 = Tick Count (ms)() -> (millisecond timer value=w1407:u32)
                                n1853 = local write "tester wt start hid"(w1406) -> ()
                                n1854 = local write "tester tt end hid"(w1407) -> ()
                                }
                                frame #3 {
                                n1855 = local read "tester tt start hid"() -> (w1411:u32)
                                n1856 = local read "tester tt end hid"() -> (w1412:u32)
                                n1857 = Subtract(x=w1412, y=w1411) -> (x-y=w1410:u32)
                                n1858 = Divide(x=w1410, y=u32 1000) -> (x/y=w1408:dbl)
                                n1859 = local write "SC measured test time hid"(w1408) -> ()
                                }
                                frame #4 {
                                n1860 = local read "Last locked handler hid"() -> (w1413:enum16{"H1", "H2"})
                                n1861 = case shown="\"H1\", Default" w1413 {
                                frame "H1", Default {
                                n1862 = local read "H1 UPH"() -> (w1414:cluster{u32, u32})
                                n1863 = local read "H2 UPH"() -> (w1444:cluster{u32, u32})
                                n1864 = local read "Utilization (%)"() -> (w1425:u32)
                                n1865 = local read "Tandem\nfloorspace area"() -> (w1446:i32)
                                n1866 = local read "Std cell \nfloorspace area"() -> (w1439:i32)
                                n1867 = local read "Std hourly\ncost ($/hr)"() -> (w1442:dbl)
                                n1868 = local read "# of devices to test"() -> (w1431:u32)
                                n1869 = local read "Hours per month"() -> (w1426:i32)
                                n1870 = local read "Tandem hourly\ncost ($/hr)"() -> (w1443:dbl)
                                n1871 = Unbundle(w1414) -> (w1415:u32)  [unwired: 1 out]
                                n1872 = Unbundle(w1444) -> (w1421:u32)  [unwired: 1 out]
                                n1873 = local read "System UPH"() -> (w1445:u32)
                                n1874 = local read "H2 calc UPH"() -> (w1440:dbl)
                                n1875 = local write "Calc H1 UPH"(w1415) -> ()
                                n1876 = local write "Calc H2 UPH"(w1421) -> ()
                                n1877 = Add(x=w1415, y=w1421) -> (x+y=w1420:u32)
                                n1878 = Divide(x=w1425, y=u32 100) -> (x/y=w1424:dbl)
                                n1879 = local write "System UPH"(w1420) -> ()
                                n1880 = local write "Calc\nsystem UPH"(w1420) -> ()
                                n1881 = local read "UPH"() -> (w1441:dbl)
                                n1882 = Divide(x=w1445, y=w1446) -> (x/y=w1418:dbl)
                                n1883 = Divide(x=w1440, y=w1439) -> (x/y=w1419:dbl)
                                n1884 = Divide(x=w1431, y=w1420) -> (x/y=w1430:dbl)
                                n1885 = Multiply(x=w1426, y=w1424) -> (x*y=w1422:dbl)
                                n1886 = local write "Tandem UPH\nper unit area"(w1418) -> ()
                                n1887 = local write "H2 UPH per unit area"(w1419) -> ()
                                n1888 = Divide(x=w1442, y=w1441) -> (x/y=w1438:dbl)
                                n1889 = Divide(x=w1443, y=w1420) -> (x/y=w1436:dbl)
                                n1890 = Divide(x=w1430, y=w1422) -> (x/y=w1429:dbl)
                                n1891 = local read "# of devices to test"() -> (w1433:u32)
                                n1892 = Multiply(x=w1429, y=30) -> (x*y=w1427:dbl)
                                n1893 = Multiply(x=w1438, y=100.0) -> (x*y=w1417:dbl)
                                n1894 = Multiply(x=w1436, y=100.0) -> (x*y=w1416:dbl)
                                n1895 = local write "Tandem unit cost\n(cents/device)"(w1416) -> ()
                                n1896 = local write "Std unit cost\n(cents/device)"(w1417) -> ()
                                n1897 = local write "Calendar days required\nfor testing all units"(w1427) -> ()
                                n1898 = Subtract(x=w1417, y=w1416) -> (x-y=w1434:dbl)
                                n1899 = Multiply(x=w1433, y=w1434) -> (x*y=w1432:dbl)
                                n1900 = local write "$ saved"(w1432) -> ()
                                }
                                frame "H2" {
                                n1901 = local read "H1 UPH"() -> (w1476:cluster{u32, u32})
                                n1902 = local read "H2 UPH"() -> (w1447:cluster{u32, u32})
                                n1903 = local read "Utilization (%)"() -> (w1460:u32)
                                n1904 = local read "Tandem\nfloorspace area"() -> (w1450:i32)
                                n1905 = local read "Std cell \nfloorspace area"() -> (w1477:i32)
                                n1906 = local read "Std hourly\ncost ($/hr)"() -> (w1474:dbl)
                                n1907 = local read "# of devices to test"() -> (w1466:u32)
                                n1908 = local read "Hours per month"() -> (w1461:i32)
                                n1909 = local read "Tandem hourly\ncost ($/hr)"() -> (w1475:dbl)
                                n1910 = Unbundle(w1476) -> (w1468:u32)  [unwired: 1 out]
                                n1911 = Unbundle(w1447) -> (w1467:u32)  [unwired: 1 out]
                                n1912 = local read "System UPH"() -> (w1449:u32)
                                n1913 = local write "Calc H1 UPH"(w1468) -> ()
                                n1914 = local write "Calc H2 UPH"(w1467) -> ()
                                n1915 = Add(x=w1468, y=w1467) -> (x+y=w1456:u32)
                                n1916 = Divide(x=w1460, y=u32 100) -> (x/y=w1459:dbl)
                                n1917 = local read "UPH"() -> (w1478:dbl)
                                n1918 = local write "System UPH"(w1456) -> ()
                                n1919 = local write "Calc\nsystem UPH"(w1456) -> ()
                                n1920 = local read "UPH"() -> (w1473:dbl)
                                n1921 = Divide(x=w1449, y=w1450) -> (x/y=w1448:dbl)
                                n1922 = Divide(x=w1466, y=w1456) -> (x/y=w1465:dbl)
                                n1923 = Multiply(x=w1461, y=w1459) -> (x*y=w1457:dbl)
                                n1924 = local write "Tandem UPH\nper unit area"(w1448) -> ()
                                n1925 = Divide(x=w1478, y=w1477) -> (x/y=w1479:dbl)
                                n1926 = Divide(x=w1474, y=w1473) -> (x/y=w1472:dbl)
                                n1927 = Divide(x=w1475, y=w1456) -> (x/y=w1470:dbl)
                                n1928 = Divide(x=w1465, y=w1457) -> (x/y=w1464:dbl)
                                n1929 = local read "# of devices to test"() -> (w1454:u32)
                                n1930 = local write "H1 UPH per unit area"(w1479) -> ()
                                n1931 = Multiply(x=w1464, y=30) -> (x*y=w1462:dbl)
                                n1932 = Multiply(x=w1472, y=100.0) -> (x*y=w1452:dbl)
                                n1933 = Multiply(x=w1470, y=100.0) -> (x*y=w1451:dbl)
                                n1934 = local write "Tandem unit cost\n(cents/device)"(w1451) -> ()
                                n1935 = local write "Calendar days required\nfor testing all units"(w1462) -> ()
                                n1936 = local write "Std unit cost\n(cents/device)"(w1452) -> ()
                                n1937 = Subtract(x=w1452, y=w1451) -> (x-y=w1455:dbl)
                                n1938 = Multiply(x=w1454, y=w1455) -> (x*y=w1453:dbl)
                                n1939 = local write "$ saved"(w1453) -> ()
                                }
                                }
                                }
                                frame #5 {
                                n1940 = local read "Tester online"() -> (w1480:bool)
                                n1941 = local read "POWER"() -> (w1482:bool)
                                n1942 = Compound Arithmetic op=AND(w1480, w1482) -> (w1481:bool)
                                n1943 = case shown="True" w1481 {
                                frame False {
                                n1944 = local write "SC handler states hid"(SC_handler_states."closing bus" ("SC virtual handler states")) -> ()
                                }
                                frame True {
                                n1945 = flat-sequence {
                                frame #0 {
                                n1946 = local read "VISA bus 0 resource name out hid"() -> (w1486:refnum<visa-resource-name>)
                                n1947 = local read "VISA bus 0 error out hid"() -> (w1485:errorcluster)
                                n1948 = VISA Close(VISA resource name=w1486, error in (no error)=w1485) -> (error out=w1487:errorcluster)
                                n1949 = Unbundle By Name(w1487) -> ("status"=w1484:bool)
                                n1950 = local write "VISA bus 0 close error"(w1484) -> ()
                                }
                                frame #1 {
                                n1951 = local write "SC handler states hid"(SC_handler_states."initializing bus" ("SC Test Interface States")) -> ()
                                }
                                }
                                }
                                }
                                }
                                }
                              }
                              frame "closing bus" {
                                n1952 = flat-sequence {
                                frame #0 {
                                n1953 = local read "GPIB Bus 0 traffic"() -> (w1494:string)
                                n1954 = Concatenate Strings(w1494, "\r\n", "Bus 0 closing" ("string")) -> (w1492:string)
                                n1955 = local write "GPIB Bus 0 traffic"(w1492) -> ()
                                }
                                frame #1 {
                                n1956 = local read "VISA bus 0 resource name out hid"() -> (w1496:refnum<visa-resource-name>)
                                n1957 = local read "VISA bus 0 error out hid"() -> (w1497:errorcluster)
                                n1958 = VISA Close(VISA resource name=w1496, error in (no error)=w1497) -> (error out=w1495:errorcluster)
                                n1959 = Unbundle By Name(w1495) -> ("status"=w1498:bool)
                                n1960 = local write "VISA bus 0 close error"(w1498) -> ()
                                }
                                frame #2 {
                                n1961 = local write "Exit SC handler StMach hid"(TRUE ("Exit tester state machine hid")) -> ()
                                }
                                }
                              }
                              frame "responding to unknown command" {
                                n1962 = flat-sequence {
                                frame #0 {
                                n1963 = local read "GPIB Bus 0 traffic"() -> (w1506:string)
                                n1964 = Concatenate Strings(w1506, "\r\n", "Bus 0 write: " ("string"), "unrecognized string") -> (w1504:string)
                                n1965 = local write "GPIB Bus 0 traffic"(w1504) -> ()
                                }
                                frame #1 {
                                n1966 = local write "SC handler states hid"(SC_handler_states."waiting on event" ("SC Test Interface States")) -> ()
                                }
                                }
                              }
                            }
                          }
                          frame #1 {
                            n1967 = local read "Slow for  Diagnostics"() -> (w1508:bool)
                            n1968 = case shown="False" w1508 {
                              frame False {
                              }
                              frame True {
                                n1969 = local read "GPIB wait time (ms)"() -> (w1511:u32)
                                n1970 = Wait (ms)(milliseconds to wait=w1511) -> ()  [unwired: 1 out]
                              }
                            }
                          }
                        }
                        n1971 = Wait (ms)(milliseconds to wait=u32 5) -> ()  [unwired: 1 out]
                        n1972 = local read "Exit SC handler StMach hid"() -> (w725:bool)
                      }
                    }
                  }
                }
              }
              n1973 = Wait (ms)(milliseconds to wait=u32 5) -> ()  [unwired: 1 out]
              n1974 = local read "POWER"() -> (w712:bool)
            }
            n1975 = while {
              stop <- w360 continue-if-true
              n1976 = local read "H1 online"() -> (w361:bool)
              n1977 = case shown="True" w361 {
                frame False {
                }
                frame True {
                  n1978 = flat-sequence {
                    frame #0 {
                      n1979 = local write "Exit SC tester H1 StMach hid"(FALSE ("Exit H1 state machine hid")) -> ()
                    }
                    frame #1 {
                      n1980 = local write "NS6040 tester states H1 hid"(SC_NS6040_tester_states_v2."initializing bus" ("NS6040 tester states H1 hid")) -> ()
                      n1981 = while {
                        stop <- w365 stop-if-true
                        n1982 = Wait (ms)(milliseconds to wait=u32 5) -> ()  [unwired: 1 out]
                        n1983 = flat-sequence {
                          frame #0 {
                            n1984 = local read "NS6040 tester states H1 hid"() -> (w366:T3)
                            n1985 = case shown="\"serial polling handler\"" w366 {
                              frame "initializing bus", Default {
                                n1986 = flat-sequence {
                                frame #0 {
                                # "bus 1"
                                n1987 = local read "GPIB wait timeout hid"() -> (w370:u32)
                                n1988 = local read "SentCtrl talks to handler 1 at"() -> (w371:refnum<visa-resource-name>)
                                n1989 = local read "GPIB wait timeout hid"() -> (w369:u32)
                                n1990 = VISA Open(timeout (0)=w370, VISA resource name=w371) -> (VISA resource name=w368:refnum<visa-resource-name>, error out=w373:errorcluster)  [unwired: 3 in]
                                n1991 = property class="GPIB Instr"(reference=w368, error in=w373, "Timeout"=w369) -> (error out=w367:errorcluster)  [unwired: 1 out]
                                n1992 = local write "VISA bus 1 resource name out hid"(w368) -> ()
                                n1993 = Unbundle By Name(w367) -> ("status"=w372:bool)
                                n1994 = local write "VISA bus 1 open error"(w372) -> ()
                                n1995 = local write "VISA bus 1 error out hid"(w367) -> ()
                                }
                                frame #1 {
                                n1996 = local read "VISA bus 1 resource name out hid"() -> (w376:refnum<visa-resource-name>)
                                n1997 = local read "VISA bus 1 error out hid"() -> (w375:errorcluster)
                                n1998 = VISA Clear(VISA resource name=w376, error in (no error)=w375) -> (error out=w374:errorcluster)  [unwired: 1 out]
                                n1999 = local write "VISA bus 1 error out hid"(w374) -> ()
                                }
                                frame #2 {
                                n2000 = local write "Exit SC tester H1 StMach hid"(FALSE ("Exit H1 state machine hid")) -> ()
                                n2001 = Concatenate Strings("Bus 1 initializing" ("string"), "\r\n") -> (w379:string)
                                n2002 = local write "GPIB bus 1 traffic"(w379) -> ()
                                }
                                frame #3 {
                                n2003 = local write "NS6040 tester states H1 hid"(SC_NS6040_tester_states_v2."serial polling handler" ("NS6040 tester states H1 hid")) -> ()
                                }
                                }
                              }
                              frame "sending *IDN?" {
                                n2004 = flat-sequence {
                                tunnel: [w391] -> w384
                                tunnel: [w390] -> w383
                                tunnel: w384 -> [w405]
                                tunnel: w383 -> [w404]
                                tunnel: [w395] -> w382
                                tunnel: w382 -> [w406]
                                frame #0 {
                                w385 = "*IDN?\n"
                                # "It was discovered that his state is not initialized in application"
                                n2005 = local read "VISA bus 1 resource name out hid"() -> (w394:refnum<visa-resource-name>)
                                n2006 = local read "GPIB bus 1 traffic"() -> (w389:string)
                                n2007 = local read "VISA bus 1 error out hid"() -> (w393:errorcluster)
                                n2008 = Concatenate Strings(w389, "\r\n", "Bus 1 write: " ("string"), w385) -> (w387:string)
                                n2009 = VISA Write(VISA resource name=w394, write buffer=w385, error in (no error)=w393) -> (VISA resource name out=w391:refnum<visa-resource-name>, error out=w390:errorcluster)  [unwired: 1 out]
                                n2010 = Unbundle By Name(w390) -> ("status"=w392:bool)
                                n2011 = local write "GPIB bus 1 traffic"(w387) -> ()
                                n2012 = local write "GPIB bus 1 write error"(w392) -> ()
                                }
                                frame #1 {
                                n2013 = local read "GPIB bus 1 traffic"() -> (w397:string)
                                n2014 = VISA Read(VISA resource name=w405, byte count=u32 128, error in (no error)=w404) -> (VISA resource name out=w402:refnum<visa-resource-name>, read buffer=w396:string, error out=w401:errorcluster)  [unwired: 1 out]
                                n2015 = local write "VISA bus 1 resource name out hid"(w402) -> ()
                                n2016 = Unbundle By Name(w401) -> ("status"=w395:bool)
                                n2017 = local write "H1 response to *IDN? hid"(w396) -> ()
                                n2018 = local write "GPIB bus 1 read error"(w395) -> ()
                                n2019 = Concatenate Strings(w397, "\r\n", "Bus 1 read: " ("string"), w396) -> (w399:string)
                                n2020 = local write "GPIB bus 1 traffic"(w399) -> ()
                                }
                                frame #2 {
                                n2021 = case shown="True" w406 {
                                frame False {
                                n2022 = local write "NS6040 tester states H1 hid"(SC_NS6040_tester_states_v2."serial polling handler" ("NS6040 tester states H1 hid")) -> ()
                                }
                                frame True {
                                n2023 = flat-sequence {
                                frame #0 {
                                n2024 = while {
                                stop <- w409 stop-if-true
                                n2025 = One Button Dialog(message="Warning:\nVirtual tester does not get a response\nto *IDN? from handler 1.\nCheck GPIB cable and that  handler 1 \nis running and ready to issue a start of test\nby responding with sites ready.", button name ("OK")="Dismiss and retry") -> (true=w409:bool)
                                n2026 = Wait (ms)(milliseconds to wait=u32 100) -> ()  [unwired: 1 out]
                                }
                                }
                                frame #1 {
                                n2027 = local write "H1 online"(FALSE ("H1 online")) -> ()
                                }
                                frame #2 {
                                n2028 = local write "NS6040 tester states H1 hid"(SC_NS6040_tester_states_v2."sending *IDN?" ("NS6040 tester states H1 hid")) -> ()
                                }
                                }
                                }
                                }
                                }
                                }
                              }
                              frame "serial polling handler" {
                                n2029 = flat-sequence {
                                frame #0 {
                                n2030 = Concatenate Strings("Bus 1 read: " ("string"), "Serial polling handler 1") -> (w415:string)
                                n2031 = local write "GPIB bus 1 traffic"(w415) -> ()
                                }
                                frame #1 {
                                n2032 = local read "VISA bus 1 resource name out hid"() -> (w417:refnum<visa-resource-name>)
                                n2033 = local read "VISA bus 1 error out hid"() -> (w422:errorcluster)
                                n2034 = VISA Read STB(8:w422, 11:w417) -> (0:w423:errorcluster, 2:w420:u16)  [unwired: 1 out]
                                n2035 = Unbundle By Name(w423) -> ("status"=w421:bool)
                                n2036 = Equal?(x=w420, y=u16 65) -> (x = y?=w418:bool)
                                n2037 = case shown="False" w418 {
                                frame False {
                                n2038 = flat-sequence {
                                frame #0 {
                                n2039 = Wait (ms)(milliseconds to wait=u32 20) -> ()  [unwired: 1 out]
                                }
                                frame #1 {
                                n2040 = local write "NS6040 tester states H1 hid"(SC_NS6040_tester_states_v2."serial polling handler" ("NS6040 tester states H1 hid")) -> ()
                                }
                                }
                                }
                                frame True {
                                n2041 = flat-sequence {
                                frame #0 {
                                n2042 = local write "NS6040 tester states H1 hid"(SC_NS6040_tester_states_v2."sending Fullsites?" ("NS6040 tester states H1 hid")) -> ()
                                }
                                }
                                }
                                }
                                n2043 = local write "GPIB bus 1 write error"(w421) -> ()
                                }
                                }
                              }
                              frame "sending Fullsites?" {
                                n2044 = flat-sequence {
                                tunnel: [w438] -> w430
                                tunnel: [w437] -> w429
                                tunnel: [w442] -> w428
                                tunnel: w429 -> [w443]
                                tunnel: w430 -> [w444]
                                tunnel: w428 -> [w460]
                                tunnel: [w460] -> w427
                                tunnel: w427 -> [w461]
                                frame #0 {
                                w436 = "Fullsites?\n"
                                n2045 = local read "VISA bus 1 resource name out hid"() -> (w440:refnum<visa-resource-name>)
                                n2046 = local read "VISA bus 1 error out hid"() -> (w439:errorcluster)
                                n2047 = local read "GPIB bus 1 traffic"() -> (w432:string)
                                n2048 = call <vilib>:"Trim Whitespace.vi"("string"=w436) -> ("trimmed string"=w431:string)  [unwired: 1 in]
                                n2049 = VISA Write(VISA resource name=w440, write buffer=w436, error in (no error)=w439) -> (VISA resource name out=w437:refnum<visa-resource-name>, error out=w438:errorcluster)  [unwired: 1 out]
                                n2050 = Unbundle By Name(w438) -> ("status"=w441:bool)
                                n2051 = Concatenate Strings(w432, "\r\n", "Bus 1 write: " ("string"), w431) -> (w435:string)
                                n2052 = local write "GPIB bus 1 write error"(w441) -> ()
                                n2053 = local write "GPIB bus 1 traffic"(w435) -> ()
                                }
                                frame #1 {
                                n2054 = while {
                                tunnel: w444 -> [w453]
                                tunnel: w443 -> [w452]
                                tunnel: [w447] -> w442
                                stop <- w446 stop-if-true
                                n2055 = local read "GPIB bus 1 traffic"() -> (w458:string)
                                n2056 = VISA Read(VISA resource name=w452, byte count=u32 128, error in (no error)=w453) -> (read buffer=w447:string, error out=w450:errorcluster)  [unwired: 2 out]
                                n2057 = Unbundle By Name(w450) -> ("status"=w459:bool)
                                n2058 = call <vilib>:"Trim Whitespace.vi"("string"=w447) -> ("trimmed string"=w451:string)  [unwired: 1 in]
                                n2059 = Match True/False String(2:"X" ("false string"), 3:"Fullsites" ("true string"), 4:w447) -> (0:w446:bool)  [unwired: 1 out]
                                n2060 = local write "GPIB bus 1 read error"(w459) -> ()
                                n2061 = Concatenate Strings(w458, "\r\n", "Bus 1 read: " ("string"), w451) -> (w456:string)
                                n2062 = local write "GPIB bus 1 traffic"(w456) -> ()
                                n2063 = Wait (ms)(milliseconds to wait=u32 5) -> ()  [unwired: 1 out]
                                }
                                }
                                frame #2 {
                                n2064 = local write "H1 FULLSITES? response hid"(w460) -> ()
                                }
                                frame #3 {
                                w463 = "%032b"  # format string
                                n2065 = call <vilib>:"Space Constant.vi"() -> ("String"=w468:string)
                                n2066 = Concatenate Strings("Fullsites" ("regular expression"), w468) -> (w469:string)
                                n2067 = Match Pattern(string=w461, regular expression=w469) -> (after substring=w465:string)  [unwired: 1 in, 3 out]
                                n2068 = Hexadecimal String To Number(string=w465, default (0uL)=u64 0 ("default (0 U32)")) -> (number=w462:u64)  [unwired: 1 in, 1 out]
                                n2069 = Format Into String "Format Into String"(format string=w463, w462) -> (resulting string=w466:string)  [unwired: 2 in, 1 out]
                                n2070 = local write "H1 FULLSITES? binary hid"(w466) -> ()
                                }
                                frame #4 {
                                n2071 = flat-sequence {
                                frame #0 {
                                n2072 = local write "H1 Ready with sites hid"(TRUE ("H1 Ready with sites hid")) -> ()
                                n2073 = local write "H1 Testing"(FALSE ("h1 indexing")) -> ()
                                n2074 = local write "H1 Indexing"(FALSE ("h1 indexing")) -> ()
                                n2075 = local write "H1 Waiting"(TRUE ("H1 Ready with sites")) -> ()
                                }
                                frame #1 {
                                n2076 = Tick Count (ms)() -> (millisecond timer value=w474:u32)
                                n2077 = Tick Count (ms)() -> (millisecond timer value=w475:u32)
                                n2078 = local write "H1 wt start hidden"(w474) -> ()
                                n2079 = local write "H1 it end hidden"(w475) -> ()
                                }
                                frame #2 {
                                n2080 = local read "H1 it start hidden"() -> (w479:u32)
                                n2081 = local read "H1 it end hidden"() -> (w480:u32)
                                n2082 = Subtract(x=w480, y=w479) -> (x-y=w476:u32)
                                n2083 = Divide(x=w476, y=u32 1000) -> (x/y=w478:dbl)
                                n2084 = local write "H1 measured Index Time"(w478) -> ()
                                }
                                }
                                }
                                frame #5 {
                                n2085 = while {
                                stop <- w481 stop-if-true
                                n2086 = Wait (ms)(milliseconds to wait=u32 5) -> ()  [unwired: 1 out]
                                n2087 = local read "H1 Lock"() -> (w481:bool)
                                }
                                }
                                frame #6 {
                                n2088 = local write "NS6040 tester states H1 hid"(SC_NS6040_tester_states_v2."testing" ("NS6040 tester states H1 hid")) -> ()
                                }
                                }
                              }
                              frame "testing" {
                                n2089 = flat-sequence {
                                frame #0 {
                                n2090 = local read "GPIB bus 1 traffic"() -> (w487:string)
                                n2091 = Concatenate Strings(w487, "\r\n", "Bus 1: " ("string"), "testing" ("string")) -> (w485:string)
                                n2092 = local write "GPIB bus 1 traffic"(w485) -> ()
                                }
                                frame #1 {
                                n2093 = Tick Count (ms)() -> (millisecond timer value=w492:u32)
                                n2094 = Tick Count (ms)() -> (millisecond timer value=w493:u32)
                                n2095 = local write "H1 Indexing"(FALSE ("waiting")) -> ()
                                n2096 = local write "H1 Testing"(TRUE ("testing")) -> ()
                                n2097 = local write "H1 tt start hidden"(w492) -> ()
                                n2098 = local write "H1 wt end hidden"(w493) -> ()
                                n2099 = local write "H1 Waiting"(FALSE ("H1 Ready with sites")) -> ()
                                }
                                frame #2 {
                                n2100 = local read "H1 wt start hidden"() -> (w497:u32)
                                n2101 = local read "H1 wt end hidden"() -> (w498:u32)
                                n2102 = Subtract(x=w498, y=w497) -> (x-y=w496:u32)
                                n2103 = Divide(x=w496, y=u32 1000) -> (x/y=w494:dbl)
                                n2104 = local write "H1 measured Wait Time"(w494) -> ()
                                }
                                frame #3 {
                                n2105 = while {
                                stop <- w500 continue-if-true
                                n2106 = local read "H1 Lock"() -> (w500:bool)
                                n2107 = Wait (ms)(milliseconds to wait=u32 5) -> ()  [unwired: 1 out]
                                }
                                }
                                frame #4 {
                                n2108 = local write "H1 Ready with sites hid"(FALSE ("H1 Ready with siutes hid")) -> ()
                                n2109 = local write "NS6040 tester states H1 hid"(SC_NS6040_tester_states_v2."binning" ("NS6040 tester states H1 hid")) -> ()
                                }
                                }
                              }
                              frame "binning" {
                                n2110 = flat-sequence {
                                frame #0 {
                                n2111 = while {
                                stop <- w504 stop-if-true
                                n2112 = local read "SC handler states hid"() -> (w505:T6)
                                n2113 = Wait (ms)(milliseconds to wait=u32 5) -> ()  [unwired: 1 out]
                                n2114 = Equal?(x=w505, y=SC_handler_states."ECHOOK" ("SC Test Interface States")) -> (x = y?=w504:bool)
                                }
                                }
                                frame #1 {
                                n2115 = Tick Count (ms)() -> (millisecond timer value=w508:u32)
                                n2116 = Tick Count (ms)() -> (millisecond timer value=w507:u32)
                                n2117 = local write "H1 it start hidden"(w508) -> ()
                                n2118 = local write "H1 tt end hidden"(w507) -> ()
                                }
                                frame #2 {
                                n2119 = local read "GPIB bus 1 traffic"() -> (w512:string)
                                n2120 = Concatenate Strings(w512, "\r\n", "Bus 1: " ("string"), "binning" ("string")) -> (w510:string)
                                n2121 = local write "GPIB bus 1 traffic"(w510) -> ()
                                }
                                frame #3 {
                                n2122 = local write "H1 Waiting"(FALSE ("H1 Ready with sites")) -> ()
                                n2123 = local write "H1 Indexing"(TRUE ("waiting")) -> ()
                                n2124 = local write "H1 Testing"(FALSE ("testing")) -> ()
                                }
                                frame #4 {
                                n2125 = local read "H1 tt start hidden"() -> (w518:u32)
                                n2126 = local read "H1 tt end hidden"() -> (w519:u32)
                                n2127 = Subtract(x=w519, y=w518) -> (x-y=w520:u32)
                                n2128 = Divide(x=w520, y=u32 1000) -> (x/y=w517:dbl)
                                n2129 = local write "H1 measured Test Time"(w517) -> ()
                                }
                                frame #5 {
                                n2130 = local read "H1 binning string hid"() -> (w528:string)
                                n2131 = local read "H1 FULLSITES? binary hid"() -> (w527:string)
                                n2132 = String Subset(string=w528, offset (0)=6, length (rest)=35 ("length (rest)")) -> (substring=w534:string)
                                n2133 = local read "H1 Device Count"() -> (w525:u32)
                                n2134 = local read "H1 Good Units"() -> (w526:u32)
                                n2135 = Search and Replace String(replace all?=TRUE ("replace all? (F)"), input string=w534, search string=",") -> (result string=w540:string)  [unwired: 5 in, 3 out]
                                n2136 = Search and Replace String(replace all?=TRUE ("replace all? (F)"), input string=w527, search string="1") -> (number of replacements=w531:i32)  [unwired: 5 in, 3 out]
                                n2137 = Add(x=w531, y=w525) -> (x+y=w523:u32)
                                n2138 = Divide(x=w526, y=w525) -> (x/y=w541:dbl)
                                n2139 = Search and Replace String(replace all?=TRUE ("replace all? (F)"), input string=w540, search string="1") -> (number of replacements=w539:i32)  [unwired: 5 in, 3 out]
                                n2140 = local write "H1 Device Count"(w523) -> ()
                                n2141 = Add(x=w539, y=w526) -> (x+y=w524:u32)
                                n2142 = Multiply(x=w541, y=100.0) -> (x*y=w522:dbl)
                                n2143 = local write "H1 Good Units"(w524) -> ()
                                n2144 = local write "H1 cycle yield hid"(w522) -> ()
                                }
                                frame #6 {
                                n2145 = local read "H1 Device Count"() -> (w544:u32)
                                n2146 = local read "H1 Good Units"() -> (w545:u32)
                                n2147 = Divide(x=w545, y=w544) -> (x/y=w546:dbl)
                                n2148 = Multiply(x=w546, y=100.0) -> (x*y=w543:dbl)
                                n2149 = local write "H1 lot yield mon"(w543) -> ()
                                }
                                frame #7 {
                                n2150 = local read "H1 online"() -> (w548:bool)
                                n2151 = local read "POWER"() -> (w549:bool)
                                n2152 = Compound Arithmetic op=AND(w548, w549) -> (w550:bool)
                                n2153 = case shown="True" w550 {
                                frame False {
                                n2154 = local write "NS6040 tester states H1 hid"(SC_NS6040_tester_states_v2."closing bus" ("NS6040 tester states H1 hid")) -> ()
                                }
                                frame True {
                                n2155 = local write "NS6040 tester states H1 hid"(SC_NS6040_tester_states_v2."serial polling handler" ("NS6040 tester states H1 hid")) -> ()
                                }
                                }
                                }
                                }
                              }
                              frame "closing bus" {
                                n2156 = local read "GPIB bus 1 traffic"() -> (w557:string)
                                n2157 = local write "Exit SC tester H1 StMach hid"(TRUE ("Exit H1 state machine hid")) -> ()
                                n2158 = local read "VISA bus 1 resource name out hid"() -> (w561:refnum<visa-resource-name>)
                                n2159 = local read "VISA bus 1 error out hid"() -> (w560:errorcluster)
                                n2160 = Concatenate Strings(w557, "\r\n", "Bus 1: closing " ("string")) -> (w555:string)
                                n2161 = local write "GPIB bus 1 traffic"(w555) -> ()
                                n2162 = VISA Close(VISA resource name=w561, error in (no error)=w560) -> (error out=w559:errorcluster)
                                n2163 = Unbundle By Name(w559) -> ("status"=w558:bool)
                                n2164 = local write "VISA bus 1 close error"(w558) -> ()
                              }
                            }
                          }
                          frame #1 {
                            n2165 = local read "Slow for  Diagnostics"() -> (w562:bool)
                            n2166 = case shown="False" w562 {
                              frame False {
                              }
                              frame True {
                                n2167 = local read "GPIB wait time (ms)"() -> (w563:u32)
                                n2168 = Wait (ms)(milliseconds to wait=w563) -> ()  [unwired: 1 out]
                              }
                            }
                          }
                        }
                        n2169 = local read "Exit SC tester H1 StMach hid"() -> (w365:bool)
                      }
                    }
                  }
                }
              }
              n2170 = local read "POWER"() -> (w360:bool)
            }
            n2171 = while {
              stop <- w1512 continue-if-true
              n2172 = local read "H2 online"() -> (w1513:bool)
              n2173 = case shown="True" w1513 {
                frame False {
                }
                frame True {
                  n2174 = flat-sequence {
                    frame #0 {
                      n2175 = local write "Exit SC tester H2 StMach hid"(FALSE ("Exit H2 state machine hid")) -> ()
                    }
                    frame #1 {
                      n2176 = local write "NS6040 tester states H2 hid"(SC_NS6040_tester_states_v2."initializing bus" ("NS6040 tester states H1 hid")) -> ()
                      n2177 = while {
                        stop <- w1517 stop-if-true
                        n2178 = Wait (ms)(milliseconds to wait=u32 5) -> ()  [unwired: 1 out]
                        n2179 = flat-sequence {
                          frame #0 {
                            n2180 = local read "NS6040 tester states H2 hid"() -> (w1518:T3)
                            n2181 = case shown="\"serial polling handler\"" w1518 {
                              frame "initializing bus", Default {
                                n2182 = flat-sequence {
                                frame #0 {
                                # "bus 2"
                                n2183 = local read "GPIB wait timeout hid"() -> (w1521:u32)
                                n2184 = local read "SentCtrl talks to handler 2 at"() -> (w1523:refnum<visa-resource-name>)
                                n2185 = local read "GPIB wait timeout hid"() -> (w1522:u32)
                                n2186 = VISA Open(timeout (0)=w1521, VISA resource name=w1523) -> (VISA resource name=w1520:refnum<visa-resource-name>, error out=w1525:errorcluster)  [unwired: 3 in]
                                n2187 = property class="GPIB Instr"(reference=w1520, error in=w1525, "Timeout"=w1522) -> (error out=w1519:errorcluster)  [unwired: 1 out]
                                n2188 = local write "VISA bus 2 resource name out hid"(w1520) -> ()
                                n2189 = Unbundle By Name(w1519) -> ("status"=w1524:bool)
                                n2190 = local write "VISA bus 2 error out hid"(w1519) -> ()
                                n2191 = local write "VISA bus 2 open error"(w1524) -> ()
                                }
                                frame #1 {
                                n2192 = local read "VISA bus 2 resource name out hid"() -> (w1528:refnum<visa-resource-name>)
                                n2193 = local read "VISA bus 2 error out hid"() -> (w1527:errorcluster)
                                n2194 = VISA Clear(VISA resource name=w1528, error in (no error)=w1527) -> (error out=w1526:errorcluster)  [unwired: 1 out]
                                n2195 = local write "VISA bus 2 error out hid"(w1526) -> ()
                                }
                                frame #2 {
                                n2196 = local write "Exit SC tester H2 StMach hid"(FALSE ("Exit H2 state machine hid")) -> ()
                                n2197 = Concatenate Strings("Bus 2 initializing" ("string"), "\r\n") -> (w1531:string)
                                n2198 = local write "GPIB bus 2 traffic"(w1531) -> ()
                                }
                                frame #3 {
                                n2199 = local write "NS6040 tester states H2 hid"(SC_NS6040_tester_states_v2."serial polling handler" ("NS6040 tester states H2 hid")) -> ()
                                }
                                }
                              }
                              frame "sending *IDN?" {
                                n2200 = flat-sequence {
                                tunnel: [w1543] -> w1536
                                tunnel: [w1542] -> w1535
                                tunnel: w1536 -> [w1557]
                                tunnel: w1535 -> [w1556]
                                tunnel: [w1547] -> w1534
                                tunnel: w1534 -> [w1558]
                                frame #0 {
                                w1537 = "*IDN?"
                                # "It was discovered that his state is not initialized in application"
                                n2201 = local read "VISA bus 2 resource name out hid"() -> (w1546:refnum<visa-resource-name>)
                                n2202 = local read "GPIB bus 2 traffic"() -> (w1541:string)
                                n2203 = local read "VISA bus 2 error out hid"() -> (w1545:errorcluster)
                                n2204 = Concatenate Strings(w1541, "\r\n", "Bus 2 write: " ("string"), w1537) -> (w1539:string)
                                n2205 = VISA Write(VISA resource name=w1546, write buffer=w1537, error in (no error)=w1545) -> (VISA resource name out=w1543:refnum<visa-resource-name>, error out=w1542:errorcluster)  [unwired: 1 out]
                                n2206 = local write "GPIB bus 2 traffic"(w1539) -> ()
                                n2207 = Unbundle By Name(w1542) -> ("status"=w1544:bool)
                                n2208 = local write "GPIB bus 2 write error"(w1544) -> ()
                                }
                                frame #1 {
                                n2209 = VISA Read(VISA resource name=w1557, byte count=u32 128, error in (no error)=w1556) -> (VISA resource name out=w1554:refnum<visa-resource-name>, read buffer=w1548:string, error out=w1553:errorcluster)  [unwired: 1 out]
                                n2210 = local read "GPIB bus 2 traffic"() -> (w1549:string)
                                n2211 = local write "VISA bus 2 resource name out hid"(w1554) -> ()
                                n2212 = Unbundle By Name(w1553) -> ("status"=w1547:bool)
                                n2213 = local write "H2 response to *IDN? hid"(w1548) -> ()
                                n2214 = local write "GPIB bus 2 read error"(w1547) -> ()
                                n2215 = Concatenate Strings(w1549, "\r\n", "Bus 2 read: " ("string"), w1548) -> (w1551:string)
                                n2216 = local write "GPIB bus 2 traffic"(w1551) -> ()
                                }
                                frame #2 {
                                n2217 = case shown="True" w1558 {
                                frame False {
                                n2218 = local write "NS6040 tester states H2 hid"(SC_NS6040_tester_states_v2."testing" ("NS6040 tester states H2 hid")) -> ()
                                }
                                frame True {
                                n2219 = flat-sequence {
                                frame #0 {
                                n2220 = while {
                                stop <- w1561 stop-if-true
                                n2221 = One Button Dialog(message="Warning:\nVirtual tester does not get a response\nto *IDN? from handler 2.\nCheck GPIB cable and that  handler 2 \nis running and ready to issue a start of test\nby responding with sites ready.", button name ("OK")="Dismiss and retry") -> (true=w1561:bool)
                                n2222 = Wait (ms)(milliseconds to wait=u32 100) -> ()  [unwired: 1 out]
                                }
                                }
                                frame #1 {
                                n2223 = local write "H2 online"(FALSE ("H2 online")) -> ()
                                }
                                frame #2 {
                                n2224 = local write "NS6040 tester states H2 hid"(SC_NS6040_tester_states_v2."serial polling handler" ("NS6040 tester states H2 hid")) -> ()
                                }
                                }
                                }
                                }
                                }
                                }
                              }
                              frame "serial polling handler" {
                                n2225 = flat-sequence {
                                frame #0 {
                                n2226 = Concatenate Strings("Bus 2 write: " ("string"), "Serial polling handler 2") -> (w1567:string)
                                n2227 = local write "GPIB bus 2 traffic"(w1567) -> ()
                                }
                                frame #1 {
                                n2228 = local read "VISA bus 2 resource name out hid"() -> (w1573:refnum<visa-resource-name>)
                                n2229 = local read "VISA bus 2 error out hid"() -> (w1574:errorcluster)
                                n2230 = VISA Read STB(8:w1574, 11:w1573) -> (0:w1575:errorcluster, 2:w1571:u16)  [unwired: 1 out]
                                n2231 = Unbundle By Name(w1575) -> ("status"=w1572:bool)
                                n2232 = Equal?(x=u16 65, y=w1571) -> (x = y?=w1569:bool)
                                n2233 = case shown="False" w1569 {
                                frame False {
                                n2234 = flat-sequence {
                                frame #0 {
                                n2235 = Wait (ms)(milliseconds to wait=u32 20) -> ()  [unwired: 1 out]
                                }
                                frame #1 {
                                n2236 = local write "NS6040 tester states H2 hid"(SC_NS6040_tester_states_v2."serial polling handler" ("NS6040 tester states H1 hid")) -> ()
                                }
                                }
                                }
                                frame True {
                                n2237 = flat-sequence {
                                frame #0 {
                                n2238 = local write "NS6040 tester states H1 hid"(SC_NS6040_tester_states_v2."sending Fullsites?" ("NS6040 tester states H1 hid")) -> ()
                                }
                                }
                                }
                                }
                                n2239 = local write "GPIB bus 2 write error"(w1572) -> ()
                                }
                                }
                              }
                              frame "sending Fullsites?" {
                                n2240 = flat-sequence {
                                tunnel: [w1590] -> w1582
                                tunnel: [w1589] -> w1581
                                tunnel: [w1594] -> w1580
                                tunnel: w1581 -> [w1595]
                                tunnel: w1582 -> [w1596]
                                tunnel: w1580 -> [w1612]
                                tunnel: [w1612] -> w1579
                                tunnel: w1579 -> [w1613]
                                frame #0 {
                                w1588 = "Fulllsites?\n"
                                n2241 = local read "VISA bus 2 resource name out hid"() -> (w1591:refnum<visa-resource-name>)
                                n2242 = local read "VISA bus 2 error out hid"() -> (w1592:errorcluster)
                                n2243 = local read "GPIB bus 2 traffic"() -> (w1587:string)
                                n2244 = call <vilib>:"Trim Whitespace.vi"("string"=w1588) -> ("trimmed string"=w1583:string)  [unwired: 1 in]
                                n2245 = VISA Write(VISA resource name=w1591, write buffer=w1588, error in (no error)=w1592) -> (VISA resource name out=w1590:refnum<visa-resource-name>, error out=w1589:errorcluster)  [unwired: 1 out]
                                n2246 = local write "GPIB bus 2 traffic"(w1583) -> ()
                                n2247 = Unbundle By Name(w1589) -> ("status"=w1593:bool)
                                n2248 = Concatenate Strings(w1587, "\r\n", "Bus 2 write: " ("string"), w1583) -> (w1584:string)
                                n2249 = local write "GPIB bus 2 write error"(w1593) -> ()
                                n2250 = local write "GPIB bus 2 traffic"(w1584) -> ()
                                }
                                frame #1 {
                                n2251 = while {
                                tunnel: w1596 -> [w1605]
                                tunnel: w1595 -> [w1604]
                                tunnel: [w1600] -> w1594
                                stop <- w1597 stop-if-true
                                n2252 = local read "GPIB bus 2 traffic"() -> (w1610:string)
                                n2253 = VISA Read(VISA resource name=w1605, byte count=u32 128, error in (no error)=w1604) -> (read buffer=w1600:string, error out=w1602:errorcluster)  [unwired: 2 out]
                                n2254 = Unbundle By Name(w1602) -> ("status"=w1611:bool)
                                n2255 = call <vilib>:"Trim Whitespace.vi"("string"=w1600) -> ("trimmed string"=w1603:string)  [unwired: 1 in]
                                n2256 = Match True/False String(2:"X" ("false string"), 3:"Fullsites" ("true string"), 4:w1600) -> (0:w1597:bool)  [unwired: 1 out]
                                n2257 = local write "GPIB bus 2 read error"(w1611) -> ()
                                n2258 = Concatenate Strings(w1610, "\r\n", "Bus 2 read: " ("string"), w1603) -> (w1609:string)
                                n2259 = local write "GPIB bus 2 traffic"(w1609) -> ()
                                n2260 = Wait (ms)(milliseconds to wait=u32 5) -> ()  [unwired: 1 out]
                                }
                                }
                                frame #2 {
                                n2261 = local write "H2 FULLSITES? response hid"(w1612) -> ()
                                }
                                frame #3 {
                                w1615 = "%032b"  # format string
                                n2262 = call <vilib>:"Space Constant.vi"() -> ("String"=w1620:string)
                                n2263 = Concatenate Strings("Fullsites" ("regular expression"), w1620) -> (w1621:string)
                                n2264 = Match Pattern(string=w1613, regular expression=w1621) -> (after substring=w1617:string)  [unwired: 1 in, 3 out]
                                n2265 = Hexadecimal String To Number(string=w1617, default (0uL)=u64 0 ("default (0 U32)")) -> (number=w1614:u64)  [unwired: 1 in, 1 out]
                                n2266 = Format Into String "Format Into String"(format string=w1615, w1614) -> (resulting string=w1618:string)  [unwired: 2 in, 1 out]
                                n2267 = local write "H2 FULLSITES? binary hid"(w1618) -> ()
                                }
                                frame #4 {
                                n2268 = flat-sequence {
                                frame #0 {
                                n2269 = local write "H2 Ready with sites hid"(TRUE ("H2 Waiting")) -> ()
                                n2270 = local write "H2 Testing"(FALSE ("h1 indexing")) -> ()
                                n2271 = local write "H2 Indexing"(FALSE ("h1 indexing")) -> ()
                                n2272 = local write "H2 Waiting"(TRUE ("H2 Waiting")) -> ()
                                }
                                frame #1 {
                                n2273 = Tick Count (ms)() -> (millisecond timer value=w1626:u32)
                                n2274 = Tick Count (ms)() -> (millisecond timer value=w1627:u32)
                                n2275 = local write "H2 it end hidden"(w1626) -> ()
                                n2276 = local write "H2 wt start hidden"(w1627) -> ()
                                }
                                frame #2 {
                                n2277 = local read "H2 it start hidden"() -> (w1631:u32)
                                n2278 = local read "H2 it end hidden"() -> (w1632:u32)
                                n2279 = Subtract(x=w1632, y=w1631) -> (x-y=w1628:u32)
                                n2280 = Divide(x=w1628, y=u32 1000) -> (x/y=w1630:dbl)
                                n2281 = local write "H2 measured  Index Time"(w1630) -> ()
                                }
                                }
                                }
                                frame #5 {
                                n2282 = while {
                                stop <- w1633 stop-if-true
                                n2283 = local read "H2 Lock"() -> (w1633:bool)
                                n2284 = Wait (ms)(milliseconds to wait=u32 5) -> ()  [unwired: 1 out]
                                }
                                }
                                frame #6 {
                                n2285 = local write "NS6040 tester states H2 hid"(SC_NS6040_tester_states_v2."testing" ("NS6040 tester states H1 hid")) -> ()
                                }
                                }
                              }
                              frame "testing" {
                                n2286 = flat-sequence {
                                frame #0 {
                                n2287 = local read "GPIB bus 2 traffic"() -> (w1639:string)
                                n2288 = Concatenate Strings(w1639, "\r\n", "Bus 2: " ("string"), "testing" ("string")) -> (w1637:string)
                                n2289 = local write "GPIB bus 2 traffic"(w1637) -> ()
                                }
                                frame #1 {
                                n2290 = Tick Count (ms)() -> (millisecond timer value=w1644:u32)
                                n2291 = Tick Count (ms)() -> (millisecond timer value=w1645:u32)
                                n2292 = local write "H2 tt start hidden"(w1644) -> ()
                                n2293 = local write "H2 wt end hidden"(w1645) -> ()
                                n2294 = local write "H2 Indexing"(FALSE ("waiting")) -> ()
                                n2295 = local write "H2 Testing"(TRUE ("testing")) -> ()
                                n2296 = local write "H2 Waiting"(FALSE ("waiting")) -> ()
                                }
                                frame #2 {
                                n2297 = local read "H2 wt start hidden"() -> (w1647:u32)
                                n2298 = local read "H2 wt end hidden"() -> (w1646:u32)
                                n2299 = Subtract(x=w1646, y=w1647) -> (x-y=w1650:u32)
                                n2300 = Divide(x=w1650, y=u32 1000) -> (x/y=w1648:dbl)
                                n2301 = local write "H2 measured Wait Time"(w1648) -> ()
                                }
                                frame #3 {
                                n2302 = while {
                                stop <- w1652 continue-if-true
                                n2303 = local read "H2 Lock"() -> (w1652:bool)
                                n2304 = Wait (ms)(milliseconds to wait=u32 5) -> ()  [unwired: 1 out]
                                }
                                }
                                frame #4 {
                                n2305 = local write "H2 Ready with sites hid"(FALSE ("H2 Waiting")) -> ()
                                n2306 = local write "NS6040 tester states H2 hid"(SC_NS6040_tester_states_v2."binning" ("NS6040 tester states H1 hid")) -> ()
                                }
                                }
                              }
                              frame "binning" {
                                n2307 = flat-sequence {
                                frame #0 {
                                n2308 = while {
                                stop <- w1656 stop-if-true
                                n2309 = local read "SC handler states hid"() -> (w1657:T6)
                                n2310 = Wait (ms)(milliseconds to wait=u32 5) -> ()  [unwired: 1 out]
                                n2311 = Equal?(x=w1657, y=SC_handler_states."ECHOOK" ("SC Test Interface States")) -> (x = y?=w1656:bool)
                                }
                                }
                                frame #1 {
                                n2312 = Tick Count (ms)() -> (millisecond timer value=w1660:u32)
                                n2313 = Tick Count (ms)() -> (millisecond timer value=w1659:u32)
                                n2314 = local write "H2 it start hidden"(w1660) -> ()
                                n2315 = local write "H2 tt end hidden"(w1659) -> ()
                                }
                                frame #2 {
                                n2316 = local read "GPIB bus 2 traffic"() -> (w1662:string)
                                n2317 = Concatenate Strings(w1662, "\r\n", "Bus2: " ("string"), "binning" ("string")) -> (w1664:string)
                                n2318 = local write "GPIB bus 2 traffic"(w1664) -> ()
                                }
                                frame #3 {
                                n2319 = local write "H2 Waiting"(FALSE ("waiting")) -> ()
                                n2320 = local write "H2 Indexing"(TRUE ("waiting")) -> ()
                                n2321 = local write "H2 Testing"(FALSE ("testing")) -> ()
                                }
                                frame #4 {
                                n2322 = local read "H2 tt start hidden"() -> (w1669:u32)
                                n2323 = local read "H2 tt end hidden"() -> (w1670:u32)
                                n2324 = Subtract(x=w1670, y=w1669) -> (x-y=w1672:u32)
                                n2325 = Divide(x=w1672, y=u32 1000) -> (x/y=w1671:dbl)
                                n2326 = local write "H2 measured Test Time"(w1671) -> ()
                                }
                                frame #5 {
                                n2327 = local read "H2 binning string hid"() -> (w1680:string)
                                n2328 = local read "H2 FULLSITES? binary hid"() -> (w1679:string)
                                n2329 = String Subset(string=w1680, offset (0)=6, length (rest)=35 ("length (rest)")) -> (substring=w1686:string)
                                n2330 = local read "H2 Device Count"() -> (w1677:u32)
                                n2331 = local read "H2 Good Units"() -> (w1678:u32)
                                n2332 = Search and Replace String(replace all?=TRUE ("replace all? (F)"), input string=w1686, search string=",") -> (result string=w1692:string)  [unwired: 5 in, 3 out]
                                n2333 = Search and Replace String(replace all?=TRUE ("replace all? (F)"), input string=w1679, search string="1") -> (number of replacements=w1683:i32)  [unwired: 5 in, 3 out]
                                n2334 = Add(x=w1683, y=w1677) -> (x+y=w1675:u32)
                                n2335 = Divide(x=w1678, y=w1677) -> (x/y=w1693:dbl)
                                n2336 = Search and Replace String(replace all?=TRUE ("replace all? (F)"), input string=w1692, search string="1") -> (number of replacements=w1691:i32)  [unwired: 5 in, 3 out]
                                n2337 = local write "H2 Device Count"(w1675) -> ()
                                n2338 = Add(x=w1691, y=w1678) -> (x+y=w1676:u32)
                                n2339 = Multiply(x=w1693, y=100.0) -> (x*y=w1674:dbl)
                                n2340 = local write "H2 Good Units"(w1676) -> ()
                                n2341 = local write "H2 cycle yield hid"(w1674) -> ()
                                }
                                frame #6 {
                                n2342 = local read "H2 Device Count"() -> (w1695:u32)
                                n2343 = local read "H2 Good Units"() -> (w1696:u32)
                                n2344 = Divide(x=w1696, y=w1695) -> (x/y=w1698:dbl)
                                n2345 = Multiply(x=w1698, y=100.0) -> (x*y=w1697:dbl)
                                n2346 = local write "H2 lot yield mon"(w1697) -> ()
                                }
                                frame #7 {
                                n2347 = local read "H2 online"() -> (w1700:bool)
                                n2348 = local read "POWER"() -> (w1701:bool)
                                n2349 = Compound Arithmetic op=AND(w1700, w1701) -> (w1702:bool)
                                n2350 = case shown="True" w1702 {
                                frame False {
                                n2351 = local write "NS6040 tester states H2 hid"(SC_NS6040_tester_states_v2."closing bus" ("NS6040 tester states H1 hid")) -> ()
                                }
                                frame True {
                                n2352 = local write "NS6040 tester states H2 hid"(SC_NS6040_tester_states_v2."serial polling handler" ("NS6040 tester states H1 hid")) -> ()
                                }
                                }
                                }
                                }
                              }
                              frame "closing bus" {
                                n2353 = local read "GPIB bus 2 traffic"() -> (w1709:string)
                                n2354 = local write "Exit SC tester H2 StMach hid"(TRUE ("Exit H2 state machine hid")) -> ()
                                n2355 = local read "VISA bus 2 resource name out hid"() -> (w1713:refnum<visa-resource-name>)
                                n2356 = local read "VISA bus 2 error out hid"() -> (w1712:errorcluster)
                                n2357 = Concatenate Strings(w1709, "\r\n", "Bus 2: closing " ("string")) -> (w1707:string)
                                n2358 = local write "GPIB bus 2 traffic"(w1707) -> ()
                                n2359 = VISA Close(VISA resource name=w1713, error in (no error)=w1712) -> (error out=w1711:errorcluster)
                                n2360 = Unbundle By Name(w1711) -> ("status"=w1710:bool)
                                n2361 = local write "VISA bus 2 close error"(w1710) -> ()
                              }
                            }
                          }
                          frame #1 {
                            n2362 = local read "Slow for  Diagnostics"() -> (w1714:bool)
                            n2363 = case shown="True" w1714 {
                              frame False {
                              }
                              frame True {
                                n2364 = local read "GPIB wait time (ms)"() -> (w1715:u32)
                                n2365 = Wait (ms)(milliseconds to wait=w1715) -> ()  [unwired: 1 out]
                              }
                            }
                          }
                        }
                        n2366 = local read "Exit SC tester H2 StMach hid"() -> (w1517:bool)
                      }
                    }
                  }
                }
              }
              n2367 = local read "POWER"() -> (w1512:bool)
            }
          }
        }
      }
    }
  }
